vi "Laser_MAIN.vi"() -> ()   [LabVIEW 2013]
doc: "Пограмма управления мишенью лазерного источника ионов."
uses:
  <vilib>/Utility/miscctls.llb/LVPositionTypeDef.ctl
  <vilib>/Utility/inputDevices.llb/closeMouse.vi
panel:
  out "Текущая мишень:":string
  out "Флаг резерв. сохр.":bool
  in  "Шаг \nручного \nсдвига":string(combo)="5" caption="Шаг"
  in  "RightButton":bool
  in  "LeftButton":bool
  in  "DownButton":bool
  in  "UpButton":bool
  in  "М3":T1
  out "Знак перех. dX М10":i8
  out "Выстрелов осталось M10":u16=3
  in  "М10":T1
  in  "выстрел X М10":u16 step=1
  in  "выстрел Y М10":u16 step=1
  out "Знак перех. dX М9":i8
  out "Выстрелов осталось M9":u16=3
  in  "М9":T1
  in  "выстрел X М9":u16 step=1
  in  "выстрел Y М9":u16 step=1
  out "Выстрелов осталось M8":u16=3
  out "Знак перех. dX М8":i8
  in  "М8":T1
  in  "выстрел X М8":u16 step=1
  in  "выстрел Y М8":u16 step=1
  out "Выстрелов осталось M7":u16=3
  out "Знак перех. dX М7":i8
  in  "М7":T1
  in  "выстрел X М7":u16 step=1
  in  "выстрел Y М7":u16 step=1
  out "Выстрелов осталось M6":u16=3
  out "Знак перех. dX М6":i8
  in  "М6":T1
  in  "выстрел X М6":u16 step=1
  in  "выстрел Y М6":u16 step=1
  out "Выстрелов осталось M5":u16=3
  in  "М2":T1
  in  "М5":T1
  out "Знак перех. dX М5":i8
  in  "выстрел Y М5":u16 step=1
  in  "выстрел X М5":u16 step=1
  in  "М4":T1
  out "Знак перех. dX М4":i8
  in  "выстрел Y М4":u16 step=1
  in  "выстрел X М4":u16 step=1
  out "Знак перех. dX М3":i8
  in  "выстрел Y М3":u16 step=1
  in  "выстрел X М3":u16 step=1
  out "Знак перех. dX М2":i8
  in  "выстрел Y М2":u16 step=1
  in  "выстрел X М2":u16 step=1
  in  "выстрел Y М1":u16 step=1
  in  "выстрел X М1":u16 step=1
  out "Знак перех. dX М1":i8
  in  "М1":T1
  out "Выстрелов осталось M4":u16=3
  out "Выстрелов осталось M3":u16=3
  out "Выстрелов осталось M2":u16=3
  out "Выстрелов осталось M1":u16=3
  out "Статус":bool=TRUE caption="Готов!"
  in  "Tab control":T2(tab)
  in  "Перемотка пленки":bool
  in  "Фокус --":bool
  in  "Фокус +":bool
  in  "Сбросить конфигурацию":bool
  in  "Шаг вперед":bool
  in  "XY лазера":bool caption="осталось: 1"
  in  "текущ. инфо":bool caption="4"
  out "флаг закрытия с сохр.":bool
  in  "Загрузить настройки":bool
  in  "Конфигурация сохранена":bool
  in  "Мишень 10":picture
  in  "Мишень 9":picture
  in  "Мишень 8":picture
  in  "Мишень 7":picture
  in  "Мишень 6":picture
  in  "Упр. звуком":bool
  in  "Мишень 5":picture
  in  "Мишень 4":picture
  in  "Мишень 3":picture
  in  "Добавить мишень":bool
  in  "Мишень 2":picture
  in  "Мишень 1":picture
  in  "Выстрелов до перемотки пленки":u16=100
  out "Осталось:":u16(slide)=3 scale=100.0..1.0
  out "id мишени":u16=1
  in  "Счетчик выстрелов:":u32
  in  "TCP read data":string
  out "Slide X axis":u8(slide) max=100 scale=0.0..100.0
  out "Slide Y axis":u8(slide) max=50 step=1
  in  "Снимок сохранен":bool
  out "con err":bool caption="Connect"
  in  "Выстрел по мишени!":u32
  out "Счетчик мишеней":u8=3
  out "Соединение с блоком":bool
  out "Флаг соединения с прибором":bool caption="Connect"
  in  "OpLog":string
  in  "порт":u16=10001
  in  "IP-адрес":string="172.16.21.200"
  in  "Disconnect":bool caption="Disconn"
  out "Соединение":bool
  in  "Connect":bool
  out "TCP error source":string
  in  "stop":bool
  out "code out":i32 format="%0.0f"
  out "read_error_indicator":bool
  in  "Connect 2":bool caption="Connect"
  in  "flag1":bool caption="Disconn"
  out "TCP con ID":refnum<k5>
  out "Текущая конфигурация:":path
  out "Con.err.text":bool caption="Ошибка соединения с блоком..."
  # "Ручное управление \nлазером в пределах \nвыбранной мишени"
  # "Шаг перехода по Y, мм"
  # "Доп. настройки"
  # "Файлы"
  # "Мишени"
  # "Задано:"
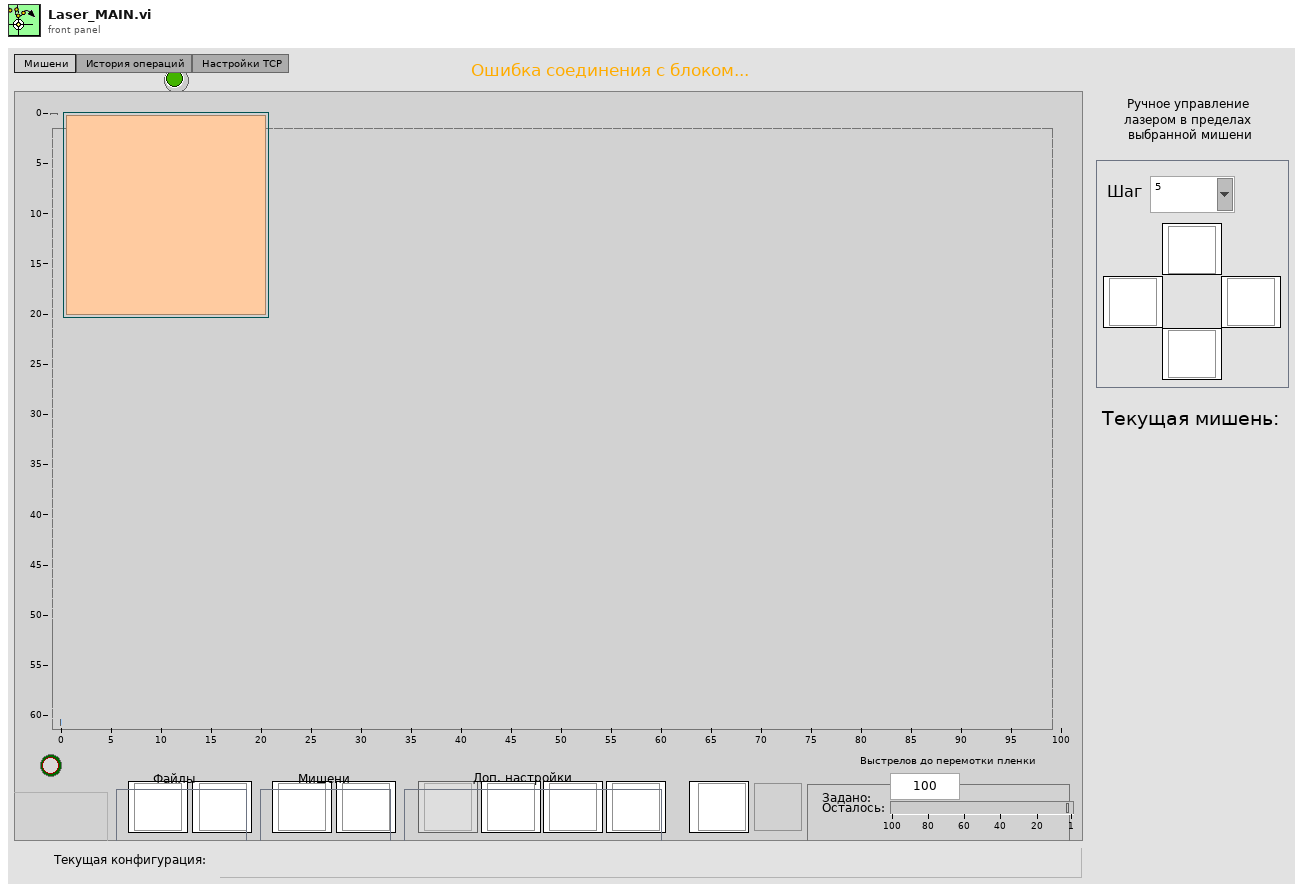
[diagram p1: front panel]
types:
  T1 = cluster{"Название мишени":string, "Х0_position":u16, "Y0_position":u16, "Длина, мм":u16, "Ширина, мм":u16, "Шаг перехода по горизонтали":dbl, "Шаг перехода по вертикали":dbl, "Выстрелов до перехода":u16, "Xo to send ":u16, "Yo to send":u16}
  T2 = enum32{" Мишени", " История операций", " Настройки TCP"}
  T3 = enum8{"Enabled", "Disabled", "Disabled and Grayed Out"}
  T4 = typedef "LVPositionTypeDef.ctl" = cluster{"Left":i32, "Top":i32}
  T5 = typedef "imagedata.ctl" = cluster{"image type":i32, "image depth":i32, "image":u8[], "mask":u8[], "colors":u32[], "Rectangle":cluster{"left":i16, "top":i16, "right":i16, "bottom":i16}}
  T6 = cluster{"id команды":u8, "№ мишени":u8, "Коорд. выстрела X ст.байт":u8, "Коорд. выстрела X мл.байт":u8, "Коорд. выстрела Y cт.байт":u8, "Коорд. выстрела Y мл.байт":u8, "Знак dX":i8, "выст. до перех. cт. байт":u8, "выст. до перех. мл. байт":u8, "выст. до перем. пленки ст. байт":u8, "выст. до перем. пленки мл. байт":u8}
  T7 = cluster{"номер мишени (id)":u8, u8, u8, u8, u8, u8, u8, u8, u8, u8, u8, u8, u8, u8, u8, u8, u8, u8, u8, u8}
  T8 = cluster{"доп команда":u8, u8, u8, u8, u8, u8, u8, u8, u8, u8, u8, u8, u8, u8, u8, u8, u8, u8, u8, u8}
  T9 = cluster{"М1":cluster{"Название мишени":string, "Х0_position":u16, "Y0_position":u16, "Длина, мм":u16, "Ширина, мм":u16, "Шаг перехода по горизонтали":dbl, "Шаг перехода по вертикали":dbl, "Выстрелов до перехода":u16, "Xo to send ":u16, "Yo to send":u16}, "М2":cluster{"Название мишени":string, "Х0_position":u16, "Y0_position":u16, "Длина, мм":u16, "Ширина, мм":u16, "Шаг перехода по горизонтали":dbl, "Шаг перехода по вертикали":dbl, "Выстрелов до перехода":u16, "Xo to send ":u16, "Yo to send":u16}, "М3":cluster{"Название мишени":string, "Х0_position":u16, "Y0_position":u16, "Длина, мм":u16, "Ширина, мм":u16, "Шаг перехода по горизонтали":dbl, "Шаг перехода по вертикали":dbl, "Выстрелов до перехода":u16, "Xo to send ":u16, "Yo to send":u16}, "М4":cluster{"Название мишени":string, "Х0_position":u16, "Y0_position":u16, "Длина, мм":u16, "Ширина, мм":u16, "Шаг перехода по горизонтали":dbl, "Шаг перехода по вертикали":dbl, "Выстрелов до перехода":u16, "Xo to send ":u16, "Yo to send":u16}, "М5":cluster{"Название мишени":string, "Х0_position":u16, "Y0_position":u16, "Длина, мм":u16, "Ширина, мм":u16, "Шаг перехода по горизонтали":dbl, "Шаг перехода по вертикали":dbl, "Выстрелов до перехода":u16, "Xo to send ":u16, "Yo to send":u16}, "М6":cluster{"Название мишени":string, "Х0_position":u16, "Y0_position":u16, "Длина, мм":u16, "Ширина, мм":u16, "Шаг перехода по горизонтали":dbl, "Шаг перехода по вертикали":dbl, "Выстрелов до перехода":u16, "Xo to send ":u16, "Yo to send":u16}, "М7":cluster{"Название мишени":string, "Х0_position":u16, "Y0_position":u16, "Длина, мм":u16, "Ширина, мм":u16, "Шаг перехода по горизонтали":dbl, "Шаг перехода по вертикали":dbl, "Выстрелов до перехода":u16, "Xo to send ":u16, "Yo to send":u16}, "М8":cluster{"Название мишени":string, "Х0_position":u16, "Y0_position":u16, "Длина, мм":u16, "Ширина, мм":u16, "Шаг перехода по горизонтали":dbl, "Шаг перехода по вертикали":dbl, "Выстрелов до перехода":u16, "Xo to send ":u16, "Yo to send":u16}, "М9":cluster{"Название мишени":string, "Х0_position":u16, "Y0_position":u16, "Длина, мм":u16, "Ширина, мм":u16, "Шаг перехода по горизонтали":dbl, "Шаг перехода по вертикали":dbl, "Выстрелов до перехода":u16, "Xo to send ":u16, "Yo to send":u16}, "М10":cluster{"Название мишени":string, "Х0_position":u16, "Y0_position":u16, "Длина, мм":u16, "Ширина, мм":u16, "Шаг перехода по горизонтали":dbl, "Шаг перехода по вертикали":dbl, "Выстрелов до перехода":u16, "Xo to send ":u16, "Yo to send":u16}}
  T10 = cluster{"выстрел X М1":u16, "выстрел Y М1":u16, "выстрел X М2":u16, "выстрел Y М2":u16, "выстрел X М3":u16, "выстрел Y М3":u16, "выстрел X М4":u16, "выстрел Y М4":u16, "выстрел X М5":u16, "выстрел Y М5":u16}
  T11 = cluster{"выстрел X М6":u16, "выстрел Y М6":u16, "выстрел X М7":u16, "выстрел Y М7":u16, "выстрел X М8":u16, "выстрел Y М8":u16, "выстрел X М9":u16, "выстрел Y М9":u16, "выстрел X М10":u16, "выстрел Y М10":u16}
  T12 = cluster{"Знак перех. dX М1":i8, "Знак перех. dX М2":i8, "Знак перех. dX М3":i8, "Знак перех. dX М4":i8, "Знак перех. dX М5":i8, "Знак перех. dX М6":i8, "Знак перех. dX М7":i8, "Знак перех. dX М8":i8, "Знак перех. dX М9":i8, "Знак перех. dX М10":i8}
  T13 = cluster{"Мишень 1":picture, "Мишень 2":picture, "Мишень 3":picture, "Мишень 4":picture, "Мишень 5":picture, "Мишень 6":picture, "Мишень 7":picture, "Мишень 8":picture, "Мишень 9":picture, "Мишень 10":picture}
  T14 = cluster{"Visible":bool, "Visible":bool, "Visible":bool, "Visible":bool, "Visible":bool, "Visible":bool, "Visible":bool, "Visible":bool, "Visible":bool, "Visible":bool}
  T15 = cluster{"Выстрелов осталось M1 ":u16, "Выстрелов осталось M2":u16, "Выстрелов осталось M3":u16, "Выстрелов осталось M4":u16, "Выстрелов осталось M5":u16, "Выстрелов осталось M6":u16, "Выстрелов осталось M7":u16, "Выстрелов осталось M8":u16, "Выстрелов осталось M9":u16, "Выстрелов осталось M10":u16}
  T16 = cluster{"Счетчик мишеней":u32, "Счетчик мишеней":u32}
  T17 = cluster{"Счетчик мишеней":i32, "Счетчик мишеней":i32}
  T18 = cluster{"Мишень 1":refnum<vi>, "Мишень 2":refnum<vi>, "Мишень 3":refnum<vi>, "Мишень 4":refnum<vi>, "Мишень 5":refnum<vi>, "Мишень 6":refnum<vi>, "Мишень 7":refnum<vi>, "Мишень 8":refnum<vi>, "Мишень 9":refnum<vi>, "Мишень 10":refnum<vi>}
  T19 = cluster{"Pict Refnum":refnum<vi>, "Pict Refnum 2":refnum<vi>, "Pict Refnum 3":refnum<vi>, "Pict Refnum 4":refnum<vi>, "Pict Refnum 5":refnum<vi>, "Pict Refnum 6":refnum<vi>, "Pict Refnum 7":refnum<vi>, "Pict Refnum 8":refnum<vi>, "Picture in Refnum 9":refnum<vi>, "Pict Refnum 10":refnum<vi>}
  T20 = cluster{"1":u16, "2":u16, "3":u16, "4":u16, "5":u16, "6":u16, "7":u16, "8":u16, "9":u16, "10":u16}
  T21 = cluster{"default value 1":i8, "default value 1":i8, "default value 1":i8, "default value 1":i8, "default value 1":i8, "default value 1":i8, "default value 1":i8, "default value 1":i8, "default value 1":i8, "default value 1":i8}
  T22 = cluster{"Кластер параметров мишени":cluster{"Название мишени":string, "Х0_position":u16, "Y0_position":u16, "Длина, мм":u16, "Ширина, мм":u16, "Шаг перехода по горизонтали":dbl, "Шаг перехода по вертикали":dbl, "Выстрелов до перехода":u16, "Xo to send ":u16, "Yo to send":u16}, "Кластер параметров мишени":cluster{"Название мишени":string, "Х0_position":u16, "Y0_position":u16, "Длина, мм":u16, "Ширина, мм":u16, "Шаг перехода по горизонтали":dbl, "Шаг перехода по вертикали":dbl, "Выстрелов до перехода":u16, "Xo to send ":u16, "Yo to send":u16}, "Кластер параметров мишени":cluster{"Название мишени":string, "Х0_position":u16, "Y0_position":u16, "Длина, мм":u16, "Ширина, мм":u16, "Шаг перехода по горизонтали":dbl, "Шаг перехода по вертикали":dbl, "Выстрелов до перехода":u16, "Xo to send ":u16, "Yo to send":u16}, "Кластер параметров мишени":cluster{"Название мишени":string, "Х0_position":u16, "Y0_position":u16, "Длина, мм":u16, "Ширина, мм":u16, "Шаг перехода по горизонтали":dbl, "Шаг перехода по вертикали":dbl, "Выстрелов до перехода":u16, "Xo to send ":u16, "Yo to send":u16}, "Кластер параметров мишени":cluster{"Название мишени":string, "Х0_position":u16, "Y0_position":u16, "Длина, мм":u16, "Ширина, мм":u16, "Шаг перехода по горизонтали":dbl, "Шаг перехода по вертикали":dbl, "Выстрелов до перехода":u16, "Xo to send ":u16, "Yo to send":u16}, "Кластер параметров мишени":cluster{"Название мишени":string, "Х0_position":u16, "Y0_position":u16, "Длина, мм":u16, "Ширина, мм":u16, "Шаг перехода по горизонтали":dbl, "Шаг перехода по вертикали":dbl, "Выстрелов до перехода":u16, "Xo to send ":u16, "Yo to send":u16}, "Кластер параметров мишени":cluster{"Название мишени":string, "Х0_position":u16, "Y0_position":u16, "Длина, мм":u16, "Ширина, мм":u16, "Шаг перехода по горизонтали":dbl, "Шаг перехода по вертикали":dbl, "Выстрелов до перехода":u16, "Xo to send ":u16, "Yo to send":u16}, "Кластер параметров мишени":cluster{"Название мишени":string, "Х0_position":u16, "Y0_position":u16, "Длина, мм":u16, "Ширина, мм":u16, "Шаг перехода по горизонтали":dbl, "Шаг перехода по вертикали":dbl, "Выстрелов до перехода":u16, "Xo to send ":u16, "Yo to send":u16}, "Кластер параметров мишени":cluster{"Название мишени":string, "Х0_position":u16, "Y0_position":u16, "Длина, мм":u16, "Ширина, мм":u16, "Шаг перехода по горизонтали":dbl, "Шаг перехода по вертикали":dbl, "Выстрелов до перехода":u16, "Xo to send ":u16, "Yo to send":u16}, "Кластер параметров мишени":cluster{"Название мишени":string, "Х0_position":u16, "Y0_position":u16, "Длина, мм":u16, "Ширина, мм":u16, "Шаг перехода по горизонтали":dbl, "Шаг перехода по вертикали":dbl, "Выстрелов до перехода":u16, "Xo to send ":u16, "Yo to send":u16}}
  T23 = enum16{"Left Button", "Center Button", "Right Button", "Window Close"}
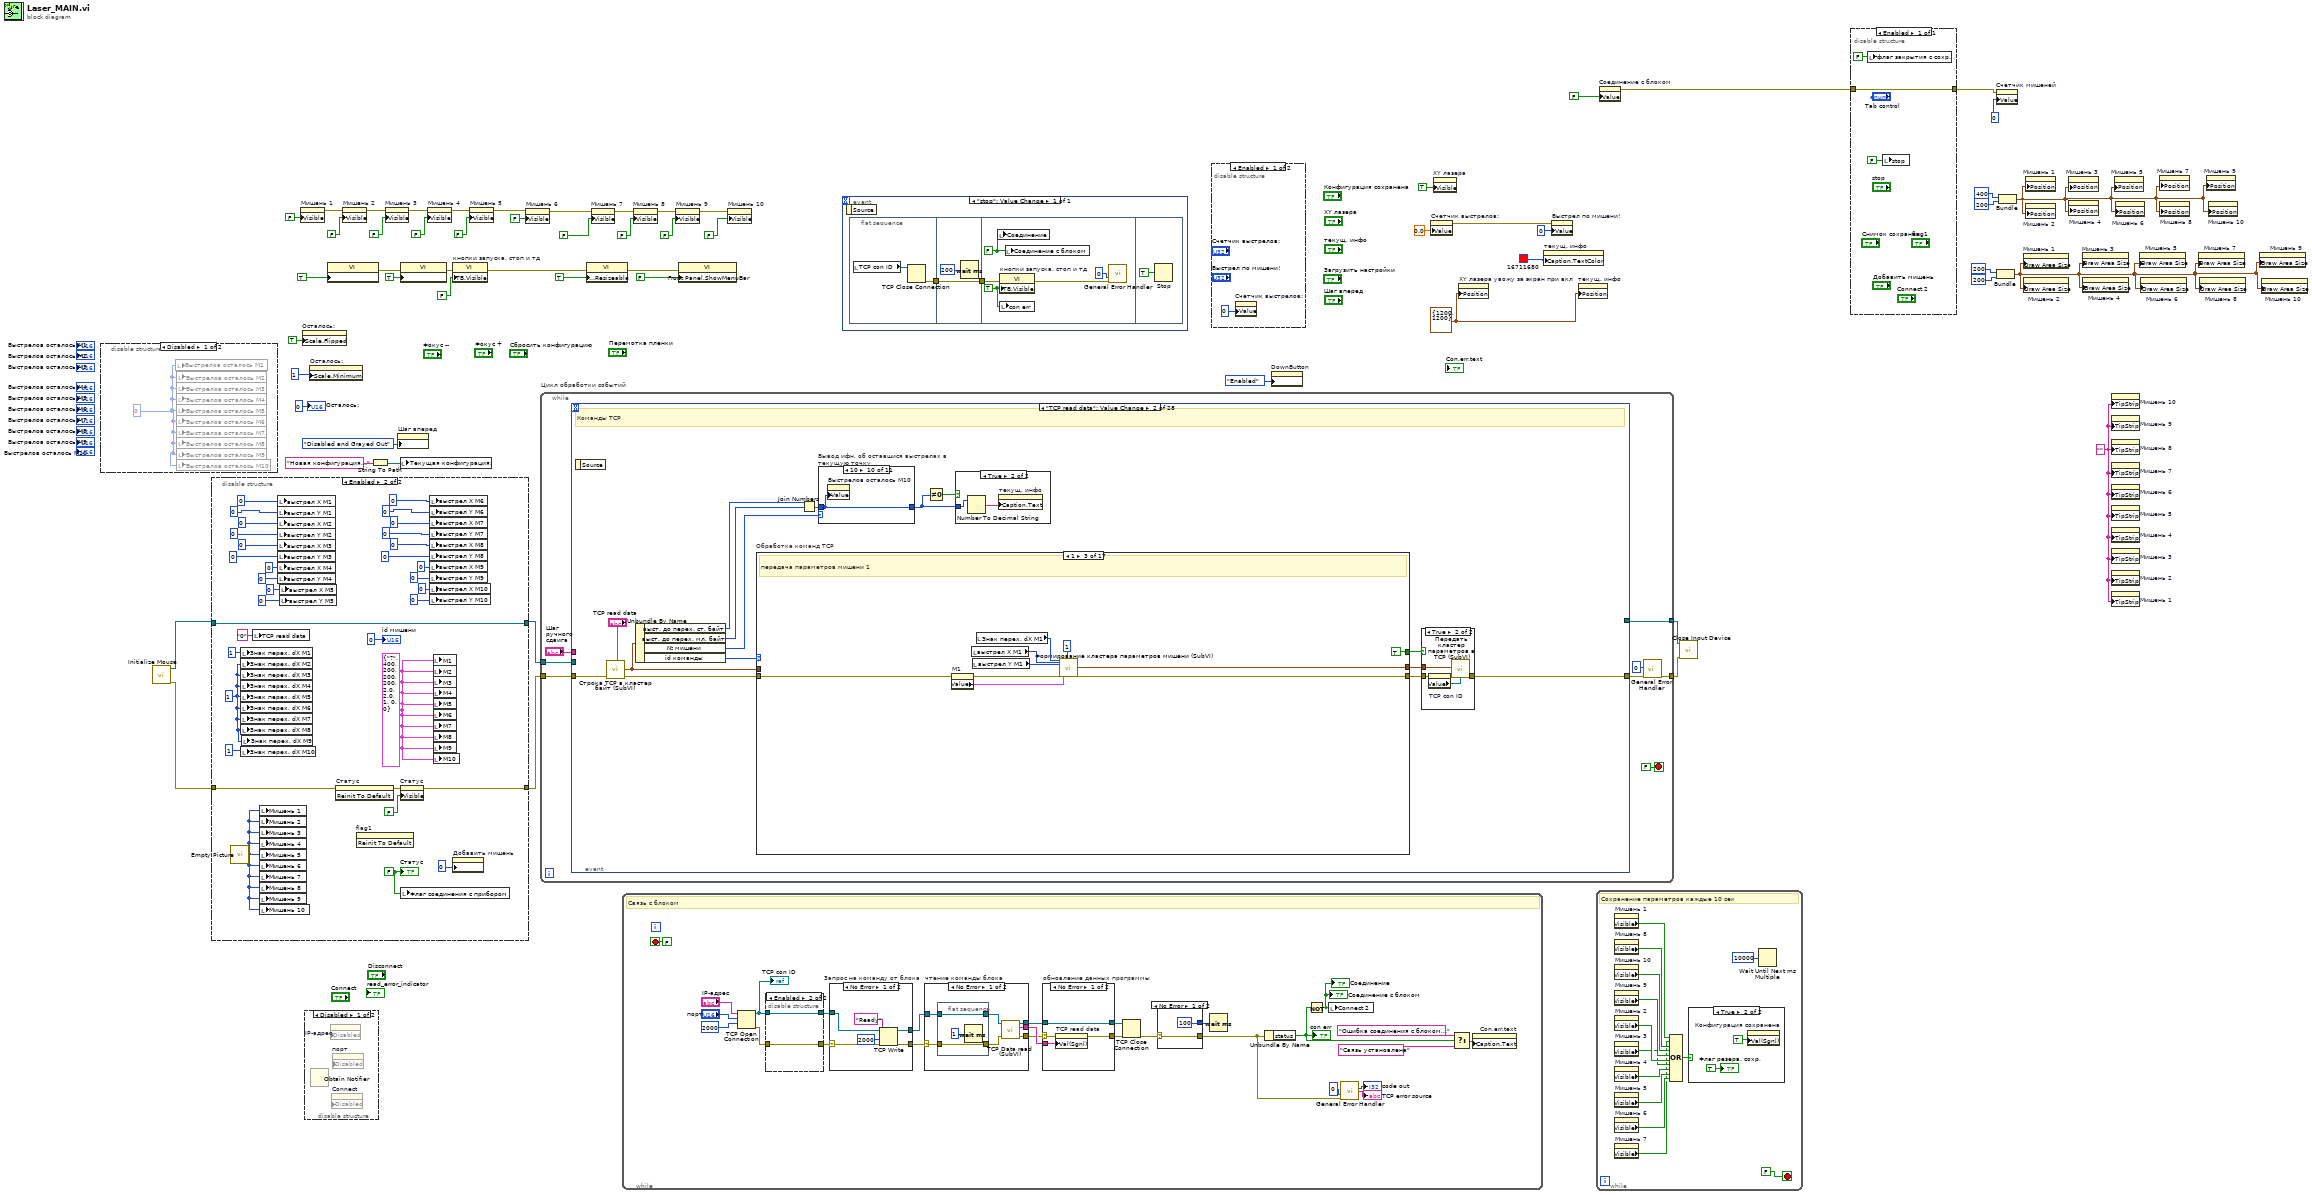
[diagram p0: block diagram]
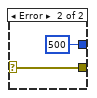
[diagram p5: hidden frame]
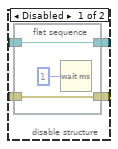
[diagram p6: hidden frame]
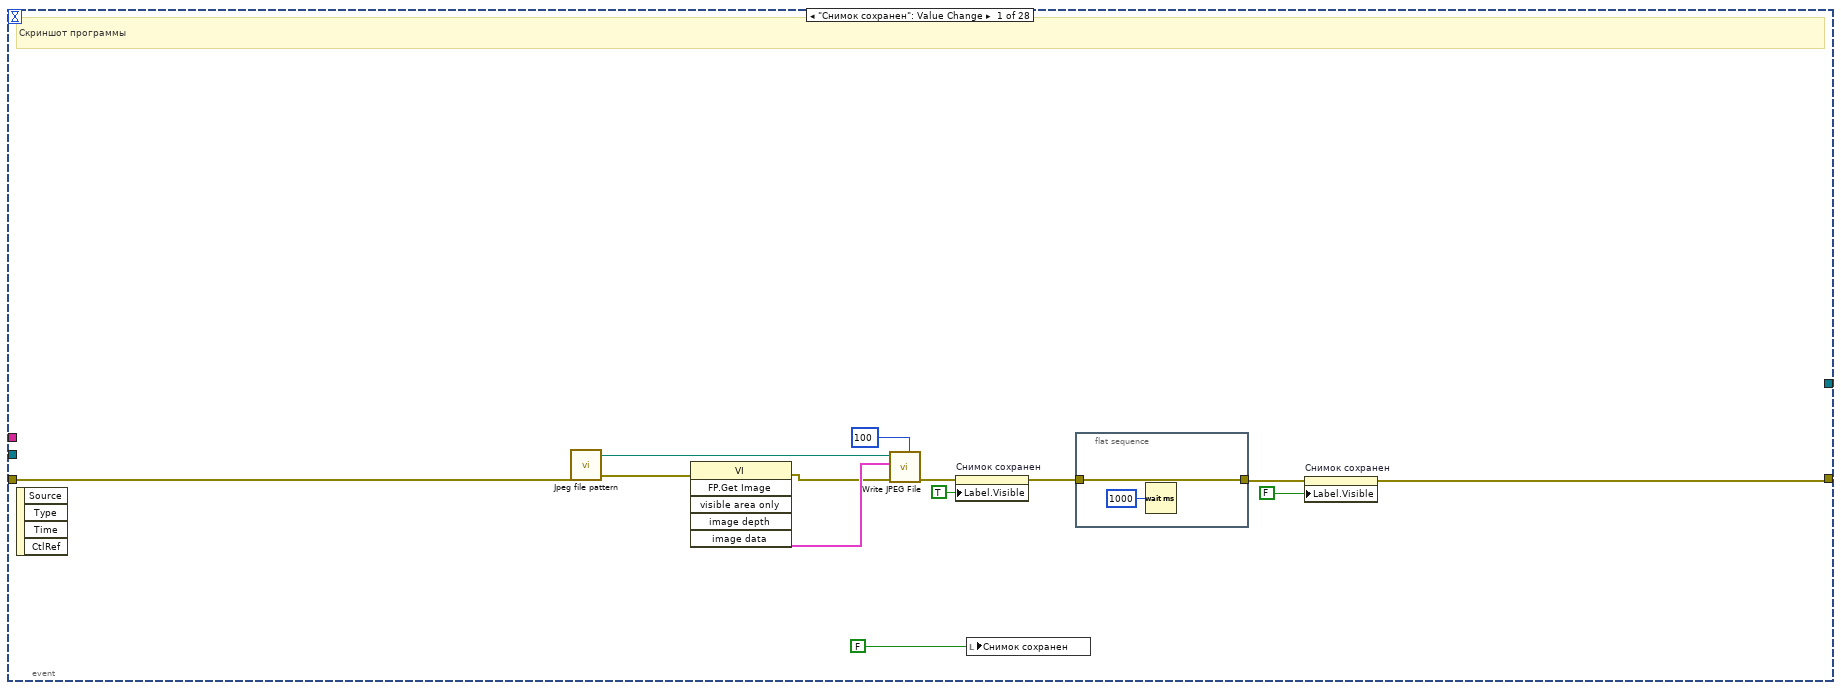
[diagram p12: hidden frame]
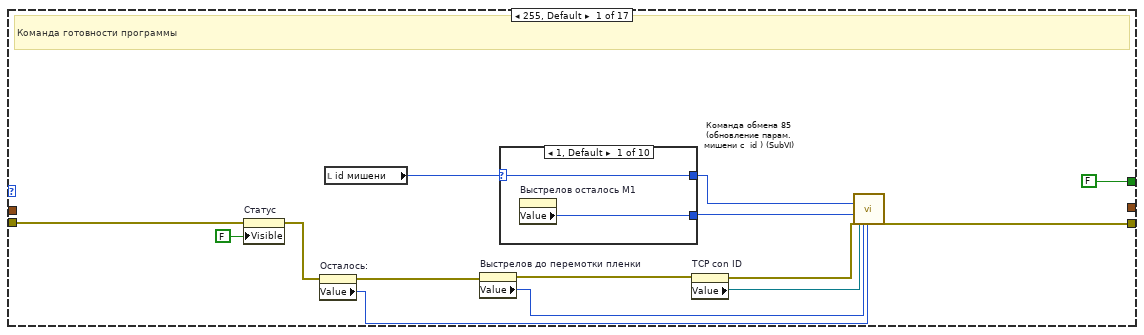
[diagram p15: hidden frame]
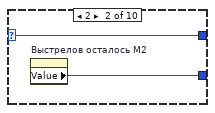
[diagram p16: hidden frame]
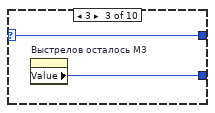
[diagram p17: hidden frame]
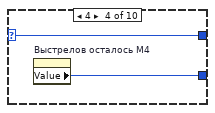
[diagram p18: hidden frame]
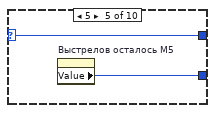
[diagram p19: hidden frame]
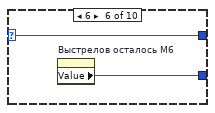
[diagram p20: hidden frame]
diagram:
  w8 = "" ("Tip Strip")
  w49 = T4 {"Left"=1200, "Top"=1200} ("Position")
  n1 = disable-structure shown="Disabled" {
    frame Disabled {
      w59 = u16 0
      n2 = local write "Выстрелов осталось M1"(w59) -> ()
      n3 = local write "Выстрелов осталось M2"(w59) -> ()
      n4 = local write "Выстрелов осталось M3"(w59) -> ()
      n5 = local write "Выстрелов осталось M4"(w59) -> ()
      n6 = local write "Выстрелов осталось M5"(w59) -> ()
      n7 = local write "Выстрелов осталось M6"(w59) -> ()
      n8 = local write "Выстрелов осталось M7"(w59) -> ()
      n9 = local write "Выстрелов осталось M8"(w59) -> ()
      n10 = local write "Выстрелов осталось M9"(w59) -> ()
      n11 = local write "Выстрелов осталось M10"(w59) -> ()
    }
    frame Enabled {
    }
  }
  n12 = call <vilib>:"Initialize Mouse.vi"() -> ("error out"=w51:errorcluster, "device ID"=w53:refnum<k1>)  [unwired: 1 in, 9 out]
  n13 = disable-structure shown="Enabled" {
    disable-tunnel: [_ w93] -> w54
    disable-tunnel: w53 -> [_ w93]
    disable-tunnel: [_ w64] -> w52
    disable-tunnel: w51 -> [_ w92]
    frame Disabled {
    }
    frame Enabled {
      w88 = i8 1 ("Выстрелов осталось M1")
      w89 = T1 {"Название мишени"="?", "Х0_position"=400, "Y0_position"=200, "Длина, мм"=200, "Ширина, мм"=200, "Шаг перехода по горизонтали"=2.0, "Шаг перехода по вертикали"=2.0, "Выстрелов до перехода"=1, "Xo to send "=0, "Yo to send"=0} ("Параметры М1")
      w61 = FALSE ("Готов")
      n14 = call "Empty Picture"() -> ("empty picture"=w65:picture)
      n15 = local write "Знак перех. dX М1"(i8 1 ("Знак перех. dX М1")) -> ()
      n16 = local write "Знак перех. dX М2"(w88) -> ()
      n17 = local write "Знак перех. dX М3"(w88) -> ()
      n18 = local write "Знак перех. dX М4"(w88) -> ()
      n19 = local write "Знак перех. dX М5"(w88) -> ()
      n20 = local write "Знак перех. dX М6"(w88) -> ()
      n21 = local write "Знак перех. dX М7"(w88) -> ()
      n22 = local write "Знак перех. dX М8"(w88) -> ()
      n23 = local write "Знак перех. dX М10"(i8 1 ("Выстрелов осталось M1")) -> ()
      n24 = local write "Знак перех. dX М9"(w88) -> ()
      n25 = local write "TCP read data"("0" ("TCP read data")) -> ()
      n26 = local write "Мишень 1"(w65) -> ()
      n27 = local write "Мишень 2"(w65) -> ()
      n28 = local write "Мишень 3"(w65) -> ()
      n29 = local write "Мишень 4"(w65) -> ()
      n30 = local write "Мишень 5"(w65) -> ()
      n31 = local write "Мишень 6"(w65) -> ()
      n32 = local write "Мишень 7"(w65) -> ()
      n33 = local write "Мишень 8"(w65) -> ()
      n34 = local write "Мишень 9"(w65) -> ()
      n35 = local write "Мишень 10"(w65) -> ()
      n36 = local write "выстрел X М1"(u16 0 ("Выстрелов осталось M1")) -> ()
      n37 = local write "выстрел Y М1"(u16 0 ("Выстрелов осталось M2")) -> ()
      n38 = local write "выстрел X М2"(u16 0 ("Выстрелов осталось M3")) -> ()
      n39 = local write "выстрел Y М2"(u16 0 ("Выстрелов осталось M4")) -> ()
      n40 = local write "выстрел X М3"(u16 0 ("Выстрелов осталось M5")) -> ()
      n41 = local write "выстрел Y М3"(u16 0 ("Выстрелов осталось M6")) -> ()
      n42 = local write "выстрел X М4"(u16 0 ("выстрел X М9")) -> ()
      n43 = local write "выстрел Y М4"(u16 0 ("выстрел Y М9")) -> ()
      n44 = local write "выстрел X М5"(u16 0 ("выстрел X М10")) -> ()
      n45 = local write "выстрел Y М5"(u16 0 ("выстрел Y М10")) -> ()
      n46 = invoke on="Статус" class="Bool (strict)" method="Reinit To Default"(error in=w92) -> (error out=w90:errorcluster)  [unwired: 2 in, 2 out]
      n47 = invoke on="flag1" class="Bool (strict)" method="Reinit To Default"() -> ()  [unwired: 3 in, 3 out]
      n48 = property on="Статус" class="Bool (strict)"(error in=w90, "Visible"=FALSE) -> (error out=w64:errorcluster)  [unwired: 1 in, 1 out]
      n49 = local write "Флаг соединения с прибором"(w61) -> ()
      n50 = local write "выстрел X М6"(u16 0 ("Выстрелов осталось M1")) -> ()
      n51 = local write "выстрел Y М6"(u16 0 ("Выстрелов осталось M2")) -> ()
      n52 = local write "выстрел X М7"(u16 0 ("Выстрелов осталось M3")) -> ()
      n53 = local write "выстрел Y М7"(u16 0 ("Выстрелов осталось M4")) -> ()
      n54 = local write "выстрел X М8"(u16 0 ("Выстрелов осталось M5")) -> ()
      n55 = local write "выстрел Y М8"(u16 0 ("Выстрелов осталось M6")) -> ()
      n56 = local write "выстрел X М9"(u16 0 ("выстрел X М9")) -> ()
      n57 = local write "выстрел Y М9"(u16 0 ("выстрел Y М9")) -> ()
      n58 = local write "выстрел X М10"(u16 0 ("выстрел X М10")) -> ()
      n59 = local write "выстрел Y М10"(u16 0 ("выстрел Y М10")) -> ()
      n60 = local write "М1"(w89) -> ()
      n61 = local write "М2"(w89) -> ()
      n62 = local write "М3"(w89) -> ()
      n63 = local write "М4"(w89) -> ()
      n64 = local write "М5"(w89) -> ()
      n65 = local write "М6"(w89) -> ()
      n66 = local write "М7"(w89) -> ()
      n67 = local write "М8"(w89) -> ()
      n68 = local write "М9"(w89) -> ()
      n69 = local write "М10"(w89) -> ()
      n70 = property on="Добавить мишень" class="Bool (strict)"("DisabledEnum"=i8 0 ("Выстрелов осталось M1")) -> ()  [unwired: 2 in, 2 out]
      "Статус" <- w61
      "id мишени" <- u16 0 ("id мишени")
    }
  }
  n71 = property on="Мишень 1" class="Pict"("Visible"=FALSE) -> (error out=w35:errorcluster)  [unwired: 2 in, 1 out]
  n72 = property on="Осталось:" class="Slide (strict)"("Scale.Flipped"=TRUE) -> ()  [unwired: 2 in, 2 out]
  n73 = disable-structure shown="Disabled" {
    frame Disabled {
      n74 = Obtain Notifier() -> ()  [unwired: 4 in, 3 out]
      n75 = property on="IP-адрес" class="Str" props=["Disabled"]() -> ()  [unwired: 3 in, 2 out]
      n76 = property on="Connect" class="Bool (strict)" props=["Disabled"]() -> ()  [unwired: 3 in, 2 out]
      n77 = property on="порт" class="DigNum (strict)" props=["Disabled"]() -> ()  [unwired: 3 in, 2 out]
    }
    frame Enabled {
    }
  }
  n78 = property on="Осталось:" class="Slide (strict)"("Scale.Minimum"=u16 1 ("До перемотки осталось")) -> ()  [unwired: 2 in, 2 out]
  n79 = property class="VI"("Front Panel.Minimizeable"=TRUE ("Front Panel Window:Minimizable")) -> (error out=w41:errorcluster)  [unwired: 2 in, 1 out]
  n80 = property on="Мишень 2" class="Pict"(error in=w35, "Visible"=FALSE) -> (error out=w32:errorcluster)  [unwired: 1 in, 1 out]
  n81 = String To Path(string="Новая конфигурация...") -> (path=w7:path)
  n82 = property on="Мишень 3" class="Pict"(error in=w32, "Visible"=FALSE) -> (error out=w30:errorcluster)  [unwired: 1 in, 1 out]
  n83 = property on="Шаг вперед" class="Bool (strict)"("DisabledEnum"=T3."Disabled and Grayed Out" ("Disabled")) -> ()  [unwired: 2 in, 2 out]
  n84 = property class="VI"(error in=w41, "Front Panel.TitleBarVis"=TRUE ("Front Panel Window:Title Bar Visible")) -> (error out=w40:errorcluster)  [unwired: 1 in, 1 out]
  n85 = local write "Текущая конфигурация:"(w7) -> ()
  n86 = property on="Мишень 4" class="Pict"(error in=w30, "Visible"=FALSE) -> (error out=w28:errorcluster)  [unwired: 1 in, 1 out]
  n87 = property on="кнопки запуска, стоп и тд" class="VI"(error in=w40, "TB.Visible"=FALSE ("Tool Bar:Visible")) -> (error out=w39:errorcluster)  [unwired: 1 in, 1 out]
  n88 = property on="Мишень 5" class="Pict"(error in=w28, "Visible"=FALSE) -> (error out=w16:errorcluster)  [unwired: 1 in, 1 out]
  n89 = property on="Мишень 6" class="Pict"(error in=w16, "Visible"=FALSE) -> (error out=w17:errorcluster)  [unwired: 1 in, 1 out]
  n90 = while "Цикл обработки событий" {
    tunnel: w52 -> [w100]
    tunnel: w54 -> [w99]
    tunnel: [w96] -> w50
    tunnel: [w95] -> w48
    stop <- FALSE stop-if-true
    n91 = event shown="[1] \"TCP read data\": Value Change" {
      selector: _ -> [_ _ _ _ _ _ _ _ _ _ _ _ _ _ _ _ _ _ _ _ _ _ _ _ _ _ _ _]
      dyn-events: _ -> [_ _ _ _ _ _ _ _ _ _ _ _ _ _ _ _ _ _ _ _ _ _ _ _ _ _ _ _]
      timeout: _ -> [_ _ _ _ _ _ _ _ _ _ _ _ _ _ _ _ _ _ _ _ _ _ _ _ _ _ _ _]
      tunnel: [w102 w131 w689 w801 w816 w851 w878 w904 w930 w956 w982 w1008 w1034 w1060 w1086 w1120 w1153 w1159 w1163 w1168 w1184 w1223 w1280 w1328 w1366 _ w1547 _] -> w97
      tunnel: w100 -> [w110 w130 w695 w805 w815 w852 w877 w903 w929 w955 w981 w1007 w1033 w1059 w1085 w1113 w1154 w1162 w1167 w1172 w1176 w1226 w1274 w1322 w1367 _ w1552 _]
      tunnel: w99 -> [_ _ _ w806 _ _ _ _ _ _ _ _ _ _ _ _ _ _ _ _ _ _ _ _ _ _ _ _]
      tunnel: [_ _ _ w804 _ _ _ _ _ _ _ _ _ _ _ _ _ _ _ _ _ _ _ _ _ _ _ _] -> w95
      tunnel: "Шаг \nручного \nсдвига" -> [_ _ _ _ _ _ _ _ _ _ _ _ _ _ _ _ _ _ _ _ w1178 w1228 w1276 w1324 _ _ _ _]
      event "Снимок сохранен": Value Change {
        # "Скриншот программы"
        n92 = event-data() -> ()  [unwired: 5 out]
        n93 = call "Jpeg file pattern.vi"("error in"=w110) -> ("path to JPG file"=w111:path, "error out"=w109:errorcluster)  [unwired: 7 in]
        n94 = invoke class="VI" method="FP.Get Image"(error in=w109) -> (error out=w108:errorcluster, "image data"=w112:T5)  [unwired: 5 in, 4 out]
        n95 = call <vilib>:"Write JPEG File.vi"("quality (80)"=100, "error in (no error)"=w108, "image data"=w112, "path to JPEG file"=w111) -> ("error out"=w105:errorcluster)  [unwired: 7 out]
        n96 = property on="Снимок сохранен" class="Bool (strict)"(error in=w105, "Label.Visible"=TRUE) -> (error out=w103:errorcluster)  [unwired: 1 in, 1 out]
        n97 = local write "Снимок сохранен"(FALSE ("Снимок")) -> ()
        n98 = flat-sequence {
          tunnel: [w116] -> w104
          tunnel: w103 -> [w116]
          frame #0 {
            n99 = Wait (ms)(milliseconds to wait=u32 1000) -> ()  [unwired: 1 out]
          }
        }
        n100 = property on="Снимок сохранен" class="Bool (strict)"(error in=w104, "Label.Visible"=FALSE) -> (error out=w102:errorcluster)  [unwired: 1 in, 1 out]
      }
      event "TCP read data": Value Change {
        # "Команды TCP"
        n101 = event-data() -> ()  [unwired: 2 out]
        n102 = call "Строка TCP в кластер байт (SubVI).vi"("TCP read data"="TCP read data", "error in"=w130) -> ("Кластер прочитанных байт"=w127:T6, "error out"=w124:errorcluster)  [unwired: 12 in]
        n103 = Unbundle By Name(w127) -> ("выст. до перех. cт. байт"=w122:u8, "выст. до перех. мл. байт"=w121:u8, "№ мишени"=w120:u8, "id команды"=w128:u8)
        n104 = case "Обработка команд TCP" shown="1" w128 {
          tunnel: w127 -> [_ _ _ _ _ _ _ _ _ _ _ _ _ w308 w393 w537 _]
          tunnel: w124 -> [w151 w175 w183 w193 w203 w213 w223 w233 w243 w253 w263 w273 w280 w299 w404 w536 _]
          tunnel: [w150 w175 w186 w196 w206 w216 w226 w236 w246 w256 w266 w276 w279 w289 w392 w533 _] -> w126
          tunnel: [_ _ w178 w188 w198 w208 w218 w228 w238 w248 w258 w268 w278 _ _ _ _] -> w125
          tunnel: [FALSE FALSE TRUE TRUE TRUE TRUE TRUE TRUE TRUE TRUE TRUE TRUE FALSE FALSE FALSE FALSE _] -> w123
          frame 255, Default {
            # "Команда готовности программы"
            n105 = property on="Статус" class="Bool (strict)"(error in=w151, "Visible"=FALSE) -> (error out=w152:errorcluster)  [unwired: 1 in, 1 out]
            n106 = property on="Осталось:" class="Slide (strict)"(error in=w152) -> (error out=w147:errorcluster, "Value"=w145:u16)  [unwired: 1 in, 1 out]
            n107 = local read "id мишени"() -> (w148:u16)
            n108 = property on="Выстрелов до перемотки пленки" class="DigNum (strict)"(error in=w147) -> (error out=w146:errorcluster, "Value"=w144:u16)  [unwired: 1 in, 1 out]
            n109 = case shown="1, Default" w148 {
              selector: w148 -> [w154 w156 w158 w160 w162 w164 w166 w168 w170 w172]
              tunnel: [w155 w157 w159 w161 w163 w165 w167 w169 w171 w173] -> w141
              tunnel: [w154 w156 w158 w160 w162 w164 w166 w168 w170 w172] -> w140
              frame 1, Default {
                n110 = property on="Выстрелов осталось M1" class="DigNum (strict)"() -> ("Value"=w155:u16)  [unwired: 2 in, 2 out]
              }
              frame 2 {
                n111 = property on="Выстрелов осталось M2" class="DigNum (strict)"() -> ("Value"=w157:u16)  [unwired: 2 in, 2 out]
              }
              frame 3 {
                n112 = property on="Выстрелов осталось M3" class="DigNum (strict)"() -> ("Value"=w159:u16)  [unwired: 2 in, 2 out]
              }
              frame 4 {
                n113 = property on="Выстрелов осталось M4" class="DigNum (strict)"() -> ("Value"=w161:u16)  [unwired: 2 in, 2 out]
              }
              frame 5 {
                n114 = property on="Выстрелов осталось M5" class="DigNum (strict)"() -> ("Value"=w163:u16)  [unwired: 2 in, 2 out]
              }
              frame 6 {
                n115 = property on="Выстрелов осталось M6" class="DigNum (strict)"() -> ("Value"=w165:u16)  [unwired: 2 in, 2 out]
              }
              frame 7 {
                n116 = property on="Выстрелов осталось M7" class="DigNum (strict)"() -> ("Value"=w167:u16)  [unwired: 2 in, 2 out]
              }
              frame 8 {
                n117 = property on="Выстрелов осталось M8" class="DigNum (strict)"() -> ("Value"=w169:u16)  [unwired: 2 in, 2 out]
              }
              frame 9 {
                n118 = property on="Выстрелов осталось M9" class="DigNum (strict)"() -> ("Value"=w171:u16)  [unwired: 2 in, 2 out]
              }
              frame 10 {
                n119 = property on="Выстрелов осталось M10" class="DigNum (strict)"() -> ("Value"=w173:u16)  [unwired: 2 in, 2 out]
              }
            }
            n120 = property on="TCP con ID" class="Ref (strict)"(error in=w146) -> (error out=w143:errorcluster, "Value"=w142:refnum<k5>)  [unwired: 1 in, 1 out]
            n121 = call "Команда обмена 85 (обновление парам. мишени с  id ) (SubVI).vi"("id мишени"=w140, "Выстрелов осталось"=w141, "error in"=w143, "TCP connection ID"=w142, "Выстрелов до перемотки"=w144, "До перемотки осталось"=w145) -> ("error out"=w150:errorcluster)  [unwired: 21 in]
          }
          frame 254 {
            # "Команда анализа активного соединения с прибором"
            "Флаг соединения с прибором" <- TRUE ("Флаг соединения с прибором")
          }
          frame 1 {
            # "передача параметров мишени 1"
            n122 = property on="М1" class="Clust (strict)"(error in=w183) -> (error out=w185:errorcluster, "Value"=w184:T1)  [unwired: 1 in, 1 out]
            n123 = local read "выстрел X М1"() -> (w180:u16)
            n124 = local read "выстрел Y М1"() -> (w179:u16)
            n125 = local read "Знак перех. dX М1"() -> (w181:i8)
            n126 = call "Формирование кластера параметров мишени (SubVI).vi"("Знак перемещения Dx"=w181, "выстрел X мишени"=w180, "выстрел Y мишени"=w179, "error in (no error)"=w185, "Параметры Мишени"=w184, "номер мишени (id)"=u8 1) -> ("Кластер параметров мишени"=w178:T7, "error out"=w186:errorcluster)  [unwired: 20 in]
          }
          frame 2 {
            # "передача параметров мишени 2"
            n127 = property on="М2" class="Clust (strict)"(error in=w193) -> (error out=w195:errorcluster, "Value"=w194:T1)  [unwired: 1 in, 1 out]
            n128 = local read "выстрел X М2"() -> (w190:u16)
            n129 = local read "выстрел Y М2"() -> (w189:u16)
            n130 = local read "Знак перех. dX М2"() -> (w191:i8)
            n131 = call "Формирование кластера параметров мишени (SubVI).vi"("Знак перемещения Dx"=w191, "выстрел X мишени"=w190, "выстрел Y мишени"=w189, "error in (no error)"=w195, "Параметры Мишени"=w194, "номер мишени (id)"=u8 2) -> ("Кластер параметров мишени"=w188:T7, "error out"=w196:errorcluster)  [unwired: 20 in]
          }
          frame 3 {
            # "передача параметров мишени 3"
            n132 = property on="М3" class="Clust (strict)"(error in=w203) -> (error out=w205:errorcluster, "Value"=w204:T1)  [unwired: 1 in, 1 out]
            n133 = local read "выстрел X М3"() -> (w200:u16)
            n134 = local read "выстрел Y М3"() -> (w199:u16)
            n135 = local read "Знак перех. dX М3"() -> (w201:i8)
            n136 = call "Формирование кластера параметров мишени (SubVI).vi"("Знак перемещения Dx"=w201, "выстрел X мишени"=w200, "выстрел Y мишени"=w199, "error in (no error)"=w205, "Параметры Мишени"=w204, "номер мишени (id)"=u8 3) -> ("Кластер параметров мишени"=w198:T7, "error out"=w206:errorcluster)  [unwired: 20 in]
          }
          frame 4 {
            # "передача параметров мишени 4"
            n137 = property on="М4" class="Clust (strict)"(error in=w213) -> (error out=w215:errorcluster, "Value"=w214:T1)  [unwired: 1 in, 1 out]
            n138 = local read "выстрел X М4"() -> (w210:u16)
            n139 = local read "выстрел Y М4"() -> (w209:u16)
            n140 = local read "Знак перех. dX М4"() -> (w211:i8)
            n141 = call "Формирование кластера параметров мишени (SubVI).vi"("Знак перемещения Dx"=w211, "выстрел X мишени"=w210, "выстрел Y мишени"=w209, "error in (no error)"=w215, "Параметры Мишени"=w214, "номер мишени (id)"=u8 4) -> ("Кластер параметров мишени"=w208:T7, "error out"=w216:errorcluster)  [unwired: 20 in]
          }
          frame 5 {
            # "передача параметров мишени 5"
            n142 = property on="М5" class="Clust (strict)"(error in=w223) -> (error out=w225:errorcluster, "Value"=w224:T1)  [unwired: 1 in, 1 out]
            n143 = local read "выстрел X М5"() -> (w220:u16)
            n144 = local read "выстрел Y М5"() -> (w219:u16)
            n145 = local read "Знак перех. dX М5"() -> (w221:i8)
            n146 = call "Формирование кластера параметров мишени (SubVI).vi"("Знак перемещения Dx"=w221, "выстрел X мишени"=w220, "выстрел Y мишени"=w219, "error in (no error)"=w225, "Параметры Мишени"=w224, "номер мишени (id)"=u8 5) -> ("Кластер параметров мишени"=w218:T7, "error out"=w226:errorcluster)  [unwired: 20 in]
          }
          frame 6 {
            # "передача параметров мишени 6"
            n147 = property on="М6" class="Clust (strict)"(error in=w233) -> (error out=w235:errorcluster, "Value"=w234:T1)  [unwired: 1 in, 1 out]
            n148 = local read "выстрел X М6"() -> (w230:u16)
            n149 = local read "выстрел Y М6"() -> (w229:u16)
            n150 = local read "Знак перех. dX М6"() -> (w231:i8)
            n151 = call "Формирование кластера параметров мишени (SubVI).vi"("Знак перемещения Dx"=w231, "выстрел X мишени"=w230, "выстрел Y мишени"=w229, "error in (no error)"=w235, "Параметры Мишени"=w234, "номер мишени (id)"=u8 6) -> ("Кластер параметров мишени"=w228:T7, "error out"=w236:errorcluster)  [unwired: 20 in]
          }
          frame 7 {
            # "передача параметров мишени 7"
            n152 = property on="М7" class="Clust (strict)"(error in=w243) -> (error out=w245:errorcluster, "Value"=w244:T1)  [unwired: 1 in, 1 out]
            n153 = local read "выстрел X М7"() -> (w240:u16)
            n154 = local read "выстрел Y М7"() -> (w239:u16)
            n155 = local read "Знак перех. dX М7"() -> (w241:i8)
            n156 = call "Формирование кластера параметров мишени (SubVI).vi"("Знак перемещения Dx"=w241, "выстрел X мишени"=w240, "выстрел Y мишени"=w239, "error in (no error)"=w245, "Параметры Мишени"=w244, "номер мишени (id)"=u8 7) -> ("Кластер параметров мишени"=w238:T7, "error out"=w246:errorcluster)  [unwired: 20 in]
          }
          frame 8 {
            # "передача параметров мишени 8"
            n157 = property on="М8" class="Clust (strict)"(error in=w253) -> (error out=w255:errorcluster, "Value"=w254:T1)  [unwired: 1 in, 1 out]
            n158 = local read "выстрел X М8"() -> (w250:u16)
            n159 = local read "выстрел Y М8"() -> (w249:u16)
            n160 = local read "Знак перех. dX М8"() -> (w251:i8)
            n161 = call "Формирование кластера параметров мишени (SubVI).vi"("Знак перемещения Dx"=w251, "выстрел X мишени"=w250, "выстрел Y мишени"=w249, "error in (no error)"=w255, "Параметры Мишени"=w254, "номер мишени (id)"=u8 8) -> ("Кластер параметров мишени"=w248:T7, "error out"=w256:errorcluster)  [unwired: 20 in]
          }
          frame 9 {
            # "передача параметров мишени 9"
            n162 = property on="М9" class="Clust (strict)"(error in=w263) -> (error out=w265:errorcluster, "Value"=w264:T1)  [unwired: 1 in, 1 out]
            n163 = local read "выстрел X М9"() -> (w260:u16)
            n164 = local read "выстрел Y М9"() -> (w259:u16)
            n165 = local read "Знак перех. dX М9"() -> (w261:i8)
            n166 = call "Формирование кластера параметров мишени (SubVI).vi"("Знак перемещения Dx"=w261, "выстрел X мишени"=w260, "выстрел Y мишени"=w259, "error in (no error)"=w265, "Параметры Мишени"=w264, "номер мишени (id)"=u8 9) -> ("Кластер параметров мишени"=w258:T7, "error out"=w266:errorcluster)  [unwired: 20 in]
          }
          frame 10 {
            # "передача параметров мишени 10"
            n167 = property on="М10" class="Clust (strict)"(error in=w273) -> (error out=w275:errorcluster, "Value"=w274:T1)  [unwired: 1 in, 1 out]
            n168 = local read "выстрел X М10"() -> (w270:u16)
            n169 = local read "выстрел Y М10"() -> (w269:u16)
            n170 = local read "Знак перех. dX М10"() -> (w271:i8)
            n171 = call "Формирование кластера параметров мишени (SubVI).vi"("Знак перемещения Dx"=w271, "выстрел X мишени"=w270, "выстрел Y мишени"=w269, "error in (no error)"=w275, "Параметры Мишени"=w274, "номер мишени (id)"=u8 10) -> ("Кластер параметров мишени"=w268:T7, "error out"=w276:errorcluster)  [unwired: 20 in]
          }
          frame 15 {
            # "Доп. команда"
            n172 = disable-structure shown="Disabled" {
              disable-tunnel: "Выстрелов до перемотки пленки" -> [w286 _]
              disable-tunnel: w280 -> [w285 w287]
              disable-tunnel: [w284 w287] -> w279
              disable-tunnel: [w283 _] -> w278
              frame Disabled {
                n173 = local read "id мишени"() -> (w282:u16)
                n174 = call "Команда обмена 5 (доп. команда) (SubVI).vi"("Выстрелов до перемотки"=w286, "error in"=w285, "номер мишени (id)"=w282) -> ("Кластер параметров 15-ой команды"=w283:T8, "error out"=w284:errorcluster)  [unwired: 23 in]
              }
              frame Enabled {
              }
            }
          }
          frame 170 {
            # "ВЫСТРЕЛ!"
            n175 = Unbundle By Name(w308) -> ("№ мишени"=w302:u8, "Коорд. выстрела X ст.байт"=w307:u8, "Коорд. выстрела X мл.байт"=w306:u8, "Коорд. выстрела Y cт.байт"=w305:u8, "Коорд. выстрела Y мл.байт"=w304:u8, "Знак dX"=w303:i8, "выст. до перем. пленки ст. байт"=w301:u8, "выст. до перем. пленки мл. байт"=w300:u8)
            n176 = Join Numbers(hi=w301, lo=w300) -> ((hi.lo)=w297:u16)
            n177 = property on="Осталось:" class="Slide (strict)"(error in=w299, "Value"=w297) -> (error out=w298:errorcluster)  [unwired: 1 in, 1 out]
            n178 = case shown="1, Default" w302 {
              tunnel: w307 -> [w319 w327 w334 w343 w351 w359 w367 w375 w383 w391]
              tunnel: w306 -> [w318 w326 w333 w342 w350 w358 w366 w374 w382 w390]
              tunnel: w305 -> [w317 w325 w332 w341 w349 w357 w365 w373 w381 w389]
              tunnel: w304 -> [w316 w324 w335 w340 w348 w356 w364 w372 w380 w388]
              tunnel: w303 -> [w314 w320 w330 w338 w344 w352 w360 w368 w376 w384]
              tunnel: w298 -> [w315 w323 w331 w339 w347 w355 w363 w371 w379 w387]
              tunnel: [w315 w323 w331 w339 w347 w355 w363 w371 w379 w387] -> w293
              frame 1, Default {
                n179 = Join Numbers(hi=w319, lo=w318) -> ((hi.lo)=w313:u16)
                n180 = Join Numbers(hi=w317, lo=w316) -> ((hi.lo)=w312:u16)
                n181 = local write "выстрел X М1"(w313) -> ()
                n182 = local write "выстрел Y М1"(w312) -> ()
                "Знак перех. dX М1" <- w314
              }
              frame 2 {
                n183 = Join Numbers(hi=w327, lo=w326) -> ((hi.lo)=w322:u16)
                n184 = Join Numbers(hi=w325, lo=w324) -> ((hi.lo)=w321:u16)
                n185 = local write "выстрел X М2"(w322) -> ()
                n186 = local write "выстрел Y М2"(w321) -> ()
                "Знак перех. dX М2" <- w320
              }
              frame 3 {
                n187 = Join Numbers(hi=w334, lo=w333) -> ((hi.lo)=w329:u16)
                n188 = Join Numbers(hi=w332, lo=w335) -> ((hi.lo)=w328:u16)
                n189 = local write "выстрел X М3"(w329) -> ()
                n190 = local write "выстрел Y М3"(w328) -> ()
                "Знак перех. dX М3" <- w330
              }
              frame 4 {
                n191 = Join Numbers(hi=w343, lo=w342) -> ((hi.lo)=w337:u16)
                n192 = Join Numbers(hi=w341, lo=w340) -> ((hi.lo)=w336:u16)
                n193 = local write "выстрел X М4"(w337) -> ()
                n194 = local write "выстрел Y М4"(w336) -> ()
                "Знак перех. dX М4" <- w338
              }
              frame 5 {
                n195 = Join Numbers(hi=w351, lo=w350) -> ((hi.lo)=w346:u16)
                n196 = Join Numbers(hi=w349, lo=w348) -> ((hi.lo)=w345:u16)
                n197 = local write "выстрел X М5"(w346) -> ()
                n198 = local write "выстрел Y М5"(w345) -> ()
                "Знак перех. dX М5" <- w344
              }
              frame 6 {
                n199 = Join Numbers(hi=w359, lo=w358) -> ((hi.lo)=w354:u16)
                n200 = Join Numbers(hi=w357, lo=w356) -> ((hi.lo)=w353:u16)
                n201 = local write "выстрел X М6"(w354) -> ()
                n202 = local write "выстрел Y М6"(w353) -> ()
                "Знак перех. dX М6" <- w352
              }
              frame 7 {
                n203 = Join Numbers(hi=w367, lo=w366) -> ((hi.lo)=w362:u16)
                n204 = Join Numbers(hi=w365, lo=w364) -> ((hi.lo)=w361:u16)
                n205 = local write "выстрел X М7"(w362) -> ()
                n206 = local write "выстрел Y М7"(w361) -> ()
                "Знак перех. dX М7" <- w360
              }
              frame 8 {
                n207 = Join Numbers(hi=w375, lo=w374) -> ((hi.lo)=w370:u16)
                n208 = Join Numbers(hi=w373, lo=w372) -> ((hi.lo)=w369:u16)
                n209 = local write "выстрел X М8"(w370) -> ()
                n210 = local write "выстрел Y М8"(w369) -> ()
                "Знак перех. dX М8" <- w368
              }
              frame 9 {
                n211 = Join Numbers(hi=w383, lo=w382) -> ((hi.lo)=w378:u16)
                n212 = Join Numbers(hi=w381, lo=w380) -> ((hi.lo)=w377:u16)
                n213 = local write "выстрел X М9"(w378) -> ()
                n214 = local write "выстрел Y М9"(w377) -> ()
                "Знак перех. dX М9" <- w376
              }
              frame 10 {
                n215 = Join Numbers(hi=w391, lo=w390) -> ((hi.lo)=w386:u16)
                n216 = Join Numbers(hi=w389, lo=w388) -> ((hi.lo)=w385:u16)
                n217 = local write "выстрел X М10"(w386) -> ()
                n218 = local write "выстрел Y М10"(w385) -> ()
                "Знак перех. dX М10" <- w384
              }
            }
            n219 = property on="XY лазера" class="Bool (strict)"(error in=w293, "Visible"=TRUE) -> (error out=w310:errorcluster)  [unwired: 1 in, 1 out]
            n220 = property on="текущ. инфо" class="Bool (strict)"(error in=w310, "Visible"=TRUE) -> (error out=w296:errorcluster)  [unwired: 1 in, 1 out]
            n221 = property on="Выстрел по мишени!" class="DigNum (strict)"(error in=w296) -> (error out=w295:errorcluster, "Value"=w294:u32)  [unwired: 1 in, 1 out]
            n222 = Increment(x=w294) -> (x+1=w311:u32)
            n223 = property on="Выстрел по мишени!" class="DigNum (strict)"(error in=w295, "Val(Sgnl)"=w311) -> (error out=w292:errorcluster)  [unwired: 1 in, 1 out]
            n224 = call "Управление звуком (SubVI).vi"("Звук выстрела"="Упр. звуком", "error in (no error)"=w292) -> ("error out"=w289:errorcluster)  [unwired: 7 in]
          }
          frame 171 {
            # "Текущее положение лазера, Готовность!"
            n225 = Unbundle By Name(w393) -> ("№ мишени"=w405:u8, "Коорд. выстрела X ст.байт"=w400:u8, "Коорд. выстрела X мл.байт"=w399:u8, "Знак dX"=w398:i8, "Коорд. выстрела Y cт.байт"=w397:u8, "Коорд. выстрела Y мл.байт"=w396:u8, "выст. до перем. пленки ст. байт"=w403:u8, "выст. до перем. пленки мл. байт"=w402:u8)
            n226 = Join Numbers(hi=w403, lo=w402) -> ((hi.lo)=w407:u16)
            n227 = property on="Осталось:" class="Slide (strict)"(error in=w404, "Value"=w407) -> (error out=w401:errorcluster)  [unwired: 1 in, 1 out]
            n228 = case shown="5" w405 {
              tunnel: [w420 w432 w444 w456 w468 w480 w492 w504 w516 w528] -> w392
              tunnel: w401 -> [w415 w427 w439 w451 w463 w475 w487 w499 w511 w523]
              tunnel: w400 -> [w424 w436 w448 w460 w472 w484 w496 w508 w520 w532]
              tunnel: w399 -> [w423 w435 w447 w459 w471 w483 w495 w507 w519 w531]
              tunnel: w398 -> [w413 w425 w437 w449 w461 w473 w485 w497 w509 w521]
              tunnel: w397 -> [w422 w434 w446 w458 w470 w482 w494 w506 w518 w530]
              tunnel: w396 -> [w421 w433 w445 w457 w469 w481 w493 w505 w517 w529]
              frame 1, Default {
                n229 = Join Numbers(hi=w424, lo=w423) -> ((hi.lo)=w417:u16)
                n230 = Join Numbers(hi=w422, lo=w421) -> ((hi.lo)=w414:u16)
                n231 = local write "Знак перех. dX М1"(w413) -> ()
                n232 = control-ref of="Мишень 1"() -> (w416:refnum<vi>)
                n233 = control-ref of="XY лазера"() -> (w419:refnum<vi>)
                n234 = control-ref of="текущ. инфо"() -> (w418:refnum<vi>)
                n235 = call "Положение лазера (SubVI).vi"("Мишень reference"=w416, "XY лазера reference"=w419, "Текущ. инфо reference"=w418, "error in"=w415, "X коорд."=w417, "Y коорд."=w414) -> ("error out"=w420:errorcluster)  [unwired: 21 in]
                n236 = local write "выстрел X М1"(w417) -> ()
                n237 = local write "выстрел Y М1"(w414) -> ()
              }
              frame 2 {
                n238 = Join Numbers(hi=w436, lo=w435) -> ((hi.lo)=w429:u16)
                n239 = Join Numbers(hi=w434, lo=w433) -> ((hi.lo)=w426:u16)
                n240 = local write "Знак перех. dX М2"(w425) -> ()
                n241 = control-ref of="Мишень 2"() -> (w428:refnum<vi>)
                n242 = control-ref of="XY лазера"() -> (w431:refnum<vi>)
                n243 = control-ref of="текущ. инфо"() -> (w430:refnum<vi>)
                n244 = call "Положение лазера (SubVI).vi"("Мишень reference"=w428, "XY лазера reference"=w431, "Текущ. инфо reference"=w430, "error in"=w427, "X коорд."=w429, "Y коорд."=w426) -> ("error out"=w432:errorcluster)  [unwired: 21 in]
                n245 = local write "выстрел X М2"(w429) -> ()
                n246 = local write "выстрел Y М2"(w426) -> ()
              }
              frame 3 {
                n247 = Join Numbers(hi=w448, lo=w447) -> ((hi.lo)=w441:u16)
                n248 = Join Numbers(hi=w446, lo=w445) -> ((hi.lo)=w438:u16)
                n249 = local write "Знак перех. dX М3"(w437) -> ()
                n250 = control-ref of="Мишень 3"() -> (w440:refnum<vi>)
                n251 = control-ref of="XY лазера"() -> (w443:refnum<vi>)
                n252 = control-ref of="текущ. инфо"() -> (w442:refnum<vi>)
                n253 = call "Положение лазера (SubVI).vi"("Мишень reference"=w440, "XY лазера reference"=w443, "Текущ. инфо reference"=w442, "error in"=w439, "X коорд."=w441, "Y коорд."=w438) -> ("error out"=w444:errorcluster)  [unwired: 21 in]
                n254 = local write "выстрел X М3"(w441) -> ()
                n255 = local write "выстрел Y М3"(w438) -> ()
              }
              frame 4 {
                n256 = Join Numbers(hi=w460, lo=w459) -> ((hi.lo)=w453:u16)
                n257 = Join Numbers(hi=w458, lo=w457) -> ((hi.lo)=w450:u16)
                n258 = local write "Знак перех. dX М4"(w449) -> ()
                n259 = control-ref of="Мишень 4"() -> (w452:refnum<vi>)
                n260 = control-ref of="XY лазера"() -> (w455:refnum<vi>)
                n261 = control-ref of="текущ. инфо"() -> (w454:refnum<vi>)
                n262 = call "Положение лазера (SubVI).vi"("Мишень reference"=w452, "XY лазера reference"=w455, "Текущ. инфо reference"=w454, "error in"=w451, "X коорд."=w453, "Y коорд."=w450) -> ("error out"=w456:errorcluster)  [unwired: 21 in]
                n263 = local write "выстрел X М4"(w453) -> ()
                n264 = local write "выстрел Y М4"(w450) -> ()
              }
              frame 5 {
                n265 = Join Numbers(hi=w472, lo=w471) -> ((hi.lo)=w465:u16)
                n266 = Join Numbers(hi=w470, lo=w469) -> ((hi.lo)=w462:u16)
                n267 = local write "Знак перех. dX М5"(w461) -> ()
                n268 = control-ref of="Мишень 5"() -> (w464:refnum<vi>)
                n269 = control-ref of="XY лазера"() -> (w467:refnum<vi>)
                n270 = control-ref of="текущ. инфо"() -> (w466:refnum<vi>)
                n271 = call "Положение лазера (SubVI).vi"("Мишень reference"=w464, "XY лазера reference"=w467, "Текущ. инфо reference"=w466, "error in"=w463, "X коорд."=w465, "Y коорд."=w462) -> ("error out"=w468:errorcluster)  [unwired: 21 in]
                n272 = local write "выстрел X М5"(w465) -> ()
                n273 = local write "выстрел Y М5"(w462) -> ()
              }
              frame 6 {
                n274 = Join Numbers(hi=w484, lo=w483) -> ((hi.lo)=w477:u16)
                n275 = Join Numbers(hi=w482, lo=w481) -> ((hi.lo)=w474:u16)
                n276 = local write "Знак перех. dX М6"(w473) -> ()
                n277 = control-ref of="Мишень 6"() -> (w476:refnum<vi>)
                n278 = control-ref of="XY лазера"() -> (w479:refnum<vi>)
                n279 = control-ref of="текущ. инфо"() -> (w478:refnum<vi>)
                n280 = call "Положение лазера (SubVI).vi"("Мишень reference"=w476, "XY лазера reference"=w479, "Текущ. инфо reference"=w478, "error in"=w475, "X коорд."=w477, "Y коорд."=w474) -> ("error out"=w480:errorcluster)  [unwired: 21 in]
                n281 = local write "выстрел X М6"(w477) -> ()
                n282 = local write "выстрел Y М6"(w474) -> ()
              }
              frame 7 {
                n283 = Join Numbers(hi=w496, lo=w495) -> ((hi.lo)=w489:u16)
                n284 = Join Numbers(hi=w494, lo=w493) -> ((hi.lo)=w486:u16)
                n285 = local write "Знак перех. dX М7"(w485) -> ()
                n286 = control-ref of="Мишень 7"() -> (w488:refnum<vi>)
                n287 = control-ref of="XY лазера"() -> (w491:refnum<vi>)
                n288 = control-ref of="текущ. инфо"() -> (w490:refnum<vi>)
                n289 = call "Положение лазера (SubVI).vi"("Мишень reference"=w488, "XY лазера reference"=w491, "Текущ. инфо reference"=w490, "error in"=w487, "X коорд."=w489, "Y коорд."=w486) -> ("error out"=w492:errorcluster)  [unwired: 21 in]
                n290 = local write "выстрел X М7"(w489) -> ()
                n291 = local write "выстрел Y М7"(w486) -> ()
              }
              frame 8 {
                n292 = Join Numbers(hi=w508, lo=w507) -> ((hi.lo)=w501:u16)
                n293 = Join Numbers(hi=w506, lo=w505) -> ((hi.lo)=w498:u16)
                n294 = local write "Знак перех. dX М8"(w497) -> ()
                n295 = control-ref of="Мишень 8"() -> (w500:refnum<vi>)
                n296 = control-ref of="XY лазера"() -> (w503:refnum<vi>)
                n297 = control-ref of="текущ. инфо"() -> (w502:refnum<vi>)
                n298 = call "Положение лазера (SubVI).vi"("Мишень reference"=w500, "XY лазера reference"=w503, "Текущ. инфо reference"=w502, "error in"=w499, "X коорд."=w501, "Y коорд."=w498) -> ("error out"=w504:errorcluster)  [unwired: 21 in]
                n299 = local write "выстрел X М8"(w501) -> ()
                n300 = local write "выстрел Y М8"(w498) -> ()
              }
              frame 9 {
                n301 = Join Numbers(hi=w520, lo=w519) -> ((hi.lo)=w513:u16)
                n302 = Join Numbers(hi=w518, lo=w517) -> ((hi.lo)=w510:u16)
                n303 = local write "Знак перех. dX М9"(w509) -> ()
                n304 = control-ref of="Мишень 9"() -> (w512:refnum<vi>)
                n305 = control-ref of="XY лазера"() -> (w515:refnum<vi>)
                n306 = control-ref of="текущ. инфо"() -> (w514:refnum<vi>)
                n307 = call "Положение лазера (SubVI).vi"("Мишень reference"=w512, "XY лазера reference"=w515, "Текущ. инфо reference"=w514, "error in"=w511, "X коорд."=w513, "Y коорд."=w510) -> ("error out"=w516:errorcluster)  [unwired: 21 in]
                n308 = local write "выстрел X М9"(w513) -> ()
                n309 = local write "выстрел Y М9"(w510) -> ()
              }
              frame 10 {
                n310 = Join Numbers(hi=w532, lo=w531) -> ((hi.lo)=w525:u16)
                n311 = Join Numbers(hi=w530, lo=w529) -> ((hi.lo)=w522:u16)
                n312 = local write "Знак перех. dX М10"(w521) -> ()
                n313 = control-ref of="Мишень 10"() -> (w524:refnum<vi>)
                n314 = control-ref of="XY лазера"() -> (w527:refnum<vi>)
                n315 = control-ref of="текущ. инфо"() -> (w526:refnum<vi>)
                n316 = call "Положение лазера (SubVI).vi"("Мишень reference"=w524, "XY лазера reference"=w527, "Текущ. инфо reference"=w526, "error in"=w523, "X коорд."=w525, "Y коорд."=w522) -> ("error out"=w528:errorcluster)  [unwired: 21 in]
                n317 = local write "выстрел X М10"(w525) -> ()
                n318 = local write "выстрел Y М10"(w522) -> ()
              }
            }
            n319 = property on="XY лазера" class="Bool (strict)"("Visible"=TRUE) -> ()  [unwired: 2 in, 2 out]
            n320 = property on="Шаг вперед" class="Bool (strict)"("DisabledEnum"=u8 0 ("y")) -> ()  [unwired: 2 in, 2 out]
            n321 = property on="текущ. инфо" class="Bool (strict)"("Visible"=TRUE) -> ()  [unwired: 2 in, 2 out]
            n322 = property on="Статус" class="Bool (strict)"("Caption.Text"="Готов!" ("Label.Text")) -> (error out=w408:errorcluster)  [unwired: 2 in, 1 out]
            n323 = property on="Статус" class="Bool (strict)"(error in=w408, "Caption.Position"=T4 {"Left"=970, "Top"=-32}) -> ()  [unwired: 1 in, 2 out]
            n324 = property on="Статус" class="Bool (strict)"("Caption.TextColor"=u32 56339 ("цвет")) -> ()  [unwired: 2 in, 2 out]
          }
          frame 172 {
            # "Команда занятости"
            n325 = Unbundle By Name(w537) -> ("№ мишени"=w548:u8, "Коорд. выстрела X ст.байт"=w544:u8, "Коорд. выстрела X мл.байт"=w543:u8, "Знак dX"=w535:i8, "Коорд. выстрела Y cт.байт"=w542:u8, "Коорд. выстрела Y мл.байт"=w541:u8, "выст. до перем. пленки ст. байт"=w547:u8, "выст. до перем. пленки мл. байт"=w546:u8)
            n326 = property on="XY лазера" class="Bool (strict)"("Visible"=FALSE) -> (error out=w551:errorcluster)  [unwired: 2 in, 1 out]
            n327 = property on="текущ. инфо" class="Bool (strict)"(error in=w551, "Visible"=FALSE) -> (error out=w552:errorcluster)  [unwired: 1 in, 1 out]
            n328 = Join Numbers(hi=w547, lo=w546) -> ((hi.lo)=w549:u16)
            n329 = property on="Осталось:" class="Slide (strict)"(error in=w536, "Value"=w549) -> (error out=w545:errorcluster)  [unwired: 1 in, 1 out]
            n330 = case shown="2" w548 {
              tunnel: [w565 w577 w589 w601 w613 w625 w637 w649 w661 w673] -> w533
              tunnel: w545 -> [w562 w574 w586 w598 w610 w622 w634 w646 w658 w670]
              tunnel: w544 -> [w569 w581 w593 w605 w617 w629 w641 w653 w665 w677]
              tunnel: w543 -> [w568 w580 w592 w604 w616 w628 w640 w652 w664 w676]
              tunnel: w535 -> [w558 w570 w582 w594 w606 w618 w630 w642 w654 w666]
              tunnel: w542 -> [w567 w579 w591 w603 w615 w627 w639 w651 w663 w675]
              tunnel: w541 -> [w566 w578 w590 w602 w614 w626 w638 w650 w662 w674]
              frame 1, Default {
                n331 = Join Numbers(hi=w569, lo=w568) -> ((hi.lo)=w559:u16)
                n332 = Join Numbers(hi=w567, lo=w566) -> ((hi.lo)=w560:u16)
                n333 = local write "Знак перех. dX М1"(w558) -> ()
                n334 = control-ref of="Мишень 1"() -> (w561:refnum<vi>)
                n335 = control-ref of="XY лазера"() -> (w564:refnum<vi>)
                n336 = control-ref of="текущ. инфо"() -> (w563:refnum<vi>)
                n337 = call "Положение лазера (SubVI).vi"("Мишень reference"=w561, "XY лазера reference"=w564, "Текущ. инфо reference"=w563, "error in"=w562, "X коорд."=w559, "Y коорд."=w560) -> ("error out"=w565:errorcluster)  [unwired: 21 in]
                n338 = local write "выстрел X М1"(w559) -> ()
                n339 = local write "выстрел Y М1"(w560) -> ()
              }
              frame 2 {
                n340 = Join Numbers(hi=w581, lo=w580) -> ((hi.lo)=w571:u16)
                n341 = Join Numbers(hi=w579, lo=w578) -> ((hi.lo)=w572:u16)
                n342 = local write "Знак перех. dX М2"(w570) -> ()
                n343 = control-ref of="Мишень 2"() -> (w573:refnum<vi>)
                n344 = control-ref of="XY лазера"() -> (w576:refnum<vi>)
                n345 = control-ref of="текущ. инфо"() -> (w575:refnum<vi>)
                n346 = call "Положение лазера (SubVI).vi"("Мишень reference"=w573, "XY лазера reference"=w576, "Текущ. инфо reference"=w575, "error in"=w574, "X коорд."=w571, "Y коорд."=w572) -> ("error out"=w577:errorcluster)  [unwired: 21 in]
                n347 = local write "выстрел X М2"(w571) -> ()
                n348 = local write "выстрел Y М2"(w572) -> ()
              }
              frame 3 {
                n349 = Join Numbers(hi=w593, lo=w592) -> ((hi.lo)=w583:u16)
                n350 = Join Numbers(hi=w591, lo=w590) -> ((hi.lo)=w584:u16)
                n351 = local write "Знак перех. dX М3"(w582) -> ()
                n352 = control-ref of="Мишень 3"() -> (w585:refnum<vi>)
                n353 = control-ref of="XY лазера"() -> (w588:refnum<vi>)
                n354 = control-ref of="текущ. инфо"() -> (w587:refnum<vi>)
                n355 = call "Положение лазера (SubVI).vi"("Мишень reference"=w585, "XY лазера reference"=w588, "Текущ. инфо reference"=w587, "error in"=w586, "X коорд."=w583, "Y коорд."=w584) -> ("error out"=w589:errorcluster)  [unwired: 21 in]
                n356 = local write "выстрел X М3"(w583) -> ()
                n357 = local write "выстрел Y М3"(w584) -> ()
              }
              frame 4 {
                n358 = Join Numbers(hi=w605, lo=w604) -> ((hi.lo)=w595:u16)
                n359 = Join Numbers(hi=w603, lo=w602) -> ((hi.lo)=w596:u16)
                n360 = local write "Знак перех. dX М4"(w594) -> ()
                n361 = control-ref of="Мишень 4"() -> (w597:refnum<vi>)
                n362 = control-ref of="XY лазера"() -> (w600:refnum<vi>)
                n363 = control-ref of="текущ. инфо"() -> (w599:refnum<vi>)
                n364 = call "Положение лазера (SubVI).vi"("Мишень reference"=w597, "XY лазера reference"=w600, "Текущ. инфо reference"=w599, "error in"=w598, "X коорд."=w595, "Y коорд."=w596) -> ("error out"=w601:errorcluster)  [unwired: 21 in]
                n365 = local write "выстрел X М4"(w595) -> ()
                n366 = local write "выстрел Y М4"(w596) -> ()
              }
              frame 5 {
                n367 = Join Numbers(hi=w617, lo=w616) -> ((hi.lo)=w607:u16)
                n368 = Join Numbers(hi=w615, lo=w614) -> ((hi.lo)=w608:u16)
                n369 = local write "Знак перех. dX М5"(w606) -> ()
                n370 = control-ref of="Мишень 5"() -> (w609:refnum<vi>)
                n371 = control-ref of="XY лазера"() -> (w612:refnum<vi>)
                n372 = control-ref of="текущ. инфо"() -> (w611:refnum<vi>)
                n373 = call "Положение лазера (SubVI).vi"("Мишень reference"=w609, "XY лазера reference"=w612, "Текущ. инфо reference"=w611, "error in"=w610, "X коорд."=w607, "Y коорд."=w608) -> ("error out"=w613:errorcluster)  [unwired: 21 in]
                n374 = local write "выстрел X М5"(w607) -> ()
                n375 = local write "выстрел Y М5"(w608) -> ()
              }
              frame 6 {
                n376 = Join Numbers(hi=w629, lo=w628) -> ((hi.lo)=w619:u16)
                n377 = Join Numbers(hi=w627, lo=w626) -> ((hi.lo)=w620:u16)
                n378 = local write "Знак перех. dX М6"(w618) -> ()
                n379 = control-ref of="Мишень 6"() -> (w621:refnum<vi>)
                n380 = control-ref of="XY лазера"() -> (w624:refnum<vi>)
                n381 = control-ref of="текущ. инфо"() -> (w623:refnum<vi>)
                n382 = call "Положение лазера (SubVI).vi"("Мишень reference"=w621, "XY лазера reference"=w624, "Текущ. инфо reference"=w623, "error in"=w622, "X коорд."=w619, "Y коорд."=w620) -> ("error out"=w625:errorcluster)  [unwired: 21 in]
                n383 = local write "выстрел X М6"(w619) -> ()
                n384 = local write "выстрел Y М6"(w620) -> ()
              }
              frame 7 {
                n385 = Join Numbers(hi=w641, lo=w640) -> ((hi.lo)=w631:u16)
                n386 = Join Numbers(hi=w639, lo=w638) -> ((hi.lo)=w632:u16)
                n387 = local write "Знак перех. dX М7"(w630) -> ()
                n388 = control-ref of="Мишень 7"() -> (w633:refnum<vi>)
                n389 = control-ref of="XY лазера"() -> (w636:refnum<vi>)
                n390 = control-ref of="текущ. инфо"() -> (w635:refnum<vi>)
                n391 = call "Положение лазера (SubVI).vi"("Мишень reference"=w633, "XY лазера reference"=w636, "Текущ. инфо reference"=w635, "error in"=w634, "X коорд."=w631, "Y коорд."=w632) -> ("error out"=w637:errorcluster)  [unwired: 21 in]
                n392 = local write "выстрел X М7"(w631) -> ()
                n393 = local write "выстрел Y М7"(w632) -> ()
              }
              frame 8 {
                n394 = Join Numbers(hi=w653, lo=w652) -> ((hi.lo)=w643:u16)
                n395 = Join Numbers(hi=w651, lo=w650) -> ((hi.lo)=w644:u16)
                n396 = local write "Знак перех. dX М8"(w642) -> ()
                n397 = control-ref of="Мишень 8"() -> (w645:refnum<vi>)
                n398 = control-ref of="XY лазера"() -> (w648:refnum<vi>)
                n399 = control-ref of="текущ. инфо"() -> (w647:refnum<vi>)
                n400 = call "Положение лазера (SubVI).vi"("Мишень reference"=w645, "XY лазера reference"=w648, "Текущ. инфо reference"=w647, "error in"=w646, "X коорд."=w643, "Y коорд."=w644) -> ("error out"=w649:errorcluster)  [unwired: 21 in]
                n401 = local write "выстрел X М8"(w643) -> ()
                n402 = local write "выстрел Y М8"(w644) -> ()
              }
              frame 9 {
                n403 = Join Numbers(hi=w665, lo=w664) -> ((hi.lo)=w655:u16)
                n404 = Join Numbers(hi=w663, lo=w662) -> ((hi.lo)=w656:u16)
                n405 = local write "Знак перех. dX М9"(w654) -> ()
                n406 = control-ref of="Мишень 9"() -> (w657:refnum<vi>)
                n407 = control-ref of="XY лазера"() -> (w660:refnum<vi>)
                n408 = control-ref of="текущ. инфо"() -> (w659:refnum<vi>)
                n409 = call "Положение лазера (SubVI).vi"("Мишень reference"=w657, "XY лазера reference"=w660, "Текущ. инфо reference"=w659, "error in"=w658, "X коорд."=w655, "Y коорд."=w656) -> ("error out"=w661:errorcluster)  [unwired: 21 in]
                n410 = local write "выстрел X М9"(w655) -> ()
                n411 = local write "выстрел Y М9"(w656) -> ()
              }
              frame 10 {
                n412 = Join Numbers(hi=w677, lo=w676) -> ((hi.lo)=w667:u16)
                n413 = Join Numbers(hi=w675, lo=w674) -> ((hi.lo)=w668:u16)
                n414 = local write "Знак перех. dX М10"(w666) -> ()
                n415 = control-ref of="Мишень 10"() -> (w669:refnum<vi>)
                n416 = control-ref of="XY лазера"() -> (w672:refnum<vi>)
                n417 = control-ref of="текущ. инфо"() -> (w671:refnum<vi>)
                n418 = call "Положение лазера (SubVI).vi"("Мишень reference"=w669, "XY лазера reference"=w672, "Текущ. инфо reference"=w671, "error in"=w670, "X коорд."=w667, "Y коорд."=w668) -> ("error out"=w673:errorcluster)  [unwired: 21 in]
                n419 = local write "выстрел X М10"(w667) -> ()
                n420 = local write "выстрел Y М10"(w668) -> ()
              }
            }
            n421 = property on="Статус" class="Bool (strict)"(error in=w552, "Visible"=TRUE) -> (error out=w538:errorcluster)  [unwired: 1 in, 1 out]
            n422 = property on="Статус" class="Bool (strict)"(error in=w538, "Caption.Text"="Идет перемещение..." ("Label.Text")) -> (error out=w539:errorcluster)  [unwired: 1 in, 1 out]
            n423 = property on="Статус" class="Bool (strict)"(error in=w539, "Caption.TextColor"=u32 16711680 ("цвет")) -> (error out=w540:errorcluster)  [unwired: 1 in, 1 out]
            n424 = property on="Статус" class="Bool (strict)"(error in=w540, "Caption.Position"=T4 {"Left"=800, "Top"=-32}) -> ()  [unwired: 1 in, 2 out]
          }
          frame 199 {
            # "Команда \"Блок на связи, режим ожидания\""
          }
        }
        n425 = Join Numbers(hi=w122, lo=w121) -> ((hi.lo)=w118:u16)
        n426 = case "Вывод ифн. об оставшися выстрелах в текущую точку" shown="10" w120 {
          tunnel: w118 -> [w678 w679 w680 w681 w682 w683 w684 w685 w686 w687 _]
          tunnel: [w678 w679 w680 w681 w682 w683 w684 w685 w686 w687 _] -> w119
          frame 1 {
            n427 = property on="Выстрелов осталось M1" class="DigNum (strict)"("Value"=w678) -> ()  [unwired: 2 in, 2 out]
          }
          frame 2 {
            n428 = property on="Выстрелов осталось M2" class="DigNum (strict)"("Value"=w679) -> ()  [unwired: 2 in, 2 out]
          }
          frame 3 {
            n429 = property on="Выстрелов осталось M3" class="DigNum (strict)"("Value"=w680) -> ()  [unwired: 2 in, 2 out]
          }
          frame 4 {
            n430 = property on="Выстрелов осталось M4" class="DigNum (strict)"("Value"=w681) -> ()  [unwired: 2 in, 2 out]
          }
          frame 5 {
            n431 = property on="Выстрелов осталось M5" class="DigNum (strict)"("Value"=w682) -> ()  [unwired: 2 in, 2 out]
          }
          frame 6 {
            n432 = property on="Выстрелов осталось M6" class="DigNum (strict)"("Value"=w683) -> ()  [unwired: 2 in, 2 out]
          }
          frame 7 {
            n433 = property on="Выстрелов осталось M7" class="DigNum (strict)"("Value"=w684) -> ()  [unwired: 2 in, 2 out]
          }
          frame 8 {
            n434 = property on="Выстрелов осталось M8" class="DigNum (strict)"("Value"=w685) -> ()  [unwired: 2 in, 2 out]
          }
          frame 9 {
            n435 = property on="Выстрелов осталось M9" class="DigNum (strict)"("Value"=w686) -> ()  [unwired: 2 in, 2 out]
          }
          frame 10 {
            n436 = property on="Выстрелов осталось M10" class="DigNum (strict)"("Value"=w687) -> ()  [unwired: 2 in, 2 out]
          }
          frame 11, Default {
          }
        }
        n437 = Not Equal To 0?(x=w119) -> (x != 0?=w117:bool)
        n438 = case shown="True" w117 {
          tunnel: w119 -> [_ w139]
          frame False {
          }
          frame True {
            n439 = Number To Decimal String(number=w139) -> (decimal integer string=w138:string)  [unwired: 1 in]
            n440 = property on="текущ. инфо" class="Bool (strict)"("Caption.Text"=w138) -> ()  [unwired: 2 in, 2 out]
          }
        }
        n441 = case shown="True" w123 {
          tunnel: [w132 w137] -> w131
          tunnel: w126 -> [w132 w134]
          tunnel: w125 -> [_ w133]
          frame False {
          }
          frame True {
            n442 = property on="TCP con ID" class="Ref (strict)"(error in=w134) -> (error out=w136:errorcluster, "Value"=w135:refnum<k5>)  [unwired: 1 in, 1 out]
            n443 = call "Передать кластер параметров в TCP (SubVI).vi"("Кластер параметров мишени"=w133, "error in"=w136, "TCP connection ID"=w135) -> ("error out"=w137:errorcluster)  [unwired: 11 in, 1 out]
          }
        }
      }
      event "Выстрел по мишени!": Value Change {
        # "Отрисовка точек на мишенях"
        n444 = event-data() -> ()  [unwired: 2 out]
        n445 = property on="id мишени" class="DigNum (strict)"(error in=w695) -> (error out=w697:errorcluster, "Value"=w700:u16)  [unwired: 1 in, 1 out]
        n446 = case "Считывание состояния \n  мишени до выстрела" shown="7" w700 {
          selector: w700 -> [w755 w760 w765 w770 w775 w780 w785 w790 w795 w800]
          tunnel: ["выстрел Y М1" "выстрел Y М2" "выстрел Y М3" "выстрел Y М4" "выстрел Y М5" "выстрел Y М6" "выстрел Y М7" "выстрел Y М8" "выстрел Y М9" "выстрел Y М10"] -> w693
          tunnel: ["выстрел X М1" "выстрел X М2" "выстрел X М3" "выстрел X М4" "выстрел X М5" "выстрел X М6" "выстрел X М7" "выстрел X М8" "выстрел X М9" "выстрел X М10"] -> w694
          tunnel: [w755 w760 w765 w770 w775 w780 w785 w790 w795 w800] -> w692
          tunnel: w697 -> [w754 w759 w764 w769 w774 w779 w784 w789 w794 w799]
          tunnel: [w754 w759 w764 w769 w774 w779 w784 w789 w794 w799] -> w696
          tunnel: ["Мишень 1" "Мишень 2" "Мишень 3" "Мишень 4" "Мишень 5" "Мишень 6" "Мишень 7" "Мишень 8" "Мишень 9" "Мишень 10"] -> w690
          frame 1, Default {
          }
          frame 2 {
          }
          frame 3 {
          }
          frame 4 {
          }
          frame 5 {
          }
          frame 6 {
          }
          frame 7 {
          }
          frame 8 {
          }
          frame 9 {
          }
          frame 10 {
          }
        }
        n447 = call "Добавить точку на рисунок (SubVI).vi"("in picture"=w690, "id мишени вх"=w692, "цвет"=u32 16777222, "error in"=w696, "dot х"=w694, "dot y"=w693) -> ("error out"=w699:errorcluster, "id мишени вых"=w691:u16, "out picture"=w698:picture)  [unwired: 11 in]
        n448 = case "Обновление мишени при выстреле" shown="1, Default" w691 {
          tunnel: w694 -> [w705 w710 w715 w719 w724 w729 w734 w739 w744 w749]
          tunnel: w693 -> [w704 w709 w714 w720 w725 w730 w735 w740 w745 w750]
          tunnel: w699 -> [w703 w708 w713 w717 w723 w728 w733 w738 w743 w748]
          tunnel: w698 -> [w701 w706 w711 w718 w721 w726 w731 w736 w741 w746]
          tunnel: [w702 w707 w712 w716 w722 w727 w732 w737 w742 w747] -> w689
          frame 1, Default {
            n449 = local write "выстрел X М1"(w705) -> ()
            n450 = property on="Мишень 1" class="Pict"(error in=w703, "Value"=w701) -> (error out=w702:errorcluster)  [unwired: 1 in, 1 out]
            n451 = local write "выстрел Y М1"(w704) -> ()
          }
          frame 2 {
            n452 = property on="Мишень 2" class="Pict"(error in=w708, "Value"=w706) -> (error out=w707:errorcluster)  [unwired: 1 in, 1 out]
            n453 = local write "выстрел X М2"(w710) -> ()
            n454 = local write "выстрел Y М2"(w709) -> ()
          }
          frame 3 {
            n455 = local write "выстрел X М3"(w715) -> ()
            n456 = property on="Мишень 3" class="Pict"(error in=w713, "Value"=w711) -> (error out=w712:errorcluster)  [unwired: 1 in, 1 out]
            n457 = local write "выстрел Y М3"(w714) -> ()
          }
          frame 4 {
            n458 = local write "выстрел X М4"(w719) -> ()
            n459 = property on="Мишень 4" class="Pict"(error in=w717, "Value"=w718) -> (error out=w716:errorcluster)  [unwired: 1 in, 1 out]
            n460 = local write "выстрел Y М4"(w720) -> ()
          }
          frame 5 {
            n461 = local write "выстрел X М5"(w724) -> ()
            n462 = local write "выстрел Y М5"(w725) -> ()
            n463 = property on="Мишень 5" class="Pict"(error in=w723, "Value"=w721) -> (error out=w722:errorcluster)  [unwired: 1 in, 1 out]
          }
          frame 6 {
            n464 = local write "выстрел X М6"(w729) -> ()
            n465 = local write "выстрел Y М6"(w730) -> ()
            n466 = property on="Мишень 6" class="Pict"(error in=w728, "Value"=w726) -> (error out=w727:errorcluster)  [unwired: 1 in, 1 out]
          }
          frame 7 {
            n467 = local write "выстрел X М7"(w734) -> ()
            n468 = local write "выстрел Y М7"(w735) -> ()
            n469 = property on="Мишень 7" class="Pict"(error in=w733, "Value"=w731) -> (error out=w732:errorcluster)  [unwired: 1 in, 1 out]
          }
          frame 8 {
            n470 = local write "выстрел X М8"(w739) -> ()
            n471 = local write "выстрел Y М8"(w740) -> ()
            n472 = property on="Мишень 8" class="Pict"(error in=w738, "Value"=w736) -> (error out=w737:errorcluster)  [unwired: 1 in, 1 out]
          }
          frame 9 {
            n473 = local write "выстрел X М9"(w744) -> ()
            n474 = local write "выстрел Y М9"(w745) -> ()
            n475 = property on="Мишень 9" class="Pict"(error in=w743, "Value"=w741) -> (error out=w742:errorcluster)  [unwired: 1 in, 1 out]
          }
          frame 10 {
            n476 = local write "выстрел X М10"(w749) -> ()
            n477 = local write "выстрел Y М10"(w750) -> ()
            n478 = property on="Мишень 10" class="Pict"(error in=w748, "Value"=w746) -> (error out=w747:errorcluster)  [unwired: 1 in, 1 out]
          }
        }
      }
      event Mouse Move {
        # "Работа с курсором - линейка"
        n479 = event-data() -> ()  [unwired: 2 out]
        n480 = control-ref of="This VI"() -> (w807:refnum<vi>)
        n481 = call "Линейка (SubVI).vi"("Mouse ID in"=w806, "VI reference"=w807, "error in (no error)"=w805) -> ("Mouse ID out"=w804:refnum<k1>, "Slide Horizontal"=→"Slide X axis":u8, "Slide Vertical"=→"Slide Y axis":u8, "error out"=w802:errorcluster)  [unwired: 13 in]
        n482 = local read "Выстрелов до перемотки пленки"() -> (w803:u16)
        n483 = property on="Осталось:" class="Slide (strict)"(error in=w802, "Scale.Maximum"=w803) -> (error out=w801:errorcluster)  [unwired: 1 in, 1 out]
      }
      event "Добавить мишень": Value Change {
        n484 = event-data() -> ("OldVal"=w814:bool)  [unwired: 1 out]
        n485 = property on="Добавить мишень" class="Bool (strict)"(error in=w815, "Value"=w814) -> (error out=w813:errorcluster)  [unwired: 1 in, 1 out]
        n486 = property on="Счетчик мишеней" class="DigNum (strict)"(error in=w813) -> (error out=w817:errorcluster, "Value"=w810:u8)  [unwired: 1 in, 1 out]
        n487 = Increment(x=w810) -> (x+1=w818:u8)
        "Счетчик мишеней" <- w818
        n488 = Greater Or Equal?(x=w810, y=u8 10) -> (x >= y?=w811:bool)
        n489 = case shown="True" w811 {
          frame False {
          }
          frame True {
            n490 = property on="Добавить мишень" class="Bool (strict)"("DisabledEnum"=T3."Disabled and Grayed Out" ("Disabled")) -> ()  [unwired: 2 in, 2 out]
          }
        }
        n491 = case shown="1" w818 {
          tunnel: w817 -> [w820 w823 w824 w827 w830 w833 w836 w839 w842 w845 w848]
          tunnel: [w820 w821 w825 w829 w832 w834 w837 w840 w843 w846 w849] -> w816
          frame 0, Default {
          }
          frame 1 {
            n492 = property on="Мишень 1" class="Pict"(error in=w823, "Visible"=TRUE) -> (error out=w821:errorcluster)  [unwired: 1 in, 1 out]
          }
          frame 2 {
            n493 = property on="Мишень 2" class="Pict"(error in=w824, "Visible"=TRUE) -> (error out=w825:errorcluster)  [unwired: 1 in, 1 out]
          }
          frame 3 {
            n494 = property on="Мишень 3" class="Pict"(error in=w827, "Visible"=TRUE) -> (error out=w829:errorcluster)  [unwired: 1 in, 1 out]
          }
          frame 4 {
            n495 = property on="Мишень 4" class="Pict"(error in=w830, "Visible"=TRUE) -> (error out=w832:errorcluster)  [unwired: 1 in, 1 out]
          }
          frame 5 {
            n496 = property on="Мишень 5" class="Pict"(error in=w833, "Visible"=TRUE) -> (error out=w834:errorcluster)  [unwired: 1 in, 1 out]
          }
          frame 6 {
            n497 = property on="Мишень 6" class="Pict"(error in=w836, "Visible"=TRUE) -> (error out=w837:errorcluster)  [unwired: 1 in, 1 out]
          }
          frame 7 {
            n498 = property on="Мишень 7" class="Pict"(error in=w839, "Visible"=TRUE) -> (error out=w840:errorcluster)  [unwired: 1 in, 1 out]
          }
          frame 8 {
            n499 = property on="Мишень 8" class="Pict"(error in=w842, "Visible"=TRUE) -> (error out=w843:errorcluster)  [unwired: 1 in, 1 out]
          }
          frame 9 {
            n500 = property on="Мишень 9" class="Pict"(error in=w845, "Visible"=TRUE) -> (error out=w846:errorcluster)  [unwired: 1 in, 1 out]
          }
          frame 10 {
            n501 = property on="Мишень 10" class="Pict"(error in=w848, "Visible"=TRUE) -> (error out=w849:errorcluster)  [unwired: 1 in, 1 out]
          }
        }
      }
      event "Мишень 1": Shortcut Menu Selection (User) {
        n502 = event-data() -> ("ItemTag"=w853:string)  [unwired: 1 out]
        n503 = case shown="\"Выбрать\"" w853 {
          tunnel: [w859 w867] -> w851
          tunnel: w852 -> [w854 w866]
          frame "Настроить", Default {
            n504 = call "Настройки мишени (Sub VI).vi"("Параметры мишеней вх"="М1", "error in"=w854) -> ("Параметры мишеней вых"=w858:T1, "error out"=w860:errorcluster)  [unwired: 16 in]
            n505 = Unbundle(w858) -> ("Название мишени"=w857:string, "Х0_position"=w865:u16, "Y0_position"=w864:u16, "Длина, мм"=w863:u16, "Ширина, мм"=w862:u16)  [unwired: 5 out]
            n506 = property on="М1" class="Clust (strict)"(error in=w860, "Val(Sgnl)"=w858) -> (error out=w859:errorcluster)  [unwired: 1 in, 1 out]
            n507 = Bundle("Х0_position"=w865, "Y0_position"=w864) -> (w856:cluster{"Х0_position":u16, "Y0_position":u16})  [unwired: 1 in]
            n508 = Bundle("Длина, мм"=w863, "Ширина, мм"=w862) -> (w855:cluster{"Длина, мм":u16, "Ширина, мм":u16})  [unwired: 1 in]
            n509 = property on="Мишень 1" class="Pict"("TipStrip"=w857) -> ()  [unwired: 2 in, 2 out]
            n510 = property on="Мишень 1" class="Pict"("Position"=w856) -> ()  [unwired: 2 in, 2 out]
            n511 = property on="Мишень 1" class="Pict"("Draw Area Size"=w855) -> ()  [unwired: 2 in, 2 out]
          }
          frame "Выбрать" {
            n512 = Two Button Dialog(message="Вы уверены, что хотите выбрать эту мишень?", 1:"Нет" ("F button name (\"Cancel\")"), 2:"Да" ("T button name (\"OK\")")) -> (T button?=w868:bool)
            n513 = case shown="True" w868 {
              tunnel: [w872 w874] -> w867
              tunnel: w866 -> [w872 w873]
              frame False {
              }
              frame True {
                w875 = u16 1 ("id мишени")
                n514 = property on="id мишени" class="DigNum (strict)"(error in=w873, "Value"=w875) -> (error out=w876:errorcluster)  [unwired: 1 in, 1 out]
                n515 = property on="id мишени" class="DigNum (strict)"(error in=w876, "Val(Sgnl)"=w875) -> (error out=w874:errorcluster)  [unwired: 1 in, 1 out]
              }
            }
          }
        }
      }
      event "Мишень 2": Shortcut Menu Selection (User) {
        n516 = event-data() -> ("ItemTag"=w879:string)  [unwired: 1 out]
        n517 = case shown="\"Настроить\", Default" w879 {
          tunnel: w877 -> [w887 w894]
          tunnel: [w881 w893] -> w878
          frame "Настроить", Default {
            n518 = call "Настройки мишени (Sub VI).vi"("Параметры мишеней вх"="М2", "error in"=w887) -> ("Параметры мишеней вых"=w882:T1, "error out"=w883:errorcluster)  [unwired: 16 in]
            n519 = Unbundle(w882) -> ("Название мишени"=w886:string, "Х0_position"=w891:u16, "Y0_position"=w890:u16, "Длина, мм"=w889:u16, "Ширина, мм"=w888:u16)  [unwired: 5 out]
            n520 = property on="М2" class="Clust (strict)"(error in=w883, "Val(Sgnl)"=w882) -> (error out=w881:errorcluster)  [unwired: 1 in, 1 out]
            n521 = Bundle("Х0_position"=w891, "Y0_position"=w890) -> (w885:cluster{"Х0_position":u16, "Y0_position":u16})  [unwired: 1 in]
            n522 = Bundle("Длина, мм"=w889, "Ширина, мм"=w888) -> (w884:cluster{"Длина, мм":u16, "Ширина, мм":u16})  [unwired: 1 in]
            n523 = property on="Мишень 2" class="Pict"("TipStrip"=w886) -> ()  [unwired: 2 in, 2 out]
            n524 = property on="Мишень 2" class="Pict"("Position"=w885) -> ()  [unwired: 2 in, 2 out]
            n525 = property on="Мишень 2" class="Pict"("Draw Area Size"=w884) -> ()  [unwired: 2 in, 2 out]
          }
          frame "Выбрать" {
            n526 = Two Button Dialog(message="Вы уверены, что хотите выбрать эту мишень?", 1:"Нет" ("F button name (\"Cancel\")"), 2:"Да" ("T button name (\"OK\")")) -> (T button?=w897:bool)
            n527 = case shown="True" w897 {
              tunnel: [w898 w900] -> w893
              tunnel: w894 -> [w898 w899]
              frame False {
              }
              frame True {
                w901 = u16 2 ("id мишени")
                n528 = property on="id мишени" class="DigNum (strict)"(error in=w899, "Value"=w901) -> (error out=w902:errorcluster)  [unwired: 1 in, 1 out]
                n529 = property on="id мишени" class="DigNum (strict)"(error in=w902, "Val(Sgnl)"=w901) -> (error out=w900:errorcluster)  [unwired: 1 in, 1 out]
              }
            }
          }
        }
      }
      event "Мишень 3": Shortcut Menu Selection (User) {
        n530 = event-data() -> ("ItemTag"=w905:string)  [unwired: 1 out]
        n531 = case shown="\"Настроить\", Default" w905 {
          tunnel: w903 -> [w913 w920]
          tunnel: [w906 w919] -> w904
          frame "Настроить", Default {
            n532 = call "Настройки мишени (Sub VI).vi"("Параметры мишеней вх"="М3", "error in"=w913) -> ("Параметры мишеней вых"=w907:T1, "error out"=w908:errorcluster)  [unwired: 16 in]
            n533 = Unbundle(w907) -> ("Название мишени"=w912:string, "Х0_position"=w917:u16, "Y0_position"=w916:u16, "Длина, мм"=w915:u16, "Ширина, мм"=w914:u16)  [unwired: 5 out]
            n534 = property on="М3" class="Clust (strict)"(error in=w908, "Val(Sgnl)"=w907) -> (error out=w906:errorcluster)  [unwired: 1 in, 1 out]
            n535 = Bundle("Х0_position"=w917, "Y0_position"=w916) -> (w911:cluster{"Х0_position":u16, "Y0_position":u16})  [unwired: 1 in]
            n536 = Bundle("Длина, мм"=w915, "Ширина, мм"=w914) -> (w910:cluster{"Длина, мм":u16, "Ширина, мм":u16})  [unwired: 1 in]
            n537 = property on="Мишень 3" class="Pict"("TipStrip"=w912) -> ()  [unwired: 2 in, 2 out]
            n538 = property on="Мишень 3" class="Pict"("Position"=w911) -> ()  [unwired: 2 in, 2 out]
            n539 = property on="Мишень 3" class="Pict"("Draw Area Size"=w910) -> ()  [unwired: 2 in, 2 out]
          }
          frame "Выбрать" {
            n540 = Two Button Dialog(message="Вы уверены, что хотите выбрать эту мишень?", 1:"Нет" ("F button name (\"Cancel\")"), 2:"Да" ("T button name (\"OK\")")) -> (T button?=w923:bool)
            n541 = case shown="True" w923 {
              tunnel: [w924 w926] -> w919
              tunnel: w920 -> [w924 w925]
              frame False {
              }
              frame True {
                w927 = u16 3 ("id мишени")
                n542 = property on="id мишени" class="DigNum (strict)"(error in=w925, "Value"=w927) -> (error out=w928:errorcluster)  [unwired: 1 in, 1 out]
                n543 = property on="id мишени" class="DigNum (strict)"(error in=w928, "Val(Sgnl)"=w927) -> (error out=w926:errorcluster)  [unwired: 1 in, 1 out]
              }
            }
          }
        }
      }
      event "Мишень 4": Shortcut Menu Selection (User) {
        n544 = event-data() -> ("ItemTag"=w931:string)  [unwired: 1 out]
        n545 = case shown="\"Настроить\", Default" w931 {
          tunnel: w929 -> [w939 w944]
          tunnel: [w932 w945] -> w930
          frame "Настроить", Default {
            n546 = call "Настройки мишени (Sub VI).vi"("Параметры мишеней вх"="М4", "error in"=w939) -> ("Параметры мишеней вых"=w933:T1, "error out"=w934:errorcluster)  [unwired: 16 in]
            n547 = Unbundle(w933) -> ("Название мишени"=w938:string, "Х0_position"=w943:u16, "Y0_position"=w942:u16, "Длина, мм"=w941:u16, "Ширина, мм"=w940:u16)  [unwired: 5 out]
            n548 = property on="М4" class="Clust (strict)"(error in=w934, "Val(Sgnl)"=w933) -> (error out=w932:errorcluster)  [unwired: 1 in, 1 out]
            n549 = Bundle("Х0_position"=w943, "Y0_position"=w942) -> (w937:cluster{"Х0_position":u16, "Y0_position":u16})  [unwired: 1 in]
            n550 = Bundle("Длина, мм"=w941, "Ширина, мм"=w940) -> (w936:cluster{"Длина, мм":u16, "Ширина, мм":u16})  [unwired: 1 in]
            n551 = property on="Мишень 4" class="Pict"("TipStrip"=w938) -> ()  [unwired: 2 in, 2 out]
            n552 = property on="Мишень 4" class="Pict"("Position"=w937) -> ()  [unwired: 2 in, 2 out]
            n553 = property on="Мишень 4" class="Pict"("Draw Area Size"=w936) -> ()  [unwired: 2 in, 2 out]
          }
          frame "Выбрать" {
            n554 = Two Button Dialog(message="Вы уверены, что хотите выбрать эту мишень?", 1:"Нет" ("F button name (\"Cancel\")"), 2:"Да" ("T button name (\"OK\")")) -> (T button?=w949:bool)
            n555 = case shown="True" w949 {
              tunnel: [w950 w952] -> w945
              tunnel: w944 -> [w950 w951]
              frame False {
              }
              frame True {
                w953 = u16 4 ("id мишени")
                n556 = property on="id мишени" class="DigNum (strict)"(error in=w951, "Value"=w953) -> (error out=w954:errorcluster)  [unwired: 1 in, 1 out]
                n557 = property on="id мишени" class="DigNum (strict)"(error in=w954, "Val(Sgnl)"=w953) -> (error out=w952:errorcluster)  [unwired: 1 in, 1 out]
              }
            }
          }
        }
      }
      event "Мишень 5": Shortcut Menu Selection (User) {
        n558 = event-data() -> ("ItemTag"=w957:string)  [unwired: 1 out]
        n559 = case shown="\"Настроить\", Default" w957 {
          tunnel: w955 -> [w965 w971]
          tunnel: [w958 w970] -> w956
          frame "Настроить", Default {
            n560 = call "Настройки мишени (Sub VI).vi"("Параметры мишеней вх"="М5", "error in"=w965) -> ("Параметры мишеней вых"=w959:T1, "error out"=w960:errorcluster)  [unwired: 16 in]
            n561 = Unbundle(w959) -> ("Название мишени"=w964:string, "Х0_position"=w969:u16, "Y0_position"=w968:u16, "Длина, мм"=w967:u16, "Ширина, мм"=w966:u16)  [unwired: 5 out]
            n562 = property on="М5" class="Clust (strict)"(error in=w960, "Val(Sgnl)"=w959) -> (error out=w958:errorcluster)  [unwired: 1 in, 1 out]
            n563 = Bundle("Х0_position"=w969, "Y0_position"=w968) -> (w963:cluster{"Х0_position":u16, "Y0_position":u16})  [unwired: 1 in]
            n564 = Bundle("Длина, мм"=w967, "Ширина, мм"=w966) -> (w962:cluster{"Длина, мм":u16, "Ширина, мм":u16})  [unwired: 1 in]
            n565 = property on="Мишень 5" class="Pict"("TipStrip"=w964) -> ()  [unwired: 2 in, 2 out]
            n566 = property on="Мишень 5" class="Pict"("Position"=w963) -> ()  [unwired: 2 in, 2 out]
            n567 = property on="Мишень 5" class="Pict"("Draw Area Size"=w962) -> ()  [unwired: 2 in, 2 out]
          }
          frame "Выбрать" {
            n568 = Two Button Dialog(message="Вы уверены, что хотите выбрать эту мишень?", 1:"Нет" ("F button name (\"Cancel\")"), 2:"Да" ("T button name (\"OK\")")) -> (T button?=w975:bool)
            n569 = case shown="True" w975 {
              tunnel: [w976 w978] -> w970
              tunnel: w971 -> [w976 w977]
              frame False {
              }
              frame True {
                w979 = u16 5 ("id мишени")
                n570 = property on="id мишени" class="DigNum (strict)"(error in=w977, "Value"=w979) -> (error out=w980:errorcluster)  [unwired: 1 in, 1 out]
                n571 = property on="id мишени" class="DigNum (strict)"(error in=w980, "Val(Sgnl)"=w979) -> (error out=w978:errorcluster)  [unwired: 1 in, 1 out]
              }
            }
          }
        }
      }
      event "Мишень 6": Shortcut Menu Selection (User) {
        n572 = event-data() -> ("ItemTag"=w983:string)  [unwired: 1 out]
        n573 = case shown="\"Настроить\", Default" w983 {
          tunnel: w981 -> [w991 w997]
          tunnel: [w984 w996] -> w982
          frame "Настроить", Default {
            n574 = call "Настройки мишени (Sub VI).vi"("Параметры мишеней вх"="М6", "error in"=w991) -> ("Параметры мишеней вых"=w985:T1, "error out"=w986:errorcluster)  [unwired: 16 in]
            n575 = Unbundle(w985) -> ("Название мишени"=w990:string, "Х0_position"=w995:u16, "Y0_position"=w994:u16, "Длина, мм"=w993:u16, "Ширина, мм"=w992:u16)  [unwired: 5 out]
            n576 = property on="М6" class="Clust (strict)"(error in=w986, "Val(Sgnl)"=w985) -> (error out=w984:errorcluster)  [unwired: 1 in, 1 out]
            n577 = Bundle("Х0_position"=w995, "Y0_position"=w994) -> (w989:cluster{"Х0_position":u16, "Y0_position":u16})  [unwired: 1 in]
            n578 = Bundle("Длина, мм"=w993, "Ширина, мм"=w992) -> (w988:cluster{"Длина, мм":u16, "Ширина, мм":u16})  [unwired: 1 in]
            n579 = property on="Мишень 6" class="Pict"("TipStrip"=w990) -> ()  [unwired: 2 in, 2 out]
            n580 = property on="Мишень 6" class="Pict"("Position"=w989) -> ()  [unwired: 2 in, 2 out]
            n581 = property on="Мишень 6" class="Pict"("Draw Area Size"=w988) -> ()  [unwired: 2 in, 2 out]
          }
          frame "Выбрать" {
            n582 = Two Button Dialog(message="Вы уверены, что хотите выбрать эту мишень?", 1:"Нет" ("F button name (\"Cancel\")"), 2:"Да" ("T button name (\"OK\")")) -> (T button?=w1001:bool)
            n583 = case shown="True" w1001 {
              tunnel: [w1002 w1004] -> w996
              tunnel: w997 -> [w1002 w1003]
              frame False {
              }
              frame True {
                w1005 = u16 6 ("id мишени")
                n584 = property on="id мишени" class="DigNum (strict)"(error in=w1003, "Value"=w1005) -> (error out=w1006:errorcluster)  [unwired: 1 in, 1 out]
                n585 = property on="id мишени" class="DigNum (strict)"(error in=w1006, "Val(Sgnl)"=w1005) -> (error out=w1004:errorcluster)  [unwired: 1 in, 1 out]
              }
            }
          }
        }
      }
      event "Мишень 7": Shortcut Menu Selection (User) {
        n586 = event-data() -> ("ItemTag"=w1009:string)  [unwired: 1 out]
        n587 = case shown="\"Настроить\", Default" w1009 {
          tunnel: w1007 -> [w1017 w1023]
          tunnel: [w1010 w1022] -> w1008
          frame "Настроить", Default {
            n588 = call "Настройки мишени (Sub VI).vi"("Параметры мишеней вх"="М7", "error in"=w1017) -> ("Параметры мишеней вых"=w1011:T1, "error out"=w1012:errorcluster)  [unwired: 16 in]
            n589 = Unbundle(w1011) -> ("Название мишени"=w1016:string, "Х0_position"=w1021:u16, "Y0_position"=w1020:u16, "Длина, мм"=w1019:u16, "Ширина, мм"=w1018:u16)  [unwired: 5 out]
            n590 = property on="М7" class="Clust (strict)"(error in=w1012, "Val(Sgnl)"=w1011) -> (error out=w1010:errorcluster)  [unwired: 1 in, 1 out]
            n591 = Bundle("Х0_position"=w1021, "Y0_position"=w1020) -> (w1015:cluster{"Х0_position":u16, "Y0_position":u16})  [unwired: 1 in]
            n592 = Bundle("Длина, мм"=w1019, "Ширина, мм"=w1018) -> (w1014:cluster{"Длина, мм":u16, "Ширина, мм":u16})  [unwired: 1 in]
            n593 = property on="Мишень 7" class="Pict"("TipStrip"=w1016) -> ()  [unwired: 2 in, 2 out]
            n594 = property on="Мишень 7" class="Pict"("Position"=w1015) -> ()  [unwired: 2 in, 2 out]
            n595 = property on="Мишень 7" class="Pict"("Draw Area Size"=w1014) -> ()  [unwired: 2 in, 2 out]
          }
          frame "Выбрать" {
            n596 = Two Button Dialog(message="Вы уверены, что хотите выбрать эту мишень?", 1:"Нет" ("F button name (\"Cancel\")"), 2:"Да" ("T button name (\"OK\")")) -> (T button?=w1027:bool)
            n597 = case shown="True" w1027 {
              tunnel: [w1028 w1030] -> w1022
              tunnel: w1023 -> [w1028 w1029]
              frame False {
              }
              frame True {
                w1031 = u16 7 ("id мишени")
                n598 = property on="id мишени" class="DigNum (strict)"(error in=w1029, "Value"=w1031) -> (error out=w1032:errorcluster)  [unwired: 1 in, 1 out]
                n599 = property on="id мишени" class="DigNum (strict)"(error in=w1032, "Val(Sgnl)"=w1031) -> (error out=w1030:errorcluster)  [unwired: 1 in, 1 out]
              }
            }
          }
        }
      }
      event "Мишень 8": Shortcut Menu Selection (User) {
        n600 = event-data() -> ("ItemTag"=w1035:string)  [unwired: 1 out]
        n601 = case shown="\"Настроить\", Default" w1035 {
          tunnel: w1033 -> [w1043 w1049]
          tunnel: [w1036 w1048] -> w1034
          frame "Настроить", Default {
            n602 = call "Настройки мишени (Sub VI).vi"("Параметры мишеней вх"="М8", "error in"=w1043) -> ("Параметры мишеней вых"=w1037:T1, "error out"=w1038:errorcluster)  [unwired: 16 in]
            n603 = Unbundle(w1037) -> ("Название мишени"=w1042:string, "Х0_position"=w1047:u16, "Y0_position"=w1046:u16, "Длина, мм"=w1045:u16, "Ширина, мм"=w1044:u16)  [unwired: 5 out]
            n604 = property on="М8" class="Clust (strict)"(error in=w1038, "Val(Sgnl)"=w1037) -> (error out=w1036:errorcluster)  [unwired: 1 in, 1 out]
            n605 = Bundle("Х0_position"=w1047, "Y0_position"=w1046) -> (w1041:cluster{"Х0_position":u16, "Y0_position":u16})  [unwired: 1 in]
            n606 = Bundle("Длина, мм"=w1045, "Ширина, мм"=w1044) -> (w1040:cluster{"Длина, мм":u16, "Ширина, мм":u16})  [unwired: 1 in]
            n607 = property on="Мишень 8" class="Pict"("TipStrip"=w1042) -> ()  [unwired: 2 in, 2 out]
            n608 = property on="Мишень 8" class="Pict"("Position"=w1041) -> ()  [unwired: 2 in, 2 out]
            n609 = property on="Мишень 8" class="Pict"("Draw Area Size"=w1040) -> ()  [unwired: 2 in, 2 out]
          }
          frame "Выбрать" {
            n610 = Two Button Dialog(message="Вы уверены, что хотите выбрать эту мишень?", 1:"Нет" ("F button name (\"Cancel\")"), 2:"Да" ("T button name (\"OK\")")) -> (T button?=w1053:bool)
            n611 = case shown="True" w1053 {
              tunnel: [w1054 w1056] -> w1048
              tunnel: w1049 -> [w1054 w1055]
              frame False {
              }
              frame True {
                w1057 = u16 8 ("id мишени")
                n612 = property on="id мишени" class="DigNum (strict)"(error in=w1055, "Value"=w1057) -> (error out=w1058:errorcluster)  [unwired: 1 in, 1 out]
                n613 = property on="id мишени" class="DigNum (strict)"(error in=w1058, "Val(Sgnl)"=w1057) -> (error out=w1056:errorcluster)  [unwired: 1 in, 1 out]
              }
            }
          }
        }
      }
      event "Мишень 9": Shortcut Menu Selection (User) {
        n614 = event-data() -> ("ItemTag"=w1061:string)  [unwired: 1 out]
        n615 = case shown="\"Настроить\", Default" w1061 {
          tunnel: w1059 -> [w1069 w1075]
          tunnel: [w1062 w1074] -> w1060
          frame "Настроить", Default {
            n616 = call "Настройки мишени (Sub VI).vi"("Параметры мишеней вх"="М9", "error in"=w1069) -> ("Параметры мишеней вых"=w1063:T1, "error out"=w1064:errorcluster)  [unwired: 16 in]
            n617 = Unbundle(w1063) -> ("Название мишени"=w1068:string, "Х0_position"=w1073:u16, "Y0_position"=w1072:u16, "Длина, мм"=w1071:u16, "Ширина, мм"=w1070:u16)  [unwired: 5 out]
            n618 = property on="М9" class="Clust (strict)"(error in=w1064, "Val(Sgnl)"=w1063) -> (error out=w1062:errorcluster)  [unwired: 1 in, 1 out]
            n619 = Bundle("Х0_position"=w1073, "Y0_position"=w1072) -> (w1067:cluster{"Х0_position":u16, "Y0_position":u16})  [unwired: 1 in]
            n620 = Bundle("Длина, мм"=w1071, "Ширина, мм"=w1070) -> (w1066:cluster{"Длина, мм":u16, "Ширина, мм":u16})  [unwired: 1 in]
            n621 = property on="Мишень 9" class="Pict"("TipStrip"=w1068) -> ()  [unwired: 2 in, 2 out]
            n622 = property on="Мишень 9" class="Pict"("Position"=w1067) -> ()  [unwired: 2 in, 2 out]
            n623 = property on="Мишень 9" class="Pict"("Draw Area Size"=w1066) -> ()  [unwired: 2 in, 2 out]
          }
          frame "Выбрать" {
            n624 = Two Button Dialog(message="Вы уверены, что хотите выбрать эту мишень?", 1:"Нет" ("F button name (\"Cancel\")"), 2:"Да" ("T button name (\"OK\")")) -> (T button?=w1079:bool)
            n625 = case shown="True" w1079 {
              tunnel: [w1080 w1082] -> w1074
              tunnel: w1075 -> [w1080 w1081]
              frame False {
              }
              frame True {
                w1083 = u16 9 ("id мишени")
                n626 = property on="id мишени" class="DigNum (strict)"(error in=w1081, "Value"=w1083) -> (error out=w1084:errorcluster)  [unwired: 1 in, 1 out]
                n627 = property on="id мишени" class="DigNum (strict)"(error in=w1084, "Val(Sgnl)"=w1083) -> (error out=w1082:errorcluster)  [unwired: 1 in, 1 out]
              }
            }
          }
        }
      }
      event "Мишень 10": Shortcut Menu Selection (User) {
        n628 = event-data() -> ("ItemTag"=w1087:string)  [unwired: 1 out]
        n629 = case shown="\"Настроить\", Default" w1087 {
          tunnel: w1085 -> [w1095 w1101]
          tunnel: [w1088 w1100] -> w1086
          frame "Настроить", Default {
            n630 = call "Настройки мишени (Sub VI).vi"("Параметры мишеней вх"="М10", "error in"=w1095) -> ("Параметры мишеней вых"=w1089:T1, "error out"=w1090:errorcluster)  [unwired: 16 in]
            n631 = Unbundle(w1089) -> ("Название мишени"=w1094:string, "Х0_position"=w1099:u16, "Y0_position"=w1098:u16, "Длина, мм"=w1097:u16, "Ширина, мм"=w1096:u16)  [unwired: 5 out]
            n632 = property on="М10" class="Clust (strict)"(error in=w1090, "Val(Sgnl)"=w1089) -> (error out=w1088:errorcluster)  [unwired: 1 in, 1 out]
            n633 = Bundle("Х0_position"=w1099, "Y0_position"=w1098) -> (w1093:cluster{"Х0_position":u16, "Y0_position":u16})  [unwired: 1 in]
            n634 = Bundle("Длина, мм"=w1097, "Ширина, мм"=w1096) -> (w1092:cluster{"Длина, мм":u16, "Ширина, мм":u16})  [unwired: 1 in]
            n635 = property on="Мишень 10" class="Pict"("TipStrip"=w1094) -> ()  [unwired: 2 in, 2 out]
            n636 = property on="Мишень 10" class="Pict"("Position"=w1093) -> ()  [unwired: 2 in, 2 out]
            n637 = property on="Мишень 10" class="Pict"("Draw Area Size"=w1092) -> ()  [unwired: 2 in, 2 out]
          }
          frame "Выбрать" {
            n638 = Two Button Dialog(message="Вы уверены, что хотите выбрать эту мишень?", 1:"Нет" ("F button name (\"Cancel\")"), 2:"Да" ("T button name (\"OK\")")) -> (T button?=w1105:bool)
            n639 = case shown="True" w1105 {
              tunnel: [w1106 w1108] -> w1100
              tunnel: w1101 -> [w1106 w1107]
              frame False {
              }
              frame True {
                w1109 = u16 10 ("id мишени")
                n640 = property on="id мишени" class="DigNum (strict)"(error in=w1107, "Value"=w1109) -> (error out=w1110:errorcluster)  [unwired: 1 in, 1 out]
                n641 = property on="id мишени" class="DigNum (strict)"(error in=w1110, "Val(Sgnl)"=w1109) -> (error out=w1108:errorcluster)  [unwired: 1 in, 1 out]
              }
            }
          }
        }
      }
      event "id мишени", "Выстрелов до перемотки пленки", "М1", "М2", "М3", "М4", "М5", "М6", "М7", "М8", "М9", "М10": Value Change {
        # "обновление информации по мишеням"
        n642 = event-data() -> ()  [unwired: 2 out]
        n643 = local read "id мишени"() -> (w1112:u16)
        n644 = property on="Осталось:" class="Slide (strict)"(error in=w1113) -> (error out=w1114:errorcluster, "Value"=w1116:u16)  [unwired: 1 in, 1 out]
        n645 = case shown="1" w1112 {
          selector: w1112 -> [w1124 w1127 w1130 w1133 w1136 w1139 w1142 w1145 w1148 w1151]
          tunnel: [w1125 w1128 w1131 w1134 w1137 w1140 w1143 w1146 w1149 w1152] -> w1121
          tunnel: [w1124 w1127 w1130 w1133 w1136 w1139 w1142 w1145 w1148 w1151] -> w1122
          tunnel: [w1123 w1126 w1129 w1132 w1135 w1138 w1141 w1144 w1147 w1150] -> w1111
          frame 1 {
            n646 = property on="Мишень 1" class="Pict"() -> ("TipStrip"=w1123:string)  [unwired: 2 in, 2 out]
            n647 = property on="Выстрелов осталось M1" class="DigNum (strict)"() -> ("Value"=w1125:u16)  [unwired: 2 in, 2 out]
          }
          frame 2, Default {
            n648 = property on="Мишень 2" class="Pict"() -> ("TipStrip"=w1126:string)  [unwired: 2 in, 2 out]
            n649 = property on="Выстрелов осталось M2" class="DigNum (strict)"() -> ("Value"=w1128:u16)  [unwired: 2 in, 2 out]
          }
          frame 3 {
            n650 = property on="Мишень 3" class="Pict"() -> ("TipStrip"=w1129:string)  [unwired: 2 in, 2 out]
            n651 = property on="Выстрелов осталось M3" class="DigNum (strict)"() -> ("Value"=w1131:u16)  [unwired: 2 in, 2 out]
          }
          frame 4 {
            n652 = property on="Мишень 4" class="Pict"() -> ("TipStrip"=w1132:string)  [unwired: 2 in, 2 out]
            n653 = property on="Выстрелов осталось M4" class="DigNum (strict)"() -> ("Value"=w1134:u16)  [unwired: 2 in, 2 out]
          }
          frame 5 {
            n654 = property on="Мишень 5" class="Pict"() -> ("TipStrip"=w1135:string)  [unwired: 2 in, 2 out]
            n655 = property on="Выстрелов осталось M5" class="DigNum (strict)"() -> ("Value"=w1137:u16)  [unwired: 2 in, 2 out]
          }
          frame 6 {
            n656 = property on="Мишень 6" class="Pict"() -> ("TipStrip"=w1138:string)  [unwired: 2 in, 2 out]
            n657 = property on="Выстрелов осталось M6" class="DigNum (strict)"() -> ("Value"=w1140:u16)  [unwired: 2 in, 2 out]
          }
          frame 7 {
            n658 = property on="Мишень 7" class="Pict"() -> ("TipStrip"=w1141:string)  [unwired: 2 in, 2 out]
            n659 = property on="Выстрелов осталось M7" class="DigNum (strict)"() -> ("Value"=w1143:u16)  [unwired: 2 in, 2 out]
          }
          frame 8 {
            n660 = property on="Мишень 8" class="Pict"() -> ("TipStrip"=w1144:string)  [unwired: 2 in, 2 out]
            n661 = property on="Выстрелов осталось M8" class="DigNum (strict)"() -> ("Value"=w1146:u16)  [unwired: 2 in, 2 out]
          }
          frame 9 {
            n662 = property on="Мишень 9" class="Pict"() -> ("TipStrip"=w1147:string)  [unwired: 2 in, 2 out]
            n663 = property on="Выстрелов осталось M9" class="DigNum (strict)"() -> ("Value"=w1149:u16)  [unwired: 2 in, 2 out]
          }
          frame 10 {
            n664 = property on="Мишень 10" class="Pict"() -> ("TipStrip"=w1150:string)  [unwired: 2 in, 2 out]
            n665 = property on="Выстрелов осталось M10" class="DigNum (strict)"() -> ("Value"=w1152:u16)  [unwired: 2 in, 2 out]
          }
        }
        "Текущая мишень:" <- w1111
        n666 = property on="Выстрелов до перемотки пленки" class="DigNum (strict)"(error in=w1114) -> (error out=w1115:errorcluster, "Value"=w1117:u16)  [unwired: 1 in, 1 out]
        n667 = property on="TCP con ID" class="Ref (strict)"(error in=w1115) -> (error out=w1118:errorcluster, "Value"=w1119:refnum<k5>)  [unwired: 1 in, 1 out]
        n668 = call "Команда обмена 85 (обновление парам. мишени с  id ) (SubVI).vi"("id мишени"=w1122, "Выстрелов осталось"=w1121, "error in"=w1118, "TCP connection ID"=w1119, "Выстрелов до перемотки"=w1117, "До перемотки осталось"=w1116) -> ("error out"=w1120:errorcluster)  [unwired: 21 in]
      }
      event "Шаг вперед": Value Change {
        n669 = event-data() -> ("OldVal"=w1157:bool)  [unwired: 1 out]
        n670 = local write "Шаг вперед"(w1157) -> ()
        n671 = property on="TCP con ID" class="Ref (strict)"(error in=w1154) -> (error out=w1156:errorcluster, "Value"=w1155:refnum<k5>)  [unwired: 1 in, 1 out]
        n672 = call "Команда обмена 86 (принудительный шаг вперед ) (SubVI).vi"("error in"=w1156, "TCP connection ID"=w1155) -> ("error out"=w1153:errorcluster)  [unwired: 25 in]
      }
      event "Фокус +": Value Change {
        n673 = event-data() -> ("OldVal"=w1158:bool)  [unwired: 1 out]
        n674 = local write "Фокус +"(w1158) -> ()
        n675 = property on="TCP con ID" class="Ref (strict)"(error in=w1162) -> (error out=w1160:errorcluster, "Value"=w1161:refnum<k5>)  [unwired: 1 in, 1 out]
        n676 = call "Команда обмена 87 (фокус +) (SubVI).vi"("error in"=w1160, "TCP connection ID"=w1161) -> ("error out"=w1159:errorcluster)  [unwired: 25 in]
      }
      event "Фокус --": Value Change {
        n677 = event-data() -> ("OldVal"=w1166:bool)  [unwired: 1 out]
        n678 = local write "Фокус --"(w1166) -> ()
        n679 = property on="TCP con ID" class="Ref (strict)"(error in=w1167) -> (error out=w1164:errorcluster, "Value"=w1165:refnum<k5>)  [unwired: 1 in, 1 out]
        n680 = call "Команда обмена 88 (фокус -) (SubVI).vi"("error in"=w1164, "TCP connection ID"=w1165) -> ("error out"=w1163:errorcluster)  [unwired: 25 in]
      }
      event "Перемотка пленки": Value Change {
        n681 = event-data() -> ("OldVal"=w1171:bool)  [unwired: 1 out]
        n682 = local write "Перемотка пленки"(w1171) -> ()
        n683 = property on="TCP con ID" class="Ref (strict)"(error in=w1172) -> (error out=w1169:errorcluster, "Value"=w1170:refnum<k5>)  [unwired: 1 in, 1 out]
        n684 = call "Команда обмена 89 (перемотка пленки) (SubVI).vi"("error in"=w1169, "TCP connection ID"=w1170) -> ("error out"=w1168:errorcluster)  [unwired: 25 in]
      }
      event "UpButton": Value Change {
        # "Ручной сдвиг мишени вверх"
        n685 = event-data() -> ("OldVal"=w1183:bool)  [unwired: 1 out]
        n686 = local write "UpButton"(w1183) -> ()
        n687 = property on="id мишени" class="DigNum (strict)"() -> ("Value"=w1179:u16)  [unwired: 2 in, 2 out]
        n688 = case shown="1, Default" w1179 {
          tunnel: [w1187 w1190 w1193 w1196 w1199 w1202 w1205 w1208 w1211 w1214] -> w1174
          tunnel: w1178 -> [w1187 w1190 w1193 w1196 w1199 w1202 w1205 w1208 w1211 w1214]
          tunnel: [w1186 w1189 w1192 w1195 w1198 w1201 w1204 w1207 w1210 w1213] -> w1177
          tunnel: w1176 -> [w1186 w1189 w1192 w1195 w1198 w1201 w1204 w1207 w1210 w1213]
          tunnel: [w1185 w1188 w1191 w1194 w1197 w1200 w1203 w1206 w1209 w1212] -> w1175
          frame 4 {
            n689 = control-ref of="Мишень 4"() -> (w1185:refnum<vi>)
          }
          frame 3 {
            n690 = control-ref of="Мишень 3"() -> (w1188:refnum<vi>)
          }
          frame 2 {
            n691 = control-ref of="Мишень 2"() -> (w1191:refnum<vi>)
          }
          frame 1, Default {
            n692 = control-ref of="Мишень 1"() -> (w1194:refnum<vi>)
          }
          frame 6 {
            n693 = control-ref of="Мишень 6"() -> (w1197:refnum<vi>)
          }
          frame 7 {
            n694 = control-ref of="Мишень 7"() -> (w1200:refnum<vi>)
          }
          frame 8 {
            n695 = control-ref of="Мишень 8"() -> (w1203:refnum<vi>)
          }
          frame 9 {
            n696 = control-ref of="Мишень 9"() -> (w1206:refnum<vi>)
          }
          frame 10 {
            n697 = control-ref of="Мишень 10"() -> (w1209:refnum<vi>)
          }
          frame 5 {
            n698 = control-ref of="Мишень 5"() -> (w1212:refnum<vi>)
          }
        }
        n699 = control-ref of="XY лазера"() -> (w1180:refnum<vi>)
        n700 = call "Анализ выхода за границы мишени (SubVI).vi"("Ref мишени"=w1175, "Ref XY лазера"=w1180, "error in"=w1177, "Шаг перехода"=w1174) -> ("Шаг перехода вых"=w1173:string, "вышел за рамки сверху"=w1181:bool, "error out"=w1182:errorcluster)  [unwired: 10 in, 3 out]
        n701 = case shown="False" w1181 {
          tunnel: [w1219 w1220] -> w1184
          tunnel: w1182 -> [w1216 w1220]
          tunnel: w1173 -> [w1215 _]
          frame False {
            n702 = property on="TCP con ID" class="Ref (strict)"(error in=w1216) -> (error out=w1218:errorcluster, "Value"=w1217:refnum<k5>)  [unwired: 1 in, 1 out]
            n703 = call "Команда обмена 70 (ручное упр. ВВЕРХ) (SubVI).vi"("Шаг перехода"=w1215, "error in"=w1218, "TCP connection ID"=w1217) -> ("error out"=w1219:errorcluster)  [unwired: 24 in]
          }
          frame True {
          }
        }
      }
      event "DownButton": Value Change {
        # "Ручной сдвиг мишени вниз"
        n704 = event-data() -> ("OldVal"=w1232:bool)  [unwired: 1 out]
        n705 = local write "DownButton"(w1232) -> ()
        n706 = property on="id мишени" class="DigNum (strict)"() -> ("Value"=w1229:u16)  [unwired: 2 in, 2 out]
        n707 = case shown="1, Default" w1229 {
          tunnel: [w1235 w1238 w1241 w1244 w1247 w1250 w1253 w1256 w1259 w1262] -> w1222
          tunnel: w1228 -> [w1235 w1238 w1241 w1244 w1247 w1250 w1253 w1256 w1259 w1262]
          tunnel: [w1234 w1237 w1240 w1243 w1246 w1249 w1252 w1255 w1258 w1261] -> w1227
          tunnel: w1226 -> [w1234 w1237 w1240 w1243 w1246 w1249 w1252 w1255 w1258 w1261]
          tunnel: [w1233 w1236 w1239 w1242 w1245 w1248 w1251 w1254 w1257 w1260] -> w1225
          frame 4 {
            n708 = control-ref of="Мишень 4"() -> (w1233:refnum<vi>)
          }
          frame 3 {
            n709 = control-ref of="Мишень 3"() -> (w1236:refnum<vi>)
          }
          frame 2 {
            n710 = control-ref of="Мишень 2"() -> (w1239:refnum<vi>)
          }
          frame 1, Default {
            n711 = control-ref of="Мишень 1"() -> (w1242:refnum<vi>)
          }
          frame 6 {
            n712 = control-ref of="Мишень 6"() -> (w1245:refnum<vi>)
          }
          frame 7 {
            n713 = control-ref of="Мишень 7"() -> (w1248:refnum<vi>)
          }
          frame 8 {
            n714 = control-ref of="Мишень 8"() -> (w1251:refnum<vi>)
          }
          frame 9 {
            n715 = control-ref of="Мишень 9"() -> (w1254:refnum<vi>)
          }
          frame 10 {
            n716 = control-ref of="Мишень 10"() -> (w1257:refnum<vi>)
          }
          frame 5 {
            n717 = control-ref of="Мишень 5"() -> (w1260:refnum<vi>)
          }
        }
        n718 = control-ref of="XY лазера"() -> (w1230:refnum<vi>)
        n719 = call "Анализ выхода за границы мишени (SubVI).vi"("Ref мишени"=w1225, "Ref XY лазера"=w1230, "error in"=w1227, "Шаг перехода"=w1222) -> ("Шаг перехода вых"=w1221:string, "вышел за рамки снизу"=w1224:bool, "error out"=w1231:errorcluster)  [unwired: 10 in, 3 out]
        n720 = case shown="False" w1224 {
          tunnel: [w1267 w1268] -> w1223
          tunnel: w1231 -> [w1264 w1268]
          tunnel: w1221 -> [w1263 _]
          frame False {
            n721 = property on="TCP con ID" class="Ref (strict)"(error in=w1264) -> (error out=w1266:errorcluster, "Value"=w1265:refnum<k5>)  [unwired: 1 in, 1 out]
            n722 = call "Команда обмена 71 (ручное упр. ВНИЗ) (SubVI).vi"("Шаг перехода"=w1263, "error in"=w1266, "TCP connection ID"=w1265) -> ("error out"=w1267:errorcluster)  [unwired: 24 in]
          }
          frame True {
          }
        }
      }
      event "LeftButton": Value Change {
        # "Ручной сдвиг мишени влево"
        n723 = event-data() -> ("OldVal"=w1271:bool)  [unwired: 1 out]
        n724 = local write "LeftButton"(w1271) -> ()
        n725 = property on="id мишени" class="DigNum (strict)"() -> ("Value"=w1277:u16)  [unwired: 2 in, 2 out]
        n726 = case shown="1, Default" w1277 {
          tunnel: [w1283 w1286 w1289 w1292 w1295 w1298 w1301 w1304 w1307 w1310] -> w1270
          tunnel: w1276 -> [w1283 w1286 w1289 w1292 w1295 w1298 w1301 w1304 w1307 w1310]
          tunnel: [w1282 w1285 w1288 w1291 w1294 w1297 w1300 w1303 w1306 w1309] -> w1275
          tunnel: w1274 -> [w1282 w1285 w1288 w1291 w1294 w1297 w1300 w1303 w1306 w1309]
          tunnel: [w1281 w1284 w1287 w1290 w1293 w1296 w1299 w1302 w1305 w1308] -> w1273
          frame 4 {
            n727 = control-ref of="Мишень 4"() -> (w1281:refnum<vi>)
          }
          frame 3 {
            n728 = control-ref of="Мишень 3"() -> (w1284:refnum<vi>)
          }
          frame 2 {
            n729 = control-ref of="Мишень 2"() -> (w1287:refnum<vi>)
          }
          frame 1, Default {
            n730 = control-ref of="Мишень 1"() -> (w1290:refnum<vi>)
          }
          frame 6 {
            n731 = control-ref of="Мишень 6"() -> (w1293:refnum<vi>)
          }
          frame 7 {
            n732 = control-ref of="Мишень 7"() -> (w1296:refnum<vi>)
          }
          frame 8 {
            n733 = control-ref of="Мишень 8"() -> (w1299:refnum<vi>)
          }
          frame 9 {
            n734 = control-ref of="Мишень 9"() -> (w1302:refnum<vi>)
          }
          frame 10 {
            n735 = control-ref of="Мишень 10"() -> (w1305:refnum<vi>)
          }
          frame 5 {
            n736 = control-ref of="Мишень 5"() -> (w1308:refnum<vi>)
          }
        }
        n737 = control-ref of="XY лазера"() -> (w1278:refnum<vi>)
        n738 = call "Анализ выхода за границы мишени (SubVI).vi"("Ref мишени"=w1273, "Ref XY лазера"=w1278, "error in"=w1275, "Шаг перехода"=w1270) -> ("Шаг перехода вых"=w1269:string, "вышел за рамки слева"=w1272:bool, "error out"=w1279:errorcluster)  [unwired: 10 in, 3 out]
        n739 = case shown="False" w1272 {
          tunnel: [w1315 w1316] -> w1280
          tunnel: w1279 -> [w1312 w1316]
          tunnel: w1269 -> [w1311 _]
          frame False {
            n740 = property on="TCP con ID" class="Ref (strict)"(error in=w1312) -> (error out=w1314:errorcluster, "Value"=w1313:refnum<k5>)  [unwired: 1 in, 1 out]
            n741 = call "Команда обмена 72 (ручное упр. ВЛЕВО) (SubVI).vi"("Шаг перехода"=w1311, "error in"=w1314, "TCP connection ID"=w1313) -> ("error out"=w1315:errorcluster)  [unwired: 24 in]
          }
          frame True {
          }
        }
      }
      event "RightButton": Value Change {
        # "Ручной сдвиг мишени влево"
        n742 = event-data() -> ("OldVal"=w1320:bool)  [unwired: 1 out]
        n743 = local write "RightButton"(w1320) -> ()
        n744 = property on="id мишени" class="DigNum (strict)"() -> ("Value"=w1325:u16)  [unwired: 2 in, 2 out]
        n745 = case shown="1, Default" w1325 {
          tunnel: [w1331 w1334 w1337 w1340 w1343 w1346 w1349 w1352 w1355 w1358] -> w1318
          tunnel: w1324 -> [w1331 w1334 w1337 w1340 w1343 w1346 w1349 w1352 w1355 w1358]
          tunnel: [w1330 w1333 w1336 w1339 w1342 w1345 w1348 w1351 w1354 w1357] -> w1323
          tunnel: w1322 -> [w1330 w1333 w1336 w1339 w1342 w1345 w1348 w1351 w1354 w1357]
          tunnel: [w1329 w1332 w1335 w1338 w1341 w1344 w1347 w1350 w1353 w1356] -> w1321
          frame 4 {
            n746 = control-ref of="Мишень 4"() -> (w1329:refnum<vi>)
          }
          frame 3 {
            n747 = control-ref of="Мишень 3"() -> (w1332:refnum<vi>)
          }
          frame 2 {
            n748 = control-ref of="Мишень 2"() -> (w1335:refnum<vi>)
          }
          frame 1, Default {
            n749 = control-ref of="Мишень 1"() -> (w1338:refnum<vi>)
          }
          frame 6 {
            n750 = control-ref of="Мишень 6"() -> (w1341:refnum<vi>)
          }
          frame 7 {
            n751 = control-ref of="Мишень 7"() -> (w1344:refnum<vi>)
          }
          frame 8 {
            n752 = control-ref of="Мишень 8"() -> (w1347:refnum<vi>)
          }
          frame 9 {
            n753 = control-ref of="Мишень 9"() -> (w1350:refnum<vi>)
          }
          frame 10 {
            n754 = control-ref of="Мишень 10"() -> (w1353:refnum<vi>)
          }
          frame 5 {
            n755 = control-ref of="Мишень 5"() -> (w1356:refnum<vi>)
          }
        }
        n756 = control-ref of="XY лазера"() -> (w1326:refnum<vi>)
        n757 = call "Анализ выхода за границы мишени (SubVI).vi"("Ref мишени"=w1321, "Ref XY лазера"=w1326, "error in"=w1323, "Шаг перехода"=w1318) -> ("Шаг перехода вых"=w1317:string, "вышел за рамки справа"=w1319:bool, "error out"=w1327:errorcluster)  [unwired: 10 in, 3 out]
        n758 = case shown="False" w1319 {
          tunnel: [w1363 w1364] -> w1328
          tunnel: w1327 -> [w1360 w1364]
          tunnel: w1317 -> [w1359 _]
          frame False {
            n759 = property on="TCP con ID" class="Ref (strict)"(error in=w1360) -> (error out=w1362:errorcluster, "Value"=w1361:refnum<k5>)  [unwired: 1 in, 1 out]
            n760 = call "Команда обмена 73 (ручное упр. ВПРАВО) (SubVI).vi"("Шаг перехода"=w1359, "error in"=w1362, "TCP connection ID"=w1361) -> ("error out"=w1363:errorcluster)  [unwired: 24 in]
          }
          frame True {
          }
        }
      }
      event "Конфигурация сохранена": Value Change {
        # "Сохранение конфигурации"
        n761 = event-data() -> ("OldVal"=w1368:bool)  [unwired: 1 out]
        n762 = flat-sequence {
          tunnel: w1368 -> [w1460]
          tunnel: w1367 -> [w1459]
          tunnel: [w1372] -> w1365
          tunnel: [w1479] -> w1366
          tunnel: w1365 -> [w1479]
          frame #0 {
            n763 = property on="Конфигурация сохранена" class="Bool (strict)"(error in=w1459, "Value"=w1460) -> (error out=w1429:errorcluster)  [unwired: 1 in, 1 out]
            n764 = local read "М10"() -> (w1449:T1)
            n765 = local read "выстрел X М1"() -> (w1408:u16)
            n766 = local read "выстрел Y М1"() -> (w1407:u16)
            n767 = local read "выстрел X М2"() -> (w1406:u16)
            n768 = local read "выстрел X М3"() -> (w1404:u16)
            n769 = local read "М1"() -> (w1458:T1)
            n770 = local read "М2"() -> (w1457:T1)
            n771 = local read "М3"() -> (w1456:T1)
            n772 = local read "М4"() -> (w1455:T1)
            n773 = local read "М5"() -> (w1454:T1)
            n774 = local read "М6"() -> (w1453:T1)
            n775 = local read "М7"() -> (w1452:T1)
            n776 = local read "М8"() -> (w1451:T1)
            n777 = local read "М9"() -> (w1450:T1)
            n778 = local read "выстрел Y М2"() -> (w1405:u16)
            n779 = local read "выстрел Y М3"() -> (w1403:u16)
            n780 = local read "выстрел X М4"() -> (w1402:u16)
            n781 = local read "выстрел X М5"() -> (w1400:u16)
            n782 = local read "выстрел Y М4"() -> (w1401:u16)
            n783 = local read "выстрел Y М5"() -> (w1399:u16)
            n784 = property on="Мишень 1" class="Pict"(error in=w1429) -> (error out=w1430:errorcluster, "Visible"=w1427:bool)  [unwired: 1 in, 1 out]
            n785 = property on="Мишень 2" class="Pict"(error in=w1430) -> (error out=w1431:errorcluster, "Visible"=w1426:bool)  [unwired: 1 in, 1 out]
            n786 = Bundle("М1"=w1458, "М2"=w1457, "М3"=w1456, "М4"=w1455, "М5"=w1454, "М6"=w1453, "М7"=w1452, "М8"=w1451, "М9"=w1450, "М10"=w1449) -> (w1385:T9)  [unwired: 1 in]
            n787 = Bundle("выстрел X М1"=w1408, "выстрел Y М1"=w1407, "выстрел X М2"=w1406, "выстрел Y М2"=w1405, "выстрел X М3"=w1404, "выстрел Y М3"=w1403, "выстрел X М4"=w1402, "выстрел Y М4"=w1401, "выстрел X М5"=w1400, "выстрел Y М5"=w1399) -> (w1377:T10)  [unwired: 1 in]
            n788 = property on="Мишень 3" class="Pict"(error in=w1431) -> (error out=w1432:errorcluster, "Visible"=w1425:bool)  [unwired: 1 in, 1 out]
            n789 = property on="Мишень 4" class="Pict"(error in=w1432) -> (error out=w1433:errorcluster, "Visible"=w1424:bool)  [unwired: 1 in, 1 out]
            n790 = local read "выстрел X М10"() -> (w1390:u16)
            n791 = local read "выстрел X М6"() -> (w1398:u16)
            n792 = local read "выстрел Y М10"() -> (w1389:u16)
            n793 = local read "Знак перех. dX М1"() -> (w1448:i8)
            n794 = local read "Знак перех. dX М2"() -> (w1447:i8)
            n795 = local read "Знак перех. dX М3"() -> (w1446:i8)
            n796 = local read "Знак перех. dX М4"() -> (w1445:i8)
            n797 = local read "Знак перех. dX М5"() -> (w1444:i8)
            n798 = local read "Знак перех. dX М6"() -> (w1443:i8)
            n799 = local read "Знак перех. dX М7"() -> (w1442:i8)
            n800 = local read "Знак перех. dX М8"() -> (w1441:i8)
            n801 = local read "Знак перех. dX М9"() -> (w1440:i8)
            n802 = local read "Знак перех. dX М10"() -> (w1439:i8)
            n803 = local read "выстрел Y М6"() -> (w1397:u16)
            n804 = local read "выстрел X М7"() -> (w1396:u16)
            n805 = local read "выстрел X М8"() -> (w1394:u16)
            n806 = local read "выстрел Y М7"() -> (w1395:u16)
            n807 = local read "выстрел Y М8"() -> (w1393:u16)
            n808 = local read "выстрел X М9"() -> (w1392:u16)
            n809 = local read "выстрел Y М9"() -> (w1391:u16)
            n810 = property on="Мишень 5" class="Pict"(error in=w1433) -> (error out=w1438:errorcluster, "Visible"=w1423:bool)  [unwired: 1 in, 1 out]
            n811 = property on="Мишень 6" class="Pict"(error in=w1438) -> (error out=w1437:errorcluster, "Visible"=w1422:bool)  [unwired: 1 in, 1 out]
            n812 = Bundle("выстрел X М6"=w1398, "выстрел Y М6"=w1397, "выстрел X М7"=w1396, "выстрел Y М7"=w1395, "выстрел X М8"=w1394, "выстрел Y М8"=w1393, "выстрел X М9"=w1392, "выстрел Y М9"=w1391, "выстрел X М10"=w1390, "выстрел Y М10"=w1389) -> (w1378:T11)  [unwired: 1 in]
            n813 = property on="Мишень 7" class="Pict"(error in=w1437) -> (error out=w1436:errorcluster, "Visible"=w1421:bool)  [unwired: 1 in, 1 out]
            n814 = Bundle("Знак перех. dX М1"=w1448, "Знак перех. dX М2"=w1447, "Знак перех. dX М3"=w1446, "Знак перех. dX М4"=w1445, "Знак перех. dX М5"=w1444, "Знак перех. dX М6"=w1443, "Знак перех. dX М7"=w1442, "Знак перех. dX М8"=w1441, "Знак перех. dX М9"=w1440, "Знак перех. dX М10"=w1439) -> (w1386:T12)  [unwired: 1 in]
            n815 = disable-structure shown="Disabled" {
              disable-tunnel: [w1462 _] -> w1376
              frame Disabled {
                n816 = local read "Мишень 1"() -> (w1472:picture)
                n817 = local read "Мишень 2"() -> (w1471:picture)
                n818 = local read "Мишень 3"() -> (w1470:picture)
                n819 = local read "Мишень 4"() -> (w1469:picture)
                n820 = local read "Мишень 5"() -> (w1468:picture)
                n821 = local read "Мишень 6"() -> (w1467:picture)
                n822 = local read "Мишень 7"() -> (w1466:picture)
                n823 = local read "Мишень 8"() -> (w1465:picture)
                n824 = local read "Мишень 9"() -> (w1464:picture)
                n825 = local read "Мишень 10"() -> (w1463:picture)
                n826 = Bundle("Мишень 1"=w1472, "Мишень 2"=w1471, "Мишень 3"=w1470, "Мишень 4"=w1469, "Мишень 5"=w1468, "Мишень 6"=w1467, "Мишень 7"=w1466, "Мишень 8"=w1465, "Мишень 9"=w1464, "Мишень 10"=w1463) -> (w1462:T13)  [unwired: 1 in]
              }
              frame Enabled {
              }
            }
            n827 = property on="Мишень 8" class="Pict"(error in=w1436) -> (error out=w1435:errorcluster, "Visible"=w1420:bool)  [unwired: 1 in, 1 out]
            n828 = property on="Мишень 9" class="Pict"(error in=w1435) -> (error out=w1434:errorcluster, "Visible"=w1419:bool)  [unwired: 1 in, 1 out]
            n829 = local read "Выстрелов осталось M1"() -> (w1418:u16)
            n830 = local read "Выстрелов осталось M2"() -> (w1417:u16)
            n831 = local read "Выстрелов осталось M3"() -> (w1416:u16)
            n832 = local read "Выстрелов осталось M4"() -> (w1415:u16)
            n833 = local read "Выстрелов осталось M5"() -> (w1414:u16)
            n834 = local read "Выстрелов осталось M6"() -> (w1413:u16)
            n835 = local read "Выстрелов осталось M7"() -> (w1412:u16)
            n836 = local read "Выстрелов осталось M8"() -> (w1411:u16)
            n837 = local read "Выстрелов осталось M9"() -> (w1410:u16)
            n838 = local read "Выстрелов осталось M10"() -> (w1409:u16)
            n839 = property on="Мишень 10" class="Pict"(error in=w1434) -> (error out=w1383:errorcluster, "Visible"=w1428:bool)  [unwired: 1 in, 1 out]
            n840 = Bundle("Visible"=w1427, "Visible"=w1426, "Visible"=w1425, "Visible"=w1424, "Visible"=w1423, "Visible"=w1422, "Visible"=w1421, "Visible"=w1420, "Visible"=w1419, "Visible"=w1428) -> (w1384:T14)  [unwired: 1 in]
            n841 = property on="текущ. инфо" class="Bool (strict)"(error in=w1383) -> (error out=w1382:errorcluster, "Position"=w1381:T4)  [unwired: 1 in, 1 out]
            n842 = Bundle("Выстрелов осталось M1"=w1418, "Выстрелов осталось M2"=w1417, "Выстрелов осталось M3"=w1416, "Выстрелов осталось M4"=w1415, "Выстрелов осталось M5"=w1414, "Выстрелов осталось M6"=w1413, "Выстрелов осталось M7"=w1412, "Выстрелов осталось M8"=w1411, "Выстрелов осталось M9"=w1410, "Выстрелов осталось M10"=w1409) -> (w1388:T15)  [unwired: 1 in]
            n843 = property on="XY лазера" class="Bool (strict)"(error in=w1382) -> (error out=w1379:errorcluster, "Position"=w1380:T4)  [unwired: 1 in, 1 out]
            n844 = local read "id мишени"() -> (w1387:u16)
            n845 = local read "Флаг резерв. сохр."() -> (w1369:bool)
            n846 = call "Фиксироание всех параметров (SubVI).vi"("Параметры всех мишеней"=w1385, "Видимость мишеней"=w1384, "error in"=w1379, "полож. красной точки лазера"=w1380, "полож. текущ. инф."=w1381, "Знаки Dx всех мишеней"=w1386, "Текущ. положение лазера на мишенях 1 - 5"=w1377, "текущий id мишени"=w1387, "Выстрелов осталось по всем мишеням"=w1388, "Текущ. положение лазера на мишенях 6 - 10"=w1378) -> ("Строка параметров мишеней для сохранения"=w1373:string, "error out"=w1375:errorcluster)  [unwired: 16 in]
            n847 = call "Запись в файл (SubVI).vi"("Резервное сохр."=w1369, "error in"=w1375, "Строка параметров мишеней для сохранения"=w1373) -> ("error out"=w1374:errorcluster, "Путь к файлу"=w1370:path)  [unwired: 6 in, 1 out]
            n848 = Not A Number/Path/Refnum?(number/path/refnum=w1370) -> (NaN/Path/Refnum?=w1371:bool)
            n849 = case shown="False" w1371 {
              tunnel: w1370 -> [w1461 _]
              frame False {
                "Текущая конфигурация:" <- w1461
              }
              frame True {
              }
            }
            n850 = disable-structure shown="Enabled" {
              disable-tunnel: w1376 -> [w1475 _]
              disable-tunnel: w1374 -> [w1474 w1476]
              disable-tunnel: [w1473 w1476] -> w1372
              frame Disabled {
                n851 = call "Сохр. рисунков мишеней в файл (SubVI).vi"("error in"=w1474, "Кластер рисунков всех мишеней"=w1475) -> ("error out"=w1473:errorcluster)  [unwired: 13 in]
              }
              frame Enabled {
              }
            }
          }
          frame #1 {
            n852 = local read "флаг закрытия с сохр."() -> (w1478:bool)
            n853 = property on="Флаг резерв. сохр." class="Bool (strict)"("Value"=FALSE ("Флаг резерв. сохр.")) -> ()  [unwired: 2 in, 2 out]
            n854 = Quit LabVIEW(quit? (T)=w1478) -> ()
          }
        }
      }
      event "Сбросить конфигурацию": Value Change {
        # "Сброс текущей конфигурации"
        n855 = event-data() -> ("OldVal"=w1484:bool)  [unwired: 1 out]
        n856 = local write "Сбросить конфигурацию"(w1484) -> ()
        n857 = Two Button Dialog(message="Вы уверены, что хотите СБРОСИТЬ текущую конфигурацию?", 1:"Нет" ("F button name (\"Cancel\")"), 2:"Да" ("T button name (\"OK\")")) -> (T button?=w1480:bool)
        n858 = case shown="True" w1480 {
          frame False {
          }
          frame True {
            w1490 = T4 {"Left"=1200, "Top"=1000} ("Position")
            w1513 = i8 1 ("Выстрелов осталось M1")
            w1537 = T1 {"Название мишени"="?", "Х0_position"=400, "Y0_position"=200, "Длина, мм"=200, "Ширина, мм"=200, "Шаг перехода по горизонтали"=2.0, "Шаг перехода по вертикали"=2.0, "Выстрелов до перехода"=1, "Xo to send "=0, "Yo to send"=0} ("Параметры М1")
            w1544 = "" ("Tip Strip")
            n859 = property on="Мишень 1" class="Pict"("Visible"=FALSE) -> (error out=w1493:errorcluster)  [unwired: 2 in, 1 out]
            n860 = local write "Знак перех. dX М1"(i8 1 ("Знак перех. dX М1")) -> ()
            n861 = local write "Знак перех. dX М2"(w1513) -> ()
            n862 = local write "Знак перех. dX М3"(w1513) -> ()
            n863 = local write "Знак перех. dX М4"(w1513) -> ()
            n864 = local write "Знак перех. dX М5"(w1513) -> ()
            n865 = local write "Знак перех. dX М6"(w1513) -> ()
            n866 = local write "Знак перех. dX М7"(w1513) -> ()
            n867 = local write "Знак перех. dX М8"(w1513) -> ()
            n868 = local write "Знак перех. dX М10"(i8 1 ("Выстрелов осталось M1")) -> ()
            n869 = local write "Знак перех. dX М9"(w1513) -> ()
            n870 = local write "выстрел X М1"(u16 0 ("Выстрелов осталось M1")) -> ()
            n871 = local write "выстрел Y М1"(u16 0 ("Выстрелов осталось M2")) -> ()
            n872 = local write "выстрел X М2"(u16 0 ("Выстрелов осталось M3")) -> ()
            n873 = local write "выстрел Y М2"(u16 0 ("Выстрелов осталось M4")) -> ()
            n874 = local write "выстрел X М3"(u16 0 ("Выстрелов осталось M5")) -> ()
            n875 = local write "выстрел Y М3"(u16 0 ("Выстрелов осталось M6")) -> ()
            n876 = local write "выстрел X М4"(u16 0 ("выстрел X М9")) -> ()
            n877 = local write "выстрел Y М4"(u16 0 ("выстрел Y М9")) -> ()
            n878 = local write "выстрел X М5"(u16 0 ("выстрел X М10")) -> ()
            n879 = local write "выстрел Y М5"(u16 0 ("выстрел Y М10")) -> ()
            n880 = property on="Мишень 2" class="Pict"(error in=w1493, "Visible"=FALSE) -> (error out=w1496:errorcluster)  [unwired: 1 in, 1 out]
            n881 = local write "Осталось:"(u16 0 ("До перемотки осталось")) -> ()
            n882 = property on="Мишень 3" class="Pict"(error in=w1496, "Visible"=FALSE) -> (error out=w1498:errorcluster)  [unwired: 1 in, 1 out]
            n883 = String To Path(string="Новая конфигурация...") -> (path=w1488:path)
            n884 = local write "Текущая конфигурация:"(w1488) -> ()
            n885 = property on="Мишень 4" class="Pict"(error in=w1498, "Visible"=FALSE) -> (error out=w1500:errorcluster)  [unwired: 1 in, 1 out]
            n886 = call "Empty Picture"() -> ("empty picture"=w1512:picture)
            n887 = property on="Мишень 5" class="Pict"(error in=w1500, "Visible"=FALSE) -> (error out=w1511:errorcluster)  [unwired: 1 in, 1 out]
            n888 = local write "выстрел X М6"(u16 0 ("Выстрелов осталось M1")) -> ()
            n889 = local write "выстрел Y М6"(u16 0 ("Выстрелов осталось M2")) -> ()
            n890 = local write "выстрел X М7"(u16 0 ("Выстрелов осталось M3")) -> ()
            n891 = local write "выстрел Y М7"(u16 0 ("Выстрелов осталось M4")) -> ()
            n892 = local write "выстрел X М8"(u16 0 ("Выстрелов осталось M5")) -> ()
            n893 = local write "выстрел Y М8"(u16 0 ("Выстрелов осталось M6")) -> ()
            n894 = local write "выстрел X М9"(u16 0 ("выстрел X М9")) -> ()
            n895 = local write "выстрел Y М9"(u16 0 ("выстрел Y М9")) -> ()
            n896 = local write "выстрел X М10"(u16 0 ("выстрел X М10")) -> ()
            n897 = local write "выстрел Y М10"(u16 0 ("выстрел Y М10")) -> ()
            n898 = local write "Мишень 1"(w1512) -> ()
            n899 = local write "Мишень 2"(w1512) -> ()
            n900 = local write "Мишень 3"(w1512) -> ()
            n901 = local write "Мишень 4"(w1512) -> ()
            n902 = local write "Мишень 5"(w1512) -> ()
            n903 = local write "Мишень 6"(w1512) -> ()
            n904 = local write "Мишень 7"(w1512) -> ()
            n905 = local write "Мишень 8"(w1512) -> ()
            n906 = local write "Мишень 9"(w1512) -> ()
            n907 = local write "Мишень 10"(w1512) -> ()
            n908 = property on="Шаг вперед" class="Bool (strict)"("DisabledEnum"=T3."Disabled and Grayed Out" ("Disabled")) -> ()  [unwired: 2 in, 2 out]
            n909 = property on="Мишень 6" class="Pict"(error in=w1511, "Visible"=FALSE) -> (error out=w1510:errorcluster)  [unwired: 1 in, 1 out]
            n910 = property on="Счетчик выстрелов:" class="DigNum (strict)"("Value"=u32 0 ("Счетчик выстрелов:")) -> ()  [unwired: 2 in, 2 out]
            n911 = property on="Мишень 7" class="Pict"(error in=w1510, "Visible"=FALSE) -> (error out=w1507:errorcluster)  [unwired: 1 in, 1 out]
            n912 = local write "id мишени"(u16 0 ("id мишени")) -> ()
            n913 = local write "М1"(w1537) -> ()
            n914 = local write "М2"(w1537) -> ()
            n915 = local write "М3"(w1537) -> ()
            n916 = local write "М4"(w1537) -> ()
            n917 = local write "М5"(w1537) -> ()
            n918 = local write "М6"(w1537) -> ()
            n919 = local write "М7"(w1537) -> ()
            n920 = local write "М8"(w1537) -> ()
            n921 = local write "М9"(w1537) -> ()
            n922 = local write "М10"(w1537) -> ()
            n923 = property on="Мишень 8" class="Pict"(error in=w1507, "Visible"=FALSE) -> (error out=w1505:errorcluster)  [unwired: 1 in, 1 out]
            n924 = property on="Выстрел по мишени!" class="DigNum (strict)"("Value"=u32 0 ("Выстрел по мишени!")) -> ()  [unwired: 2 in, 2 out]
            n925 = property on="Мишень 10" class="Pict"("TipStrip"=w1544) -> ()  [unwired: 2 in, 2 out]
            n926 = property on="Мишень 9" class="Pict"("TipStrip"=w1544) -> ()  [unwired: 2 in, 2 out]
            n927 = property on="Мишень 8" class="Pict"("TipStrip"=w1544) -> ()  [unwired: 2 in, 2 out]
            n928 = property on="Мишень 7" class="Pict"("TipStrip"=w1544) -> ()  [unwired: 2 in, 2 out]
            n929 = property on="Мишень 6" class="Pict"("TipStrip"=w1544) -> ()  [unwired: 2 in, 2 out]
            n930 = property on="Мишень 5" class="Pict"("TipStrip"=w1544) -> ()  [unwired: 2 in, 2 out]
            n931 = property on="Мишень 4" class="Pict"("TipStrip"=w1544) -> ()  [unwired: 2 in, 2 out]
            n932 = property on="Мишень 3" class="Pict"("TipStrip"=w1544) -> ()  [unwired: 2 in, 2 out]
            n933 = property on="Мишень 2" class="Pict"("TipStrip"=w1544) -> ()  [unwired: 2 in, 2 out]
            n934 = property on="Мишень 1" class="Pict"("TipStrip"=w1544) -> ()  [unwired: 2 in, 2 out]
            n935 = property on="Мишень 9" class="Pict"(error in=w1505, "Visible"=FALSE) -> (error out=w1503:errorcluster)  [unwired: 1 in, 1 out]
            n936 = property on="Мишень 10" class="Pict"(error in=w1503, "Visible"=FALSE) -> ()  [unwired: 1 in, 2 out]
            n937 = property on="Счетчик мишеней" class="DigNum (strict)"("Value"=u32 0 ("Выстрел по мишени!")) -> ()  [unwired: 2 in, 2 out]
            n938 = Bundle("Счетчик мишеней"=u32 200, "Счетчик мишеней"=u32 200) -> (w1543:T16)  [unwired: 1 in]
            n939 = Bundle("Счетчик мишеней"=400, "Счетчик мишеней"=200) -> (w1542:T17)  [unwired: 1 in]
            n940 = property on="Мишень 1" class="Pict"("Draw Area Size"=w1543) -> ()  [unwired: 2 in, 2 out]
            n941 = property on="Мишень 2" class="Pict"("Draw Area Size"=w1543) -> ()  [unwired: 2 in, 2 out]
            n942 = property on="Мишень 1" class="Pict"("Position"=w1542) -> ()  [unwired: 2 in, 2 out]
            n943 = property on="Мишень 2" class="Pict"("Position"=w1542) -> ()  [unwired: 2 in, 2 out]
            n944 = property on="XY лазера увожу за экран при вкл" class="Bool (strict)"("Position"=w1490) -> ()  [unwired: 2 in, 2 out]
            n945 = property on="Мишень 3" class="Pict"("Position"=w1542) -> ()  [unwired: 2 in, 2 out]
            n946 = property on="Мишень 4" class="Pict"("Position"=w1542) -> ()  [unwired: 2 in, 2 out]
            n947 = property on="Мишень 3" class="Pict"("Draw Area Size"=w1543) -> ()  [unwired: 2 in, 2 out]
            n948 = property on="Мишень 4" class="Pict"("Draw Area Size"=w1543) -> ()  [unwired: 2 in, 2 out]
            n949 = property on="Мишень 5" class="Pict"("Position"=w1542) -> ()  [unwired: 2 in, 2 out]
            n950 = property on="Мишень 6" class="Pict"("Position"=w1542) -> ()  [unwired: 2 in, 2 out]
            n951 = property on="Мишень 5" class="Pict"("Draw Area Size"=w1543) -> ()  [unwired: 2 in, 2 out]
            n952 = property on="Мишень 6" class="Pict"("Draw Area Size"=w1543) -> ()  [unwired: 2 in, 2 out]
            n953 = property on="текущ. инфо" class="Bool (strict)"("Position"=w1490) -> ()  [unwired: 2 in, 2 out]
            n954 = property on="Мишень 7" class="Pict"("Position"=w1542) -> ()  [unwired: 2 in, 2 out]
            n955 = property on="Мишень 8" class="Pict"("Position"=w1542) -> ()  [unwired: 2 in, 2 out]
            n956 = property on="Мишень 7" class="Pict"("Draw Area Size"=w1543) -> ()  [unwired: 2 in, 2 out]
            n957 = property on="Мишень 8" class="Pict"("Draw Area Size"=w1543) -> ()  [unwired: 2 in, 2 out]
            n958 = property on="Мишень 9" class="Pict"("Position"=w1542) -> ()  [unwired: 2 in, 2 out]
            n959 = property on="Мишень 10" class="Pict"("Position"=w1542) -> ()  [unwired: 2 in, 2 out]
            n960 = property on="Мишень 9" class="Pict"("Draw Area Size"=w1543) -> ()  [unwired: 2 in, 2 out]
            n961 = property on="Мишень 10" class="Pict"("Draw Area Size"=w1543) -> ()  [unwired: 2 in, 2 out]
          }
        }
      }
      event "Загрузить настройки": Value Change {
        # "Восстановление конфигурации из файла"
        n962 = event-data() -> ("OldVal"=w1553:bool)  [unwired: 1 out]
        n963 = property on="Загрузить \nнастройки" class="Bool (strict)"(error in=w1552, "Value"=w1553) -> (error out=w1549:errorcluster)  [unwired: 1 in, 1 out]
        n964 = Read from Text File(prompt (Open existing file)="Укажите  файл конфигурации...", error in=w1549) -> (refnum out=w1546:refnum<file>, text=w1550:string, cancelled=w1545:bool, error out=w1548:errorcluster)  [unwired: 2 in]
        n965 = case shown="False" w1545 {
          tunnel: w1550 -> [w1641 _]
          tunnel: w1548 -> [w1564 w1651]
          tunnel: [w1563 w1651] -> w1547
          tunnel: w1546 -> [w1560 _]
          frame False {
            n966 = control-ref of="Мишень 1"() -> (w1639:refnum<vi>)
            n967 = control-ref of="Мишень 2"() -> (w1638:refnum<vi>)
            n968 = control-ref of="Мишень 3"() -> (w1637:refnum<vi>)
            n969 = control-ref of="Мишень 4"() -> (w1636:refnum<vi>)
            n970 = control-ref of="Мишень 5"() -> (w1635:refnum<vi>)
            n971 = control-ref of="Мишень 6"() -> (w1634:refnum<vi>)
            n972 = control-ref of="Мишень 7"() -> (w1633:refnum<vi>)
            n973 = control-ref of="Мишень 8"() -> (w1632:refnum<vi>)
            n974 = control-ref of="Мишень 9"() -> (w1631:refnum<vi>)
            n975 = control-ref of="Мишень 10"() -> (w1630:refnum<vi>)
            n976 = Refnum to Path(1:w1560) -> (0:w1559:path)
            n977 = Bundle("Мишень 1"=w1639, "Мишень 2"=w1638, "Мишень 3"=w1637, "Мишень 4"=w1636, "Мишень 5"=w1635, "Мишень 6"=w1634, "Мишень 7"=w1633, "Мишень 8"=w1632, "Мишень 9"=w1631, "Мишень 10"=w1630) -> (w1629:T18)  [unwired: 1 in]
            n978 = call "Строку в параметры мишени (SubVI).vi"("Параметры мишени строка"=w1641) -> ("Кластер параметров мишени"=w1576:T1, "Остаток строки параметров"=w1642:string)  [unwired: 13 in]
            n979 = call "Строку в параметры мишени (SubVI).vi"("Параметры мишени строка"=w1642) -> ("Кластер параметров мишени"=w1575:T1, "Остаток строки параметров"=w1650:string)  [unwired: 13 in]
            n980 = call "Строку в параметры мишени (SubVI).vi"("Параметры мишени строка"=w1650) -> ("Кластер параметров мишени"=w1574:T1, "Остаток строки параметров"=w1648:string)  [unwired: 13 in]
            n981 = call "Строку в параметры мишени (SubVI).vi"("Параметры мишени строка"=w1648) -> ("Кластер параметров мишени"=w1573:T1, "Остаток строки параметров"=w1649:string)  [unwired: 13 in]
            n982 = call "Строку в параметры мишени (SubVI).vi"("Параметры мишени строка"=w1649) -> ("Кластер параметров мишени"=w1572:T1, "Остаток строки параметров"=w1644:string)  [unwired: 13 in]
            n983 = call "Строку в параметры мишени (SubVI).vi"("Параметры мишени строка"=w1644) -> ("Кластер параметров мишени"=w1571:T1, "Остаток строки параметров"=w1645:string)  [unwired: 13 in]
            n984 = call "Строку в параметры мишени (SubVI).vi"("Параметры мишени строка"=w1645) -> ("Кластер параметров мишени"=w1570:T1, "Остаток строки параметров"=w1647:string)  [unwired: 13 in]
            n985 = call "Строку в параметры мишени (SubVI).vi"("Параметры мишени строка"=w1647) -> ("Кластер параметров мишени"=w1569:T1, "Остаток строки параметров"=w1646:string)  [unwired: 13 in]
            n986 = call "Строку в параметры мишени (SubVI).vi"("Параметры мишени строка"=w1646) -> ("Кластер параметров мишени"=w1568:T1, "Остаток строки параметров"=w1643:string)  [unwired: 13 in]
            n987 = call "Строку в параметры мишени (SubVI).vi"("Параметры мишени строка"=w1643) -> ("Кластер параметров мишени"=w1567:T1, "Остаток строки параметров"=w1640:string)  [unwired: 13 in]
            n988 = call "Упр. видимостью мишеней (SubVI).vi"("Строка параметров видимости мишеней"=w1640, "Кластер reference"=w1629) -> ("Кластер reference out"=w1561:T19, "Остаток строки"=w1628:string, "Кол-во видимых мишеней"=w1562:u8)  [unwired: 11 in]
            n989 = call "Строку в числовые данные мишеней (SubVI).vi"("Строка с числовыми параметрами мишени"=w1628) -> ("Остаток строки"=w1615:string, "Кластер числовых параметров мишеней"=w1627:T20)  [unwired: 25 in]
            n990 = call "Строку в числовые данные мишеней (SubVI).vi"("Строка с числовыми параметрами мишени"=w1615) -> ("Остаток строки"=w1604:string, "Кластер числовых параметров мишеней"=w1616:T20)  [unwired: 25 in]
            n991 = call "Строку в числовые данные мишеней (SubVI).vi"("Строка с числовыми параметрами мишени"=w1604) -> ("Остаток строки"=w1592:string, "Кластер числовых параметров мишеней"=w1593:T20)  [unwired: 25 in]
            n992 = call "Строка параметров в I8 (SubVI).vi"("Строка чисел параметров мишеней"=w1592) -> ("Остаток строки"=w1579:string, "Кластер чисел типа I8"=w1591:T21)  [unwired: 17 in]
            n993 = Match Pattern(string=w1579, regular expression="-----") -> (after substring=w1577:string)  [unwired: 1 in, 3 out]
            n994 = local write "Текущая конфигурация:"(w1559) -> ()
            n995 = local write "Счетчик мишеней"(w1562) -> ()
            n996 = Decimal String To Number(string=w1577, default (0L)=u16 0 ("default (0 I32)")) -> (number=w1554:u16)  [unwired: 1 in, 1 out]
            n997 = property on="id мишени" class="DigNum (strict)"("Val(Sgnl)"=w1554) -> ()  [unwired: 2 in, 2 out]
            n998 = Unbundle(w1627) -> ("1"=w1626:u16, "2"=w1625:u16, "3"=w1624:u16, "4"=w1623:u16, "5"=w1622:u16, "6"=w1621:u16, "7"=w1620:u16, "8"=w1619:u16, "9"=w1618:u16, "10"=w1617:u16)
            n999 = local write "М1"(w1576) -> ()
            n1000 = local write "М2"(w1575) -> ()
            n1001 = local write "М3"(w1574) -> ()
            n1002 = local write "М4"(w1573) -> ()
            n1003 = local write "М5"(w1572) -> ()
            n1004 = local write "М6"(w1571) -> ()
            n1005 = local write "М7"(w1570) -> ()
            n1006 = local write "М8"(w1569) -> ()
            n1007 = local write "М9"(w1568) -> ()
            n1008 = local write "М10"(w1567) -> ()
            n1009 = call "Строку в коор. выстрела лазера (SubVI).vi"("Строка числовых параметров мишеней"=w1577) -> ("Положение XY лазера"=w1558:cluster{i32, i32}, "Положение информации о выстреле"=w1557:cluster{i32, i32})  [unwired: 25 in]
            n1010 = local write "Выстрелов осталось M1"(w1626) -> ()
            n1011 = local write "Выстрелов осталось M2"(w1625) -> ()
            n1012 = local write "Выстрелов осталось M3"(w1624) -> ()
            n1013 = local write "Выстрелов осталось M4"(w1623) -> ()
            n1014 = local write "Выстрелов осталось M5"(w1622) -> ()
            n1015 = local write "Выстрелов осталось M6"(w1621) -> ()
            n1016 = local write "Выстрелов осталось M7"(w1620) -> ()
            n1017 = local write "Выстрелов осталось M8"(w1619) -> ()
            n1018 = local write "Выстрелов осталось M9"(w1618) -> ()
            n1019 = local write "Выстрелов осталось M10"(w1617) -> ()
            n1020 = property on="XY лазера" class="Bool (strict)"("Position"=w1558) -> (error out=w1555:errorcluster)  [unwired: 2 in, 1 out]
            n1021 = Bundle("Кластер параметров мишени"=w1576, "Кластер параметров мишени"=w1575, "Кластер параметров мишени"=w1574, "Кластер параметров мишени"=w1573, "Кластер параметров мишени"=w1572, "Кластер параметров мишени"=w1571, "Кластер параметров мишени"=w1570, "Кластер параметров мишени"=w1569, "Кластер параметров мишени"=w1568, "Кластер параметров мишени"=w1567) -> (w1566:T22)  [unwired: 1 in]
            n1022 = property on="текущ. инфо" class="Bool (strict)"(error in=w1555, "Position"=w1557) -> (error out=w1556:errorcluster)  [unwired: 1 in, 1 out]
            n1023 = call "Восстановление мишеней (SubVI).vi"("error in"=w1564, "Параметры всех мишеней"=w1566, "Кластер reference"=w1561) -> ("error out"=w1565:errorcluster)  [unwired: 12 in]
            n1024 = Unbundle(w1616) -> ("1"=w1614:u16, "2"=w1613:u16, "3"=w1612:u16, "4"=w1611:u16, "5"=w1610:u16, "6"=w1609:u16, "7"=w1608:u16, "8"=w1607:u16, "9"=w1606:u16, "10"=w1605:u16)
            n1025 = local write "выстрел X М1"(w1614) -> ()
            n1026 = local write "выстрел Y М1"(w1613) -> ()
            n1027 = local write "выстрел X М2"(w1612) -> ()
            n1028 = local write "выстрел Y М2"(w1611) -> ()
            n1029 = local write "выстрел X М3"(w1610) -> ()
            n1030 = local write "выстрел Y М3"(w1609) -> ()
            n1031 = local write "выстрел X М4"(w1608) -> ()
            n1032 = local write "выстрел Y М4"(w1607) -> ()
            n1033 = local write "выстрел X М5"(w1606) -> ()
            n1034 = local write "выстрел Y М5"(w1605) -> ()
            n1035 = Unbundle(w1593) -> ("1"=w1594:u16, "2"=w1595:u16, "3"=w1596:u16, "4"=w1597:u16, "5"=w1598:u16, "6"=w1599:u16, "7"=w1600:u16, "8"=w1601:u16, "9"=w1602:u16, "10"=w1603:u16)
            n1036 = local write "выстрел X М6"(w1594) -> ()
            n1037 = local write "выстрел Y М6"(w1595) -> ()
            n1038 = local write "выстрел X М7"(w1596) -> ()
            n1039 = local write "выстрел Y М7"(w1597) -> ()
            n1040 = local write "выстрел X М8"(w1598) -> ()
            n1041 = local write "выстрел Y М8"(w1599) -> ()
            n1042 = local write "выстрел X М9"(w1600) -> ()
            n1043 = local write "выстрел Y М9"(w1601) -> ()
            n1044 = local write "выстрел X М10"(w1602) -> ()
            n1045 = local write "выстрел Y М10"(w1603) -> ()
            n1046 = Unbundle(w1591) -> ("default value 1"=w1590:i8, "default value 1"=w1589:i8, "default value 1"=w1588:i8, "default value 1"=w1587:i8, "default value 1"=w1586:i8, "default value 1"=w1585:i8, "default value 1"=w1584:i8, "default value 1"=w1583:i8, "default value 1"=w1582:i8, "default value 1"=w1581:i8)
            n1047 = local write "Знак перех. dX М1"(w1590) -> ()
            n1048 = local write "Знак перех. dX М2"(w1589) -> ()
            n1049 = local write "Знак перех. dX М3"(w1588) -> ()
            n1050 = local write "Знак перех. dX М4"(w1587) -> ()
            n1051 = local write "Знак перех. dX М5"(w1586) -> ()
            n1052 = local write "Знак перех. dX М6"(w1585) -> ()
            n1053 = local write "Знак перех. dX М7"(w1584) -> ()
            n1054 = local write "Знак перех. dX М8"(w1583) -> ()
            n1055 = local write "Знак перех. dX М10"(w1581) -> ()
            n1056 = local write "Знак перех. dX М9"(w1582) -> ()
            n1057 = Merge Errors(w1565, w1556) -> (w1563:errorcluster)
          }
          frame True {
          }
        }
      }
      event Panel Close? {
        # "Защита и сохранение при закрытии программы"
        n1058 = event-data() -> ()  [unwired: 2 out]
        n1059 = call <vilib>:"Three Button Dialog.vi"("Allow user to close window? (TRUE)"=TRUE, "Right Button Text (\"Cancel\")"="Отмена" ("message"), "Center Button Text (\"No\")"="Закрыть программу \nбез сохранений" ("message"), "Left Button Text (\"Yes\")"="Сохранить текущую конфигурацию \nи закрыть программу" ("message"), "message"="Вы уверены, что хотите закрыть программу?") -> ("Which Button?"=w1658:T23)  [unwired: 6 in]
        n1060 = case shown="\"Left Button\"" w1658 {
          tunnel: [w1660 FALSE ("Discard?") TRUE ("Value (Signaling)") TRUE ("Discard?")] -> w1655
          frame "Left Button" {
            n1061 = flat-sequence {
              tunnel: [w1663] -> w1662
              tunnel: w1662 -> [w1667]
              tunnel: [w1667] -> w1661
              tunnel: [TRUE ("Discard?")] -> w1659
              tunnel: w1661 -> [w1670]
              tunnel: [w1669] -> w1660
              tunnel: w1659 -> [w1669]
              frame #0 {
                n1062 = local read "TCP con ID"() -> (w1664:refnum<k5>)
                n1063 = TCP Close Connection(connection ID=w1664) -> (error out=w1663:errorcluster)  [unwired: 1 in, 2 out]
              }
              frame #1 {
                n1064 = property on="Конфигурация сохранена" class="Bool (strict)"("Val(Sgnl)"=TRUE ("Value (Signaling)")) -> ()  [unwired: 2 in, 2 out]
                "флаг закрытия с сохр." <- TRUE ("флаг закрытия")
              }
              frame #2 {
                w1674 = FALSE ("Запись в файл")
                w1673 = TRUE ("Tool Bar:Visible")
                n1065 = local write "Соединение"(w1674) -> ()
                n1066 = property on="кнопки запуска, стоп и тд" class="VI"(error in=w1670, "TB.Visible"=w1673) -> (error out=w1672:errorcluster)  [unwired: 1 in, 1 out]
                n1067 = local write "con err"(w1673) -> ()
                n1068 = local write "Соединение с блоком"(w1674) -> ()
                n1069 = call <vilib>:"General Error Handler.vi"("type of dialog (OK msg:1)"=u32 0 ("milliseconds to wait"), "error in (no error)"=w1672) -> ()  [unwired: 14 out]
              }
            }
          }
          frame "Center Button" {
            w1680 = FALSE ("Запись в файл")
            w1679 = TRUE ("Tool Bar:Visible")
            n1070 = local read "TCP con ID"() -> (w1681:refnum<k5>)
            n1071 = TCP Close Connection(connection ID=w1681) -> (error out=w1675:errorcluster)  [unwired: 1 in, 2 out]
            n1072 = flat-sequence {
              tunnel: [w1683] -> w1676
              tunnel: w1675 -> [w1683]
              frame #0 {
                n1073 = Wait (ms)(milliseconds to wait=u32 200) -> ()  [unwired: 1 out]
              }
            }
            n1074 = local write "Соединение"(w1680) -> ()
            n1075 = property on="кнопки запуска, стоп и тд" class="VI"(error in=w1676, "TB.Visible"=w1679) -> (error out=w1678:errorcluster)  [unwired: 1 in, 1 out]
            n1076 = local write "con err"(w1679) -> ()
            n1077 = local write "Соединение с блоком"(w1680) -> ()
            n1078 = call <vilib>:"General Error Handler.vi"("type of dialog (OK msg:1)"=u32 0 ("milliseconds to wait"), "error in (no error)"=w1678) -> ()  [unwired: 14 out]
          }
          frame "Right Button" {
            n1079 = local write "флаг закрытия с сохр."(FALSE ("флаг закрытия с сохр.")) -> ()
          }
          frame "Window Close" {
          }
        }
        n1080 = event-data("Discard?"=w1655) -> ()  [unwired: 1 in, 1 out]
      }
    }
    n1081 = call <vilib>:"General Error Handler.vi"("type of dialog (OK msg:1)"=u8 0, "error in (no error)"=w97) -> ("error out"=w96:errorcluster)  [unwired: 13 out]
  }
  n1082 = property class="VI"(error in=w39, "Front Panel.Resizeable"=TRUE ("Front Panel Window:Resizable")) -> (error out=w38:errorcluster)  [unwired: 1 in, 1 out]
  n1083 = property on="Мишень 7" class="Pict"(error in=w17, "Visible"=FALSE) -> (error out=w20:errorcluster)  [unwired: 1 in, 1 out]
  n1084 = while {
    stop <- FALSE stop-if-true
    # "Связь с блоком"
    n1085 = TCP Open Connection(address="IP-адрес", remote port or service name="порт", timeout ms (60000)=2000) -> (connection ID=w1700:refnum<k5>, error out=w1701:errorcluster)  [unwired: 1 in, 1 out]
    "TCP con ID" <- w1700
    n1086 = disable-structure shown="Enabled" {
      disable-tunnel: w1701 -> [w1721 w1725]
      disable-tunnel: w1700 -> [w1720 w1726]
      disable-tunnel: [w1719 w1725] -> w1694
      disable-tunnel: [w1718 w1726] -> w1693
      frame Disabled {
        n1087 = flat-sequence {
          tunnel: w1721 -> [w1723]
          tunnel: [w1723] -> w1719
          tunnel: [w1722] -> w1718
          tunnel: w1720 -> [w1722]
          frame #0 {
            n1088 = Wait (ms)(milliseconds to wait=u32 1) -> ()  [unwired: 1 out]
          }
        }
      }
      frame Enabled {
      }
    }
    n1089 = case "Запрос на команду от блока" shown="No Error" w1694 {
      selector: w1694 -> [w1744 w1746]
      tunnel: [w1743 w1746] -> w1691
      tunnel: w1693 -> [w1742 w1745]
      tunnel: [w1741 w1745] -> w1692
      frame No Error {
        n1090 = TCP Write(connection ID=w1742, data in="Ready", error in (no error)=w1744, 9:2000 ("timeout ms (25000)")) -> (connection ID out=w1741:refnum<k5>, error out=w1743:errorcluster)  [unwired: 1 out]
      }
      frame Error {
      }
    }
    n1091 = case "чтение команды блока" shown="No Error" w1691 {
      selector: w1691 -> [w1727 w1738]
      tunnel: [w1733 _] -> w1711
      tunnel: [w1732 w1738] -> w1699
      tunnel: [w1731 w1737] -> w1697
      tunnel: w1692 -> [w1730 w1737]
      frame No Error {
        n1092 = flat-sequence {
          tunnel: w1727 -> [w1735]
          tunnel: [w1735] -> w1728
          tunnel: [w1734] -> w1729
          tunnel: w1730 -> [w1734]
          frame #0 {
            n1093 = Wait (ms)(milliseconds to wait=u32 1) -> ()  [unwired: 1 out]
          }
        }
        n1094 = call "TCP Data read (SubVI).vi"("error in (no error)"=w1728, "TCP Network Connection in"=w1729) -> ("error out"=w1732:errorcluster, "Read data"=w1733:string, "TCP Network Connection out"=w1731:refnum<k5>)  [unwired: 1 in, 6 out]
      }
      frame Error {
      }
    }
    n1095 = case "обновление данных программы" shown="No Error" w1699 {
      selector: w1699 -> [w1748 w1752]
      tunnel: w1711 -> [w1750 _]
      tunnel: [w1749 w1752] -> w1709
      tunnel: [w1747 w1751] -> w1698
      tunnel: w1697 -> [w1747 w1751]
      frame No Error {
        n1096 = property on="TCP read data" class="Str"(error in=w1748, "Val(Sgnl)"=w1750) -> (error out=w1749:errorcluster)  [unwired: 1 in, 1 out]
      }
      frame Error {
      }
    }
    n1097 = TCP Close Connection(connection ID=w1698, error in (no error)=w1709) -> (error out=w1690:errorcluster)  [unwired: 2 out]
    n1098 = case shown="No Error" w1690 {
      selector: w1690 -> [w1715 w1717]
      tunnel: [w1715 w1717] -> w1689
      tunnel: [u32 100 ("milliseconds to wait") u32 500 ("milliseconds to wait")] -> w1688
      frame No Error {
      }
      frame Error {
      }
    }
    n1099 = Wait (ms)(milliseconds to wait=w1688) -> ()  [unwired: 1 out]
    n1100 = Unbundle By Name(w1689) -> ("status"=w1695:bool)
    "con err" <- w1695
    n1101 = Not(x=w1695) -> (.not. x?=w1696:bool)
    "Соединение с блоком" <- w1696
    "Соединение" <- w1696
    n1102 = local write "Connect 2"(w1696) -> ()
    n1103 = call <vilib>:"General Error Handler.vi"("type of dialog (OK msg:1)"=u8 0, "error in (no error)"=w1689) -> ("code out"=→"code out":i32, "source out"=→"TCP error source":string)  [unwired: 12 out]
    n1104 = Select(t="Ошибка соединения с блоком..." ("Caption.Text"), s=w1695, f="Связь установлена" ("Caption.Text")) -> (s? t:f=w1706:string)
    n1105 = property on="Con.err.text" class="Bool (strict)"("Caption.Text"=w1706) -> ()  [unwired: 2 in, 2 out]
  }
  n1106 = property on="Мишень 8" class="Pict"(error in=w20, "Visible"=FALSE) -> (error out=w22:errorcluster)  [unwired: 1 in, 1 out]
  n1107 = property on="Мишень 9" class="Pict"(error in=w22, "Visible"=FALSE) -> (error out=w24:errorcluster)  [unwired: 1 in, 1 out]
  n1108 = property class="VI"(error in=w38, "Front Panel.ShowMenuBar"=FALSE ("Front Panel Window:Show Menu Bar")) -> ()  [unwired: 1 in, 2 out]
  n1109 = property on="Мишень 10" class="Pict"(error in=w24, "Visible"=FALSE) -> ()  [unwired: 1 in, 2 out]
  n1110 = event shown="[0] \"stop\": Value Change" {
    selector: _ -> [_]
    dyn-events: _ -> [_]
    timeout: _ -> [_]
    event "stop": Value Change {
      n1111 = event-data() -> ()  [unwired: 2 out]
      n1112 = flat-sequence {
        tunnel: [w1755] -> w1754
        tunnel: w1754 -> [w1758]
        tunnel: [w1758] -> w1753
        tunnel: w1753 -> [w1759]
        frame #0 {
          n1113 = local read "TCP con ID"() -> (w1756:refnum<k5>)
          n1114 = TCP Close Connection(connection ID=w1756) -> (error out=w1755:errorcluster)  [unwired: 1 in, 2 out]
        }
        frame #1 {
          n1115 = Wait (ms)(milliseconds to wait=u32 200) -> ()  [unwired: 1 out]
        }
        frame #2 {
          w1763 = FALSE ("Запись в файл")
          w1762 = TRUE ("Tool Bar:Visible")
          n1116 = local write "Соединение"(w1763) -> ()
          n1117 = property on="кнопки запуска, стоп и тд" class="VI"(error in=w1759, "TB.Visible"=w1762) -> (error out=w1761:errorcluster)  [unwired: 1 in, 1 out]
          n1118 = local write "con err"(w1762) -> ()
          n1119 = local write "Соединение с блоком"(w1763) -> ()
          n1120 = call <vilib>:"General Error Handler.vi"("type of dialog (OK msg:1)"=u32 0 ("milliseconds to wait"), "error in (no error)"=w1761) -> ()  [unwired: 14 out]
        }
        frame #3 {
          n1121 = Stop(stop? (T)=TRUE) -> ()
        }
      }
    }
  }
  n1122 = disable-structure shown="Enabled" {
    frame Enabled {
      n1123 = property on="Счетчик выстрелов:" class="DigNum (strict)"("Value"=u32 0 ("Счетчик выстрелов:")) -> ()  [unwired: 2 in, 2 out]
    }
    frame Disabled {
    }
  }
  n1124 = property on="DownButton" class="Bool (strict)"("DisabledEnum"=T3."Enabled" ("Disabled")) -> ()  [unwired: 2 in, 2 out]
  n1125 = property on="Счетчик выстрелов:" class="DigNum (strict)"("Value"=0.0 ("Счетчик выстрелов:")) -> (error out=w56:errorcluster)  [unwired: 2 in, 1 out]
  n1126 = property on="XY лазера" class="Bool (strict)"("Visible"=TRUE) -> ()  [unwired: 2 in, 2 out]
  n1127 = property on="XY лазера увожу за экран при вкл" class="Bool (strict)"("Position"=w49) -> ()  [unwired: 2 in, 2 out]
  n1128 = property on="текущ. инфо" class="Bool (strict)"("Caption.TextColor"=u32 16711680 ("цвет")) -> ()  [unwired: 2 in, 2 out]
  n1129 = property on="Выстрел по мишени!" class="DigNum (strict)"(error in=w56, "Value"=u32 0 ("Выстрел по мишени!")) -> ()  [unwired: 1 in, 2 out]
  n1130 = property on="текущ. инфо" class="Bool (strict)"("Position"=w49) -> ()  [unwired: 2 in, 2 out]
  n1131 = while {
    stop <- FALSE stop-if-true
    # "Сохранение параметров каждые 10 сек"
    n1132 = property on="Мишень 1" class="Pict"() -> ("Visible"=w1778:bool)  [unwired: 2 in, 2 out]
    n1133 = property on="Мишень 8" class="Pict"() -> ("Visible"=w1777:bool)  [unwired: 2 in, 2 out]
    n1134 = property on="Мишень 10" class="Pict"() -> ("Visible"=w1776:bool)  [unwired: 2 in, 2 out]
    n1135 = property on="Мишень 9" class="Pict"() -> ("Visible"=w1775:bool)  [unwired: 2 in, 2 out]
    n1136 = property on="Мишень 2" class="Pict"() -> ("Visible"=w1774:bool)  [unwired: 2 in, 2 out]
    n1137 = property on="Мишень 3" class="Pict"() -> ("Visible"=w1773:bool)  [unwired: 2 in, 2 out]
    n1138 = property on="Мишень 4" class="Pict"() -> ("Visible"=w1772:bool)  [unwired: 2 in, 2 out]
    n1139 = property on="Мишень 5" class="Pict"() -> ("Visible"=w1771:bool)  [unwired: 2 in, 2 out]
    n1140 = property on="Мишень 6" class="Pict"() -> ("Visible"=w1770:bool)  [unwired: 2 in, 2 out]
    n1141 = property on="Мишень 7" class="Pict"() -> ("Visible"=w1767:bool)  [unwired: 2 in, 2 out]
    n1142 = Compound Arithmetic op=OR(w1778, w1767, w1777, w1776, w1775, w1774, w1773, w1772, w1771, w1770) -> (w1768:bool)
    n1143 = case shown="True" w1768 {
      frame False {
      }
      frame True {
        n1144 = property on="Конфигурация сохранена" class="Bool (strict)"("Val(Sgnl)"=TRUE ("Value (Signaling)")) -> ()  [unwired: 2 in, 2 out]
        "Флаг резерв. сохр." <- TRUE ("Флаг резерв. сохр.")
      }
    }
    n1145 = Wait Until Next ms Multiple(millisecond multiple=u32 10000) -> ()  [unwired: 1 out]
  }
  n1146 = property on="Соединение с блоком" class="Bool (strict)"("Value"=FALSE ("Connected")) -> (error out=w37:errorcluster)  [unwired: 2 in, 1 out]
  n1147 = call-poly <vilib>:"Close Input Device.vi"("error in (no error)"=w50, "device ID"=w48) -> ()  [unwired: 9 out]
  n1148 = disable-structure shown="Enabled" {
    disable-tunnel: [w1782] -> w26
    disable-tunnel: w37 -> [w1782]
    frame Enabled {
      n1149 = local write "флаг закрытия с сохр."(FALSE ("флаг закрытия с сохр.")) -> ()
      n1150 = local write "stop"(FALSE ("Boolean")) -> ()
    }
  }
  n1151 = property on="Счетчик мишеней" class="DigNum (strict)"(error in=w26, "Value"=u16 0 ("Счетчик мишеней")) -> ()  [unwired: 1 in, 2 out]
  n1152 = Bundle("Счетчик мишеней"=u32 200, "Счетчик мишеней"=u32 200) -> (w9:T16)  [unwired: 1 in]
  n1153 = Bundle("Счетчик мишеней"=400, "Счетчик мишеней"=200) -> (w10:T17)  [unwired: 1 in]
  n1154 = property on="Мишень 1" class="Pict"("Draw Area Size"=w9) -> ()  [unwired: 2 in, 2 out]
  n1155 = property on="Мишень 2" class="Pict"("Draw Area Size"=w9) -> ()  [unwired: 2 in, 2 out]
  n1156 = property on="Мишень 1" class="Pict"("Position"=w10) -> ()  [unwired: 2 in, 2 out]
  n1157 = property on="Мишень 2" class="Pict"("Position"=w10) -> ()  [unwired: 2 in, 2 out]
  n1158 = property on="Мишень 3" class="Pict"("Position"=w10) -> ()  [unwired: 2 in, 2 out]
  n1159 = property on="Мишень 4" class="Pict"("Position"=w10) -> ()  [unwired: 2 in, 2 out]
  n1160 = property on="Мишень 3" class="Pict"("Draw Area Size"=w9) -> ()  [unwired: 2 in, 2 out]
  n1161 = property on="Мишень 4" class="Pict"("Draw Area Size"=w9) -> ()  [unwired: 2 in, 2 out]
  n1162 = property on="Мишень 10" class="Pict"("TipStrip"=w8) -> ()  [unwired: 2 in, 2 out]
  n1163 = property on="Мишень 9" class="Pict"("TipStrip"=w8) -> ()  [unwired: 2 in, 2 out]
  n1164 = property on="Мишень 8" class="Pict"("TipStrip"=w8) -> ()  [unwired: 2 in, 2 out]
  n1165 = property on="Мишень 7" class="Pict"("TipStrip"=w8) -> ()  [unwired: 2 in, 2 out]
  n1166 = property on="Мишень 6" class="Pict"("TipStrip"=w8) -> ()  [unwired: 2 in, 2 out]
  n1167 = property on="Мишень 5" class="Pict"("TipStrip"=w8) -> ()  [unwired: 2 in, 2 out]
  n1168 = property on="Мишень 4" class="Pict"("TipStrip"=w8) -> ()  [unwired: 2 in, 2 out]
  n1169 = property on="Мишень 3" class="Pict"("TipStrip"=w8) -> ()  [unwired: 2 in, 2 out]
  n1170 = property on="Мишень 2" class="Pict"("TipStrip"=w8) -> ()  [unwired: 2 in, 2 out]
  n1171 = property on="Мишень 1" class="Pict"("TipStrip"=w8) -> ()  [unwired: 2 in, 2 out]
  n1172 = property on="Мишень 5" class="Pict"("Position"=w10) -> ()  [unwired: 2 in, 2 out]
  n1173 = property on="Мишень 6" class="Pict"("Position"=w10) -> ()  [unwired: 2 in, 2 out]
  n1174 = property on="Мишень 5" class="Pict"("Draw Area Size"=w9) -> ()  [unwired: 2 in, 2 out]
  n1175 = property on="Мишень 6" class="Pict"("Draw Area Size"=w9) -> ()  [unwired: 2 in, 2 out]
  n1176 = property on="Мишень 7" class="Pict"("Position"=w10) -> ()  [unwired: 2 in, 2 out]
  n1177 = property on="Мишень 8" class="Pict"("Position"=w10) -> ()  [unwired: 2 in, 2 out]
  n1178 = property on="Мишень 7" class="Pict"("Draw Area Size"=w9) -> ()  [unwired: 2 in, 2 out]
  n1179 = property on="Мишень 8" class="Pict"("Draw Area Size"=w9) -> ()  [unwired: 2 in, 2 out]
  n1180 = property on="Мишень 9" class="Pict"("Position"=w10) -> ()  [unwired: 2 in, 2 out]
  n1181 = property on="Мишень 10" class="Pict"("Position"=w10) -> ()  [unwired: 2 in, 2 out]
  n1182 = property on="Мишень 9" class="Pict"("Draw Area Size"=w9) -> ()  [unwired: 2 in, 2 out]
  n1183 = property on="Мишень 10" class="Pict"("Draw Area Size"=w9) -> ()  [unwired: 2 in, 2 out]
  "Осталось:" <- u16 0 ("До перемотки осталось")
